vi "Position_TOTAL_R25.vi"(5 "Distance Between \nCameras  (*unit)":sgl=2.25) -> (12 "dX, dY\nLeft Cam":cluster{"X":sgl[], "Y":sgl[]}={"X"=[-1.0065897, 0.099401906, 1.1628555, 2.2500029, 0.0], "Y"=[10.716516, 10.801518, 10.883252, 10.9668045, 0.0]}, 13 "Position Valid":bool=TRUE, 14 "Left Camera Real Coordinates":cluster{"X":sgl, "Y":sgl}={"X"=10.842023, "Y"=1.3735824}, 16 "dX, dY\nRight Cam":cluster{"X":sgl[], "Y":sgl[]}={"X"=[-2.8840373, -1.7780458, -0.7145921, 0.3725553, -1.8774476], "Y"=[9.387911, 9.472914, 9.554648, 9.638201, -1.3286046]}, 18 "Robot Coordinates":cluster{"X":sgl, "Y":sgl}={"X"=10.17772, "Y"=2.3123062}, 19 "Orietnation\n(current)":sgl=-30.94054 format="%#_13g")   [LabVIEW 2015]
uses:
  <vilib>/Analysis/coordinate.llb/2D Cartesian Coordinate Rotation (Array).vi
  <vilib>/myRIO/Common/Instrument Driver Framework/myRIO v1.0/DIO/vis/myRIO v1.0 Close DIO.vi
  <vilib>/myRIO/Common/Instrument Driver Framework/myRIO v1.0/DIO/vis/myRIO v1.0 Unreserve DIO.vi
  <vilib>/myRIO/Common/Instrument Driver Framework/myRIO v1.0/DIO/vis/myRIO v1.0 Build MUX Configuration DIO.vi
  <vilib>/myRIO/Common/Instrument Driver Framework/myRIO v1.0/Resource Manager/vis/myRIO v1.0 Unreserve Channel List.vi
  <vilib>/myRIO/Common/Instrument Driver Framework/myRIO v1.0/Resource Manager/vis/myRIO v1.0 Create Configuration List.vi
  <vilib>/myRIO/Common/Instrument Driver Framework/myRIO v1.0/Resource Manager/vis/myRIO v1.0 Unreserve Channel.vi
  <vilib>/myRIO/Common/Instrument Driver Framework/myRIO v1.0/Resource Manager/vis/myRIO v1.0 Build Mutex Name.vi
  <vilib>/Instr/_visa.llb/VISA Configure Serial Port (Instr).vi
  <vilib>/myRIO/Common/Instrument Driver Framework/myRIO v1.0/DIO/vis/myRIO v1.0 Shutdown DIO.vi
  <vilib>/Utility/error.llb/Error Cluster From Error Code.vi
  <vilib>/myRIO/Common/Instrument Driver Framework/myRIO v1.0/Resource Manager/vis/myRIO v1.0 Configure IO.vi
  <vilib>/myRIO/Common/Instrument Driver Framework/Utilities/vis/Configuration Manager.vi
  <vilib>/myRIO/Common/Instrument Driver Framework/Utilities/vis/IO Manager.vi
  <vilib>/myRIO/Common/Instrument Driver Framework/myRIO v1.0/myRIO v1.0 Close.vi
  <vilib>/Analysis/NI_AALPro.lvlib
  <vilib>/myRIO/Instrument Drivers/Onboard IO/DIO/DIO.lvlib
panel:
  out "Current Template - Right":T1(ring)
  out "Current Template - Left":T1(ring)
  in  "Tab Control 2":T2(tab)
  out "Beacon Coordinates - Right Image":T3={"Beacon Position - X px"=[88.975365, 121.85722, 157.60713, 192.74931, 229.82234], "Beacon Position - Y px"=[106.21975, 102.49595, 103.61968, 103.22959, 103.920715]}
  out "Beacon Coordinates - Left Image":T3={"Beacon Position - X px"=[96.57839, 127.0317, 159.93825, 190.94315, 221.86247], "Beacon Position - Y px"=[111.67795, 107.306076, 106.92789, 105.73433, 104.09002]}
  in  "Image Width (px)":sgl=320.0
  in  "Image Height (px)":sgl=240.0
  in  "Cam AOV Horizontal (deg)":sgl=58.0
  in  "Cam AOV Vertical (deg)":sgl=45.0
  out "Angle to Pixel Ratios":T4={"Angle to Pixel\nRatio - Horizontal"=0.18125, "Angle to Pixel\nRatio - Vertical"=0.1875} {"Angle to Pixel\nRatio - Vertical" format="%#_13g"; "Angle to Pixel\nRatio - Horizontal" format="%#_13g"}
  in  "Num of Beacons (Total)":i8=5
  out "Left Data\nInput Flag\n- Internal":bool
  out "Right Data\nInput Flag\n- Internal":bool
  out "This Servo \nAngle - Left":sgl=52.96875
  in  "Valid Angles - L":bool[](array[boolean])=[TRUE, TRUE, TRUE, TRUE, TRUE]
  in  "Valid Angles -R":bool[](array[boolean])=[TRUE, TRUE, TRUE, TRUE, TRUE]
  in  "Beacon Angles - L":sgl[](array[numeric])=[64.19745, 58.642975, 52.682835, 47.05908, 41.446476]
  in  "Beacon Angles -R":sgl[](array[numeric])=[71.43643, 65.46979, 58.9926, 52.62266, 45.904842]
  out "This Servo \nAngle - Right":sgl=58.76953
  in  "Position Calc\nReady":bool=TRUE
  out "Array":sgl[](array[numeric])=[9.555056, 8.575206, 8.036942, 7.810829, 6.6351933]
  out "Array 2":sgl[](array[numeric])=[5.5039287, 6.210328, 7.1312, 8.266513, 8.73579]
  out "Array 3":sgl[](array[numeric])=[3.2039287, 3.9103284, 4.8311996, 5.9665127, 6.4357905]
  in  "stop":bool
  in  "Servo Algorithm\nCycle Time(ms)":i32=25
  in  "Move Servo\nThreshold (deg)":sgl=2.0 format="%#_13g"
  in  "SERVO ENABLE":bool
  in  "Max Write\nTx Attempts":u8=3
  in  "Max Read\nTx Attempts":u8=3
  in  "close comms":bool
  in  "Servo Comm\nLoop Time (ms)":i32=20
  out "dT - Comm Loop":u32=21
  in  "Left Servo\nID":string="\u0000"
  in  "Servo Comm\nWait Time - (ms)":i32
  in  "Right Servo\nID":string="\u0001"
  in  "Search Step Size\n(deg)":sgl=15.0 format="%#_13g"
  out "Last Orientation":sgl=-35.285717
  out "Last Position":cluster{"X":sgl, "Y":sgl}={"X"=10.147585, "Y"=2.64441}
  in  "Compliance Slope":u8=128
  in  "Search Step Size":u16=50
  in  "Mounting Offset - Left":sgl=-45.0
  in  "Minimum Delta \nServo Threshold":i16=3
  in  "Maximum Move \nServo Threshold":i16=300
  in  "Wait Tick Threshold":i32=10
  in  "Min Num Frames\nper Search":i32=3
  in  "Middle Beacon\nCoordinates":cluster{"X":sgl, "Y":sgl}={"X"=0.0, "Y"=2.5}
  in  "Max Recovery\nSearch Attempts":u16=3
  in  "Max Recovery Count\n(Recovery Search)":u16=20
  in  "Mounting Offset - Right":sgl=45.0
  in  "Tracking Timeout\nThreshold":i32=10
  in  "Timeout to \nEnable Reactive Predict":u16=3
  out "Beacon Scales - Right":sgl[](array[numeric])=[50.81787, 54.150085, 54.01553, 51.723366, 54.605507]
  out "Beacon Scales - Left":sgl[](array[numeric])=[46.59789, 48.180458, 47.842606, 46.504417, 45.297752]
  in  "Recovery Parallel\nSearch Offset":u16=50
  in  "Max # Pan Moves":u16=3
  in  "Current Angle\n - Right (internal)":sgl=58.76953
  in  "Current Angle\n - Left (internal)":sgl=52.96875
  in  "Servo Goal Position\n - Left":u16=360
  in  "Servo Goal Position\n - Right":u16=670
  out "Move Servo - R":bool
  out "Move Servo - L":bool
  out "Current L (10bit)":u16=232
  out "Servo Moving - L":bool
  out "Servo Moving - R":bool
  out "Current R (10bit)":u16=559
  out "deltaMoveServo\n- L":i16
  out "Move Respond - L":bool
  out "Move Respond - R":bool
  out "deltaMoveServo\n- R":i16
  out "Current Main State - Left":T5(ring)=enum."Tracking"
  in  "Initial Main State - Left":T5(ring)
  in  "Image Lock - Left":bool=TRUE
  in  "Track Angle Valid - Left":bool=TRUE
  out "New Data  Flag\nLeft Servo":bool
  in  "Tracking Angle - Left":sgl=52.933372
  in  "Search Direction - in - L":bool
  out "Frames Processed\nCount - in -L":i32
  out "Recovery Mode Count - in Left":u16
  in  "Image Lock - Right":bool
  out "Recovery Search\nmove Count - in - L":u16
  out "Recovery Search\nAttempt Count - in - L":u16
  out "Current Move Delta - L":u16
  out "Next Main State - Left":T5(ring)=enum."Tracking"
  in  "Recovery Search\nDirection - L":bool=TRUE
  out "Last Track Angle - L":sgl=52.96875
  in  "Initial Main State- Right":T5(ring)
  out "Current Main State - Right":T5(ring)=enum."Tracking"
  in  "Track Angle Valid  - Right":bool
  out "New Data  Flag\nRight Servo":bool
  in  "Tracking Angle - Right":sgl=58.953144
  out "Recovery Search\nAttempt Count - Right":u16
  out "Recovery Search\nmove Count - Right":u16
  out "Frames Processed\nCount - in Right":i32
  out "Recovery Mode Count in Right":i32
  in  "Recovery Search\nDirection - R":bool
  out "Next Main State - Right":T5(ring)=enum."Tracking"
  in  "Search Direction - in - Right":bool=TRUE
  out "Tracking Timeout\nCount - L":i32
  out "Tracking Timeout\nCount - R":i32
  out "Current Tracking State - Left":enum16{"Track", "Reactive Predict", ""}(ring)
  in  "Initial Tracking State - Left":enum16{"Track", "Reactive Predict", ""}(ring)
  out "Next Tracking State - Left":enum16{"Track", "Reactive Predict", ""}(ring)
  in  "Initial Tracking State - Right":enum16{"Track", "Reactive Predict", ""}(ring)
  out "Current Tracking State - Right 2":enum16{"Track", "Reactive Predict", ""}(ring)
  out "Next Tracking State - Right":enum16{"Track", "Reactive Predict", ""}(ring)
  in  "Initial Recovery State - L":enum16{"Generic Sweep", "Recovery Search"}(ring)=enum."Recovery Search"
  in  "Initial Recovery State  - Right":enum16{"Generic Sweep", "Recovery Search"}(ring)=enum."Recovery Search"
  out "Current Recovery State - Right":enum16{"Generic Sweep", "Recovery Search"}(ring)=enum."Recovery Search"
  out "Next Recovery State - Right":enum16{"Generic Sweep", "Recovery Search"}(ring)=enum."Recovery Search"
  out "Next Recovery State - Left":enum16{"Generic Sweep", "Recovery Search"}(ring)=enum."Recovery Search"
  out "Current Recovery State -L":enum16{"Generic Sweep", "Recovery Search"}(ring)=enum."Recovery Search"
  out "Current Move Delta - R":u16
  in  "Mining Alignment\nEnabled":bool
  in  "Real Beacon\n - Coordinates":cluster{"X":dbl[], "Y":dbl[]}={"X"=[0.0, 0.0, 0.0, 0.0, 0.0, 0.0], "Y"=[0.5, 1.5, 2.5, 3.5, 4.5, 0.0]}
  out "LOCAL\nBeacon Coordinates\nRelative to Robot":cluster{"dX_beacon":sgl[], "dY_beacon":sgl[]}={"dX_beacon"=[5.5039287, 6.210328, 7.1312, 8.266513, 8.73579], "dY_beacon"=[9.555056, 8.575206, 8.036942, 7.810829, 6.6351933]}
  out "Local Coordinates - Calculated":cluster{sgl[], sgl[]}(graph)={[5.5039287, 6.210328, 7.1312, 8.266513, 8.73579], [9.555056, 8.575206, 8.036942, 7.810829, 6.6351933]}
  out "Distance to LBF":sgl[](array[numeric])=[0.024284193, 0.015691843, 0.008273765, 0.028971607, 0.03291407]
  out "Right Camera Real Coordinate":cluster{"X":sgl, "Y":sgl}={"X"=9.513418, "Y"=3.25103}
  out "Post Filtering\n- Valid Beacons":bool[](array[boolean])=[TRUE, TRUE, TRUE, TRUE, FALSE]
  in  "Distance\nBetween Beacons":sgl=1.0 format="%#_13g"
  in  "Distance\nBetween Beacons \n- Tolerance":sgl=0.5 format="%#_13g"
  in  "Distance Threshold\nRef Triangles (*unit)":sgl=30.0
  out "All Object Coordinates \n- Local":cluster{"X":sgl[], "Y":sgl[]}={"X"=[2.3, 5.368779, 6.320682, 7.235974, 8.171657, 0.0], "Y"=[0.0, 9.329155, 8.759661, 8.21207, 7.6522775, 0.0]}
  out "Local Coordinates - Normalized":cluster{sgl[], dbl[]}(graph)={[2.3, 5.368779, 6.320682, 7.235974, 8.171657, 0.0], [0.0, 9.329154968261719, 8.759660720825195, 8.21207046508789, 7.65227746963501, 0.0]}
  out "All Object Coordinates \n- Local - Rotated":cluster{"X":sgl[], "Y":sgl[]}={"X"=[1.8774476, -1.0065897, 0.099401906, 1.1628555, 2.2500029, 0.0], "Y"=[1.3286046, 10.716516, 10.801518, 10.883252, 10.9668045, 0.0]}
  out "Local Coordinates - Rotated":cluster{dbl[], dbl[]}(graph)={[1.8774476489648846, -1.0065896210507148, 0.09940190570174412, 1.1628555490135675, 2.250002943734801, 0.0], [1.3286045709883498, 10.716515276262749, 10.801518262128845, 10.883252530212562, 10.966804865321656, 0.0]}
  out "Right_Flag 2":bool
  out "Beacons Found\n- Right (Bool Array)":bool[](array[boolean])=[TRUE, TRUE, TRUE, TRUE, TRUE]
  out "RIGHT Beacon Position - Y px (IN)":sgl[](array[numeric])=[106.21975, 102.49595, 103.61968, 103.22959, 103.920715]
  out "RIGHT Beacon Coord - X px (IN)":sgl[](array[numeric])=[88.975365, 121.85722, 157.60713, 192.74931, 229.82234]
  out "Left_Flag 2":bool
  out "Beacons Found\n- Left (Bool Array) 2":bool[](array[boolean])=[TRUE, TRUE, TRUE, TRUE, TRUE]
  out "LEFT Beacon Coord - X px (IN) 2":sgl[](array[numeric])=[96.57839, 127.0317, 159.93825, 190.94315, 221.86247]
  out "LEFT Beacon Position - Y px (IN) 2":sgl[](array[numeric])=[111.67795, 107.306076, 106.92789, 105.73433, 104.09002]
  in  "Fetch Input\n(mSec)":u32=20 caption="Update Camera Input\n(mSec)"
  in  "Max Std Dev (5)":sgl=0.1 format="%#_13g"
  out "Position \nLock Status":bool=TRUE
  out "Real Position in Course 2":cluster{"X":dbl[], "Y":dbl[]}(graph)={"X"=[10.147584990557128], "Y"=[2.644409845240164]}
  out "Robot Coordinates - Avgd":cluster{"X":sgl, "Y":sgl}={"X"=10.147585, "Y"=2.64441}
  in  "Max Std Dev (4)":sgl=0.1 format="%#_13g"
  in  "Max Std Dev (3)":sgl=0.2 format="%#_13g"
  in  "New Position\nWeight (X coord)":sgl=0.8 format="%#_13g"
  in  "Max X (arena)":sgl=35.0
  in  "Max Y (arena)":sgl=15.0
  in  "History Size":u8=15
  out "Orientation Avgd":sgl=-35.285717
  in  "New Position \nThreshold":sgl=2.0
  out "Robot Coordinates\nHistory":cluster{sgl, sgl}[](array[cluster])=[{10.147585, 2.64441}, {10.056327, 2.8351064}, {10.020484, 2.7815769}, {10.034186, 2.7172103}, {0.0, 0.0}, {10.036168, 2.7859242}, {9.938812, 2.8961887}, {10.1160965, 2.6632404}, {10.016709, 2.7454932}, {10.037537, 2.8544023}, {10.017025, 2.7817721}, {9.997087, 2.8064857}, {10.065648, 2.6537364}, {10.084976, 2.6750228}, {10.082739, 2.688601}]
  out "Orientation\nHistory":sgl[](array[numeric])=[-35.285717, -36.86449, -36.153664, -35.44657, 0.0, -37.6105, -36.02637, -35.82032, -36.08894, -37.01076, -36.293255, -36.40525, -35.738438, -35.683483, -35.770218]
  out "Position Valid\nHistory":bool[](array[boolean])=[TRUE, TRUE, TRUE, TRUE, FALSE, TRUE, TRUE, TRUE, TRUE, TRUE, TRUE, TRUE, TRUE, TRUE, TRUE]
  in  "Moving Average\nWindow Length":u8=10
  in  "New Orientation \nThreshold":sgl=10.0
  in  "Triangle Based\nWeight":sgl format="%#_13g"
  out "Scale Based\nWeight":sgl=1.0 format="%#_13g"
  out "New Position\nWeight (Y coord)":sgl=0.3 format="%#_13g"
  out "New Orientation\nWeight":sgl=0.2
  out "dT":dbl=144.111
  in  "Position Calc\nTimer":u32=100 caption="Position Calc Timer"
  out "inches":dbl
  out "dA2 3":sgl=44.126 format="%#_13g"
  out "Valid Beacon Sets_":bool[](array[boolean])=[TRUE, TRUE, TRUE, TRUE, TRUE]
  in  "Check Shared Var Timer":u32=50 caption="Main Loop\n Timer (ms)"
  out "dA2 2":sgl=48.543114 format="%#_13g"
  out "dA2 4":sgl=48.543114 format="%#_13g"
  out "Last Track Angle - R":sgl=59.941406
  in  "Recovery Search\nDirection - L 2":bool
  in  "Max Recovery Count\n(Recovery Search) 2":u16
  in  "Max Recovery\nSearch Attempts 2":u16
  in  "Image Lock - Right 2":bool
  # "SETTINGS"
  # "IMAGE TO ANGLE VARIABLES"
  # "INPUTS"
  # "OUTPUT VALUES"
  # "CONFIG"
  # "SERVO CONTROL VARIABLES"
  # "SERVO CONTROL VARIABLES"
  # "CONFIG"
  # "SHARED VARIABLE INPUTS"
  # "LOCAL VARIABLE INPUTS"
  # "INTERNRAL VARIABLES"
  # "MISC"
  # "SERVO IDs"
  # "CONTROL DELAYS"
  # "COMM LOOP DELAY"
  # "COMM PROTOCOL"
  # "Make function of distance^^"
  # "LEFT SERVO"
  # "RIGHT SERVO"
  # "Main State Machine"
  # "Recovery State Machine"
  # "Current Track Angle Inputs"
  # "Servo Status Inputs"
  # "Main State Machine Inputs"
  # "Recovery State Machine Inputs"
  # "Current Track Angle Inputs"
  # "Servo Status Inputs"
  # "Tracking State Machine Inputs"
  # "Tracking State Machine Inputs"
  # "POSITION CALCULATION VARIABLES"
  # "OUTPUT VALUES"
  # "CONFIG VALUES"
  # "FILTER CONFIG VALUES"
  # "FEEDBACK INPUT VALUES"
  # "INPUT VALUES"
  # "INTERMEDIATE VALUES"
  # "Use moving average for previous orientation thresholds"
  # "*********************"
  # "unfiltered"
  # "Inter Beacon Distance Filtering"
  # "NOTE: Must be 1 bigger than amount of beacons"
  # "NOTE: Must be 1 bigger than amount of beacons"
  # "VISION PROCESSEING INPUTS"
  # "update to coordinate outlier filtering R2"
  # "NEW FILTER VALS"
  # "MOVING AVERAGE\nVARIABLES"
  # "DISTANCE SOURCE WEIGHT"
  # "*****  I made this 0\n         bc it seems to be \n        more stable"
  # "Recovery State Machine Feedback"
  # "SEARCH ROUTINE VARIABLES"
types:
  T1 = enum16{"Range 1", "Range 2", "Range 3", "Range 0"}
  T2 = enum32{"image to angle ", "Empty", "servo control - Config", "left and right servo - Status", "Position Calc - Debug Data", "Position Calc - Debug Data 2", "Vision Processing INputs", "ROBOT POSITION", "Random"}
  T3 = cluster{"Beacon Position - X px":sgl[], "Beacon Position - Y px":sgl[]}
  T4 = cluster{"Angle to Pixel\nRatio - Horizontal":sgl, "Angle to Pixel\nRatio - Vertical":sgl}
  T5 = enum16{"Start Up Search", "Tracking", "Recovery Mode", ""}
  T6 = cluster{"Lock":bool, "Current Valid":bool, "Current Template":enum16{"Range 1", "Range 2", "Range 3", "Range 0"}, "Tracking Coordinates":cluster{"X":dbl, "Y":dbl}, "Setting Values":cluster{"Min Score":dbl, "Min Scale":dbl, "Max Scale":dbl, "Curve Parameters":cluster{"Min Length":i32, "Row Search Step":i32, "Col Search Step":i32}}}
  T7 = cluster{"Array of Double":dbl[], "Array of Double":dbl[]}
  T8 = enum16{"Sub - 2", "Sub - 3", "Sub - 4", "Normal - 5"}
  T9 = typedef "DIO.lvlib/DIO Reference.ctl" = cluster{"myRIO Reference":T10, "DIO Channels List":T14}
  T10 = typedef "myRIO Generic Hardware Reference.ctl" = cluster{"myRIO Model":T11, "myRIO Hardware Reference":T12}
  T11 = typedef "Hardware Version Enum.ctl" = enum16{"Unknown", "myRIO-1900", "myRIO-1950", "roboRIO"}
  T12 = typedef "myRIO v1.0 Reference.ctl" = cluster{"Generic FPGA Reference":T13, "Allow multiple opens":bool}
  T13 = typedef "Generic FPGA Reference.ctl" = refnum<k20>
  T14 = typedef "DIO Channels List.ctl" = T15[]
  T15 = typedef "DIO Channels Enum.ctl" = enum16{"Not Connected", "C/DIO0", "C/DIO1", "C/DIO2", "C/DIO3", "C/DIO4", "C/DIO5", "C/DIO6", "C/DIO7", "A/DIO0", "A/DIO1", "A/DIO2", "A/DIO3", "A/DIO4", "A/DIO5", "A/DIO6", "A/DIO7", "A/DIO8", "A/DIO9", "A/DIO10", "A/DIO11", "A/DIO12", "A/DIO13", "A/DIO14", "A/DIO15", "B/DIO0", "B/DIO1", "B/DIO2", "B/DIO3", "B/DIO4", "B/DIO5", "B/DIO6", "B/DIO7", "B/DIO8", "B/DIO9", "B/DIO10", "B/DIO11", "B/DIO12", "B/DIO13", "B/DIO14", "B/DIO15", "LED0", "LED1", "LED2", "LED3", "Button0", "DIO/DIO0", "DIO/DIO1", "DIO/DIO2", "DIO/DIO3", "DIO/DIO4", "DIO/DIO5", "DIO/DIO6", "DIO/DIO7", "DIO/DIO8", "DIO/DIO9", "SPI/CS0", "SPI/CS1", "SPI/CS2", "SPI/CS3", "LED RADIO (Green)", "LED RADIO (Red)", "LED COMM (Green)", "LED COMM (Red)", "LED MODE (Green)", "LED MODE (Red)"}
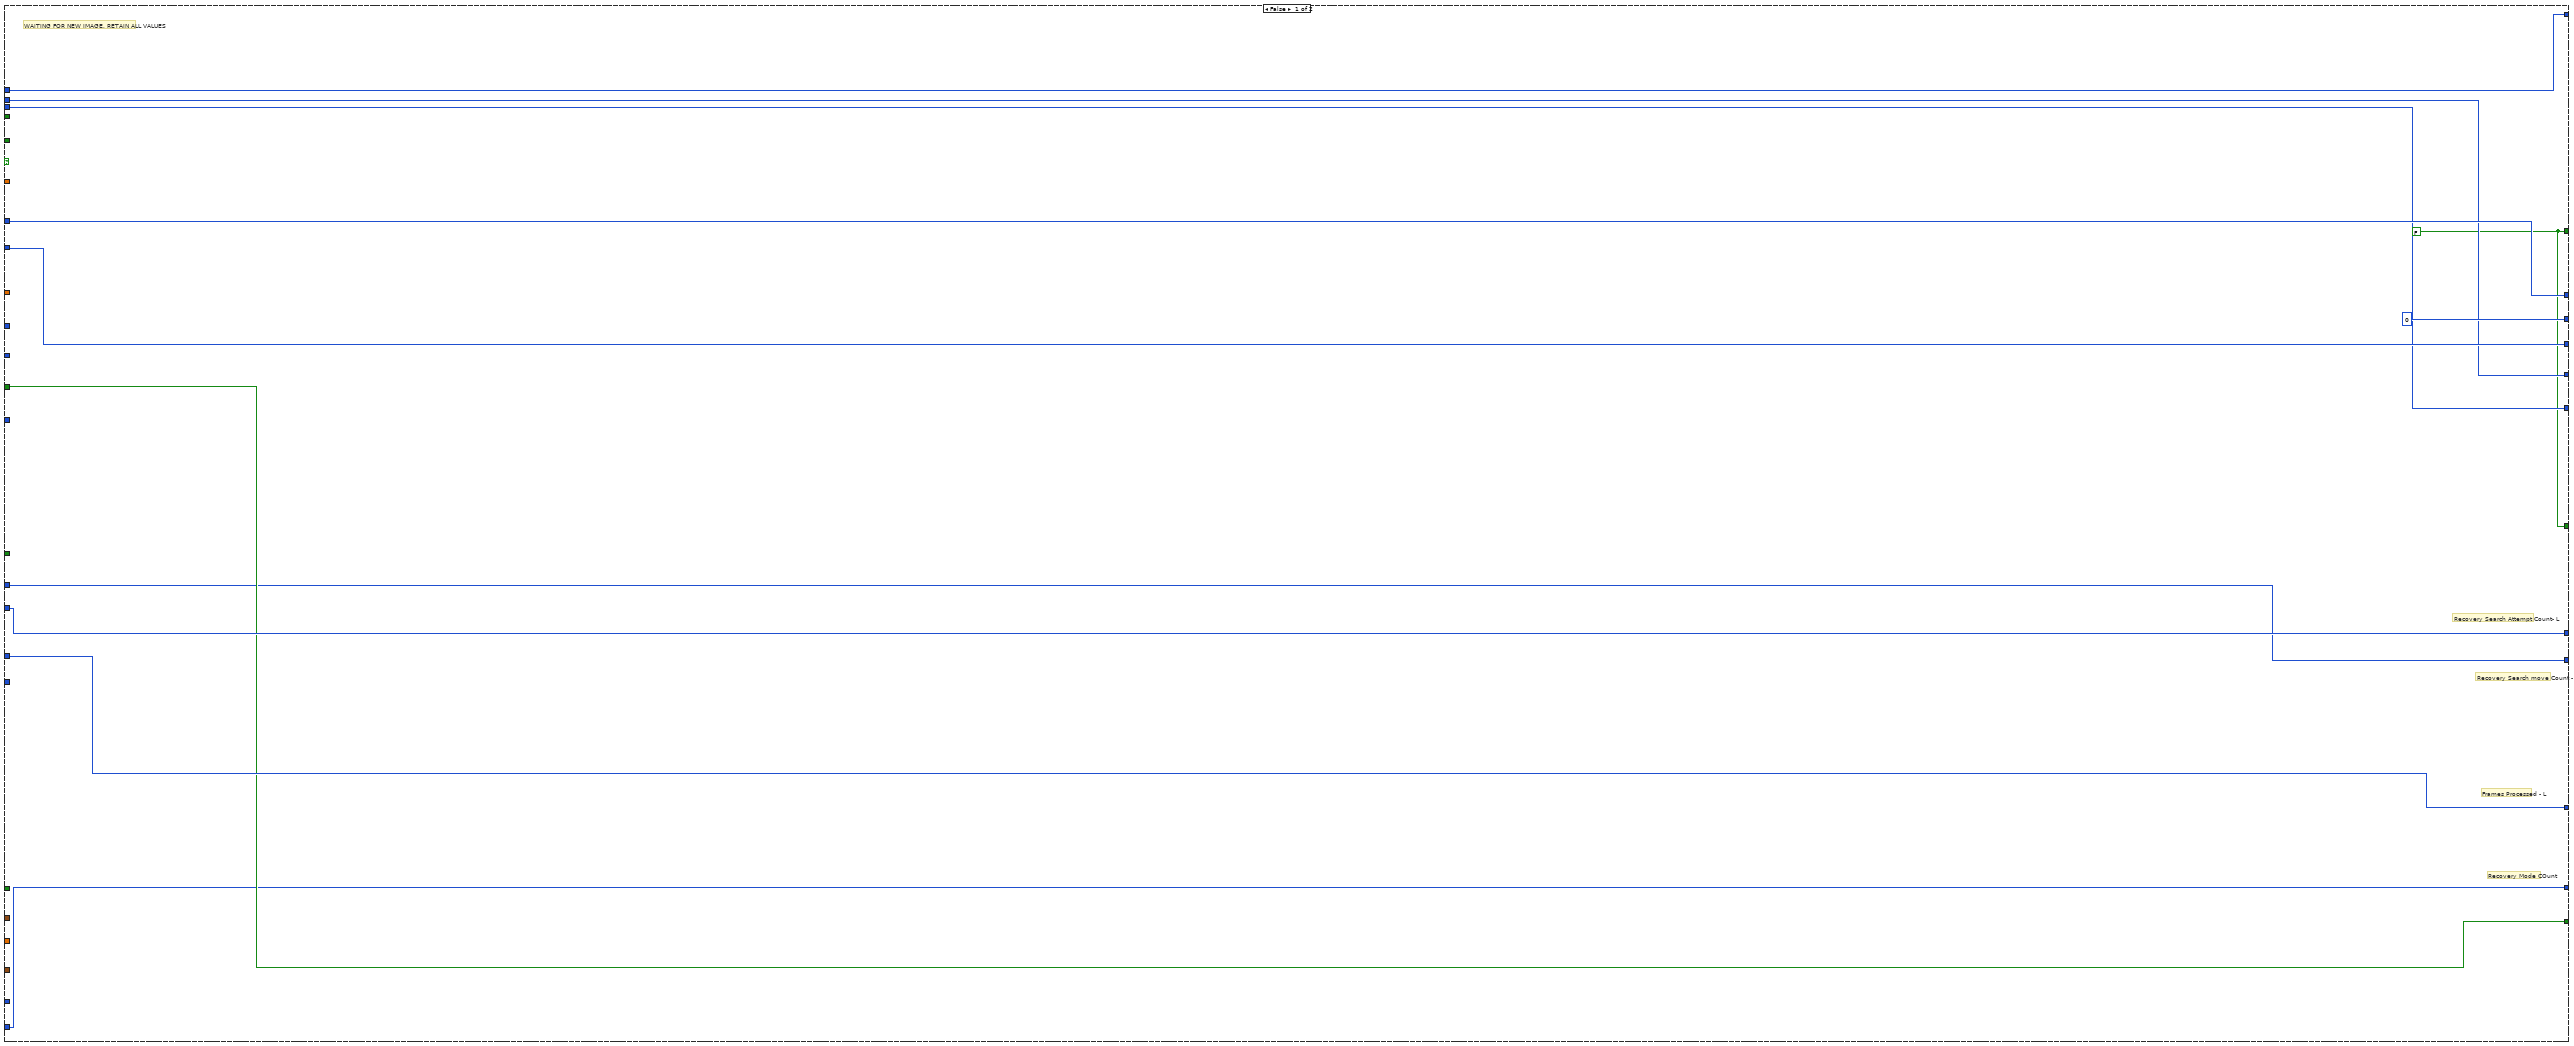
[diagram p2: hidden frame]
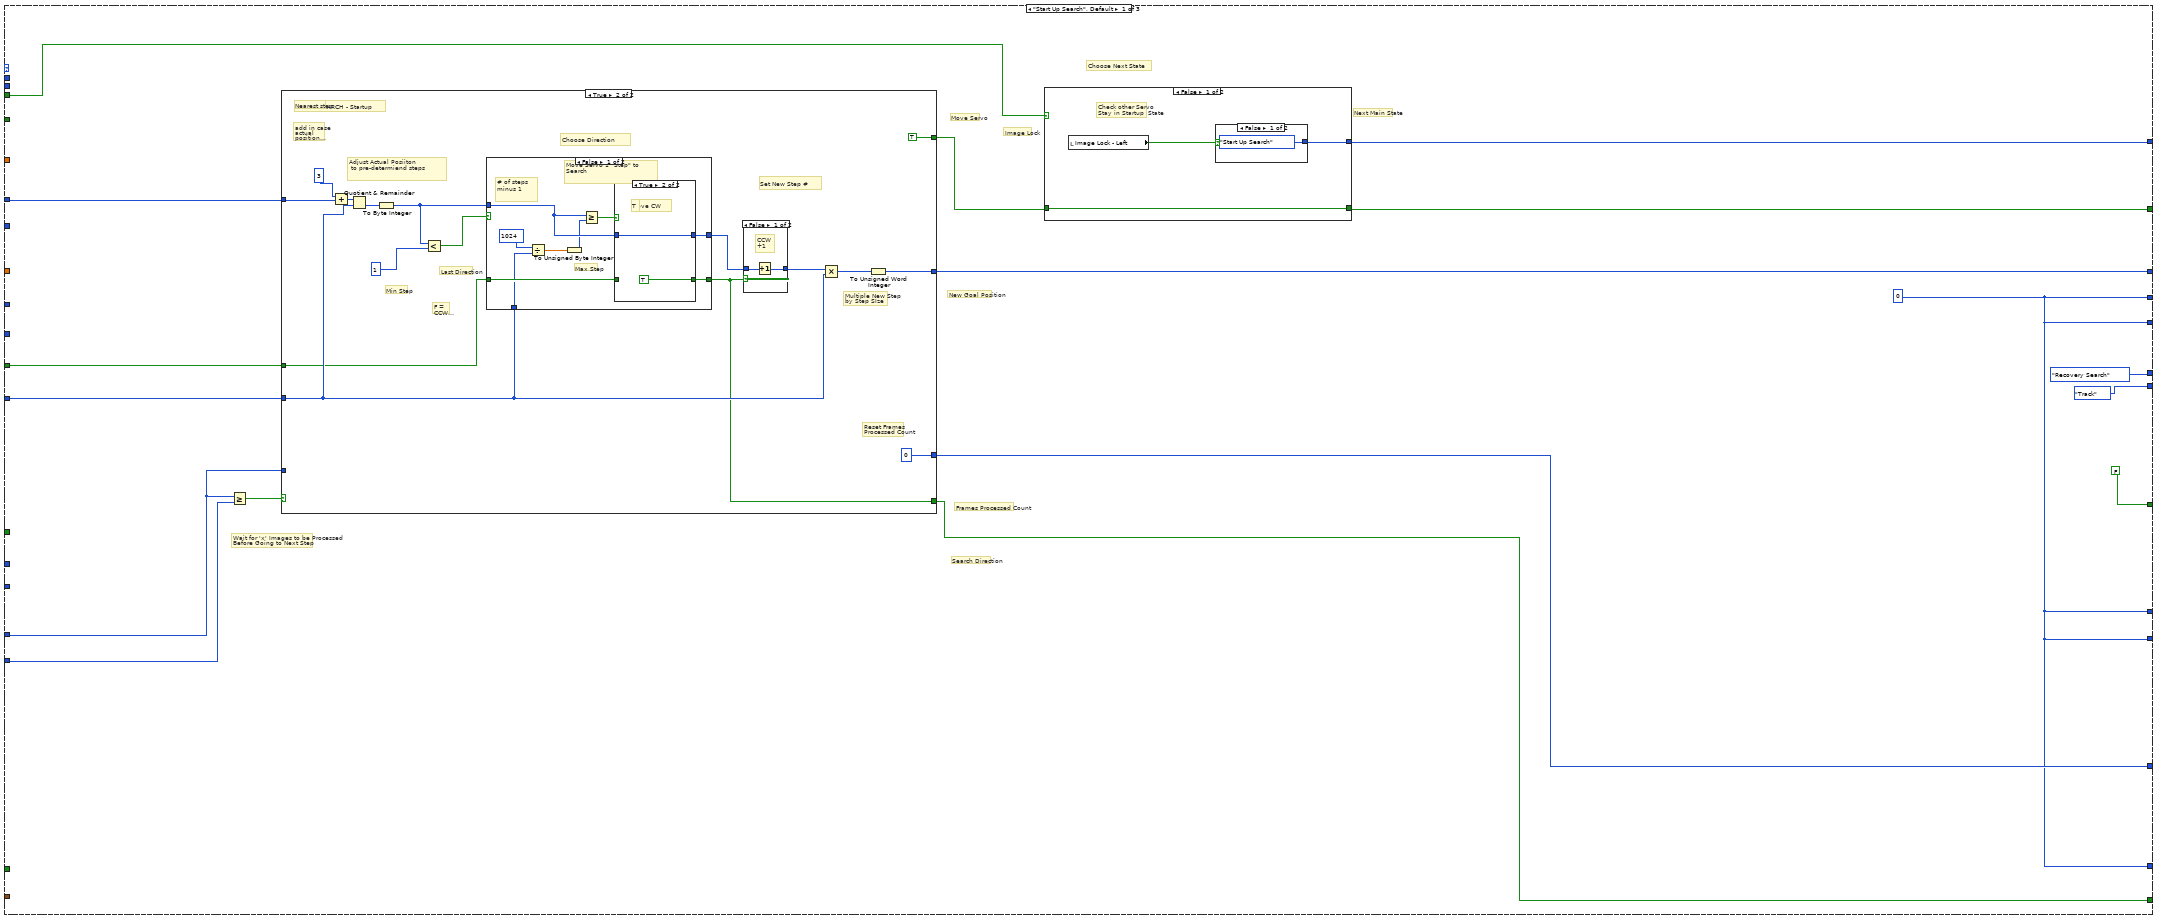
[diagram p3: hidden frame]
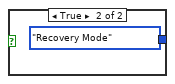
[diagram p4: hidden frame]
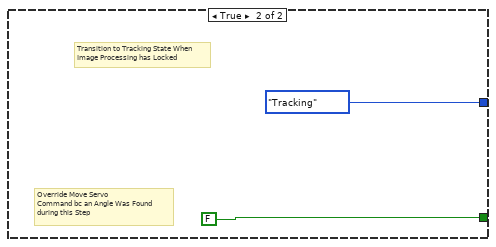
[diagram p5: hidden frame]
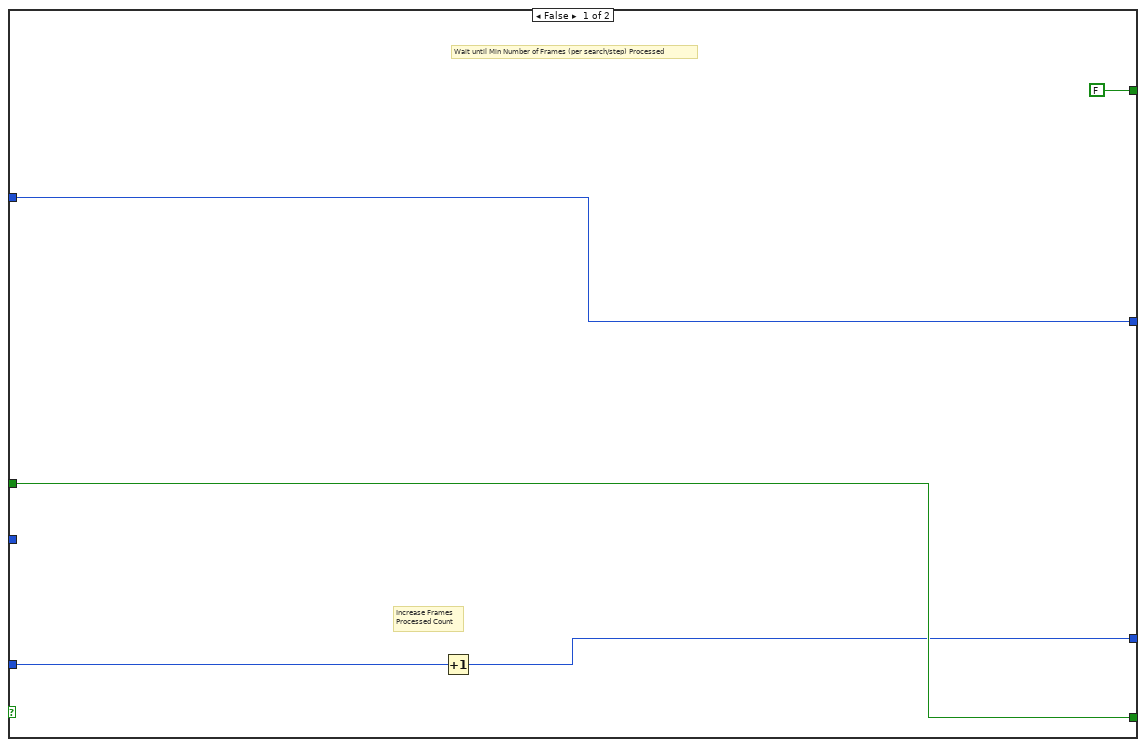
[diagram p6: hidden frame]
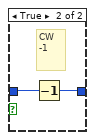
[diagram p7: hidden frame]
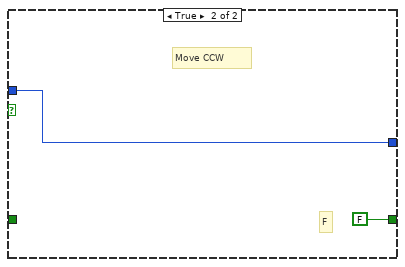
[diagram p9: hidden frame]
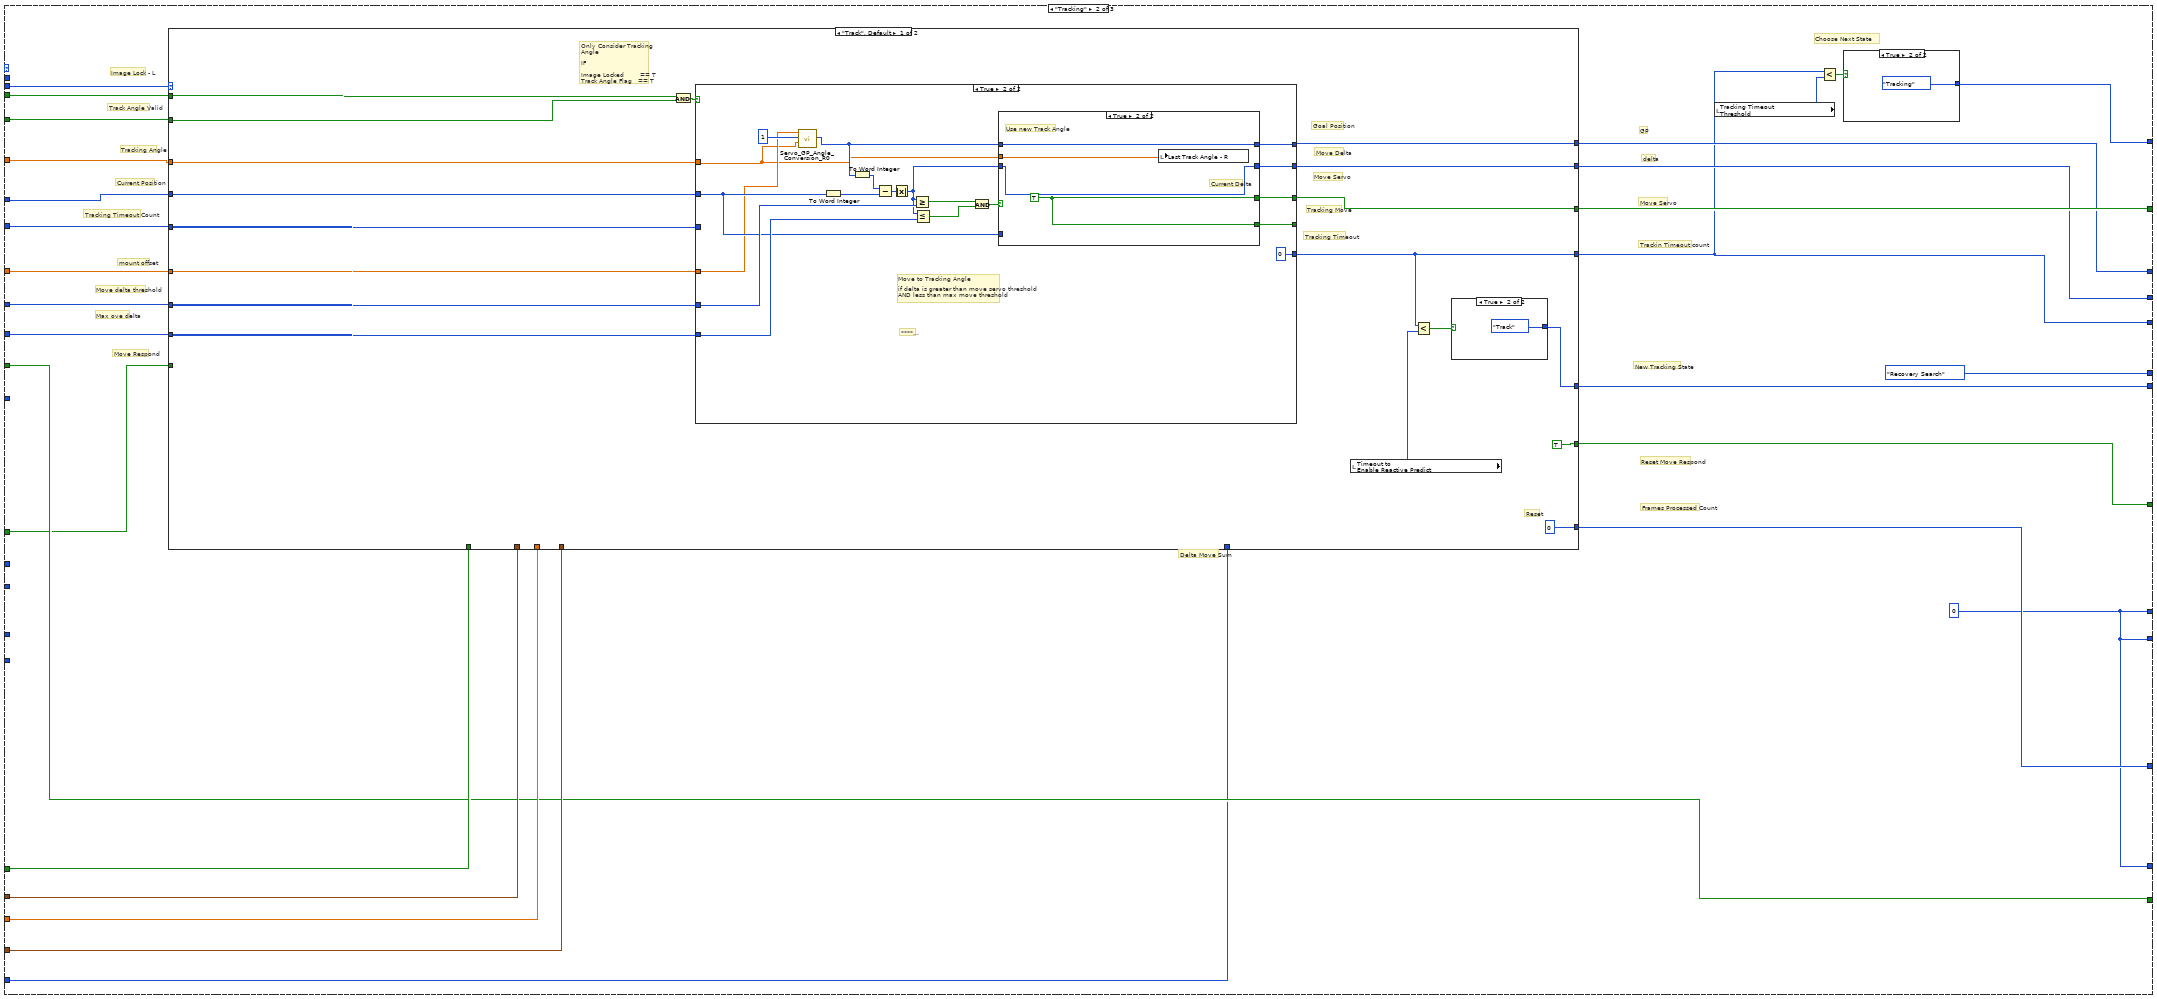
[diagram p10: hidden frame]
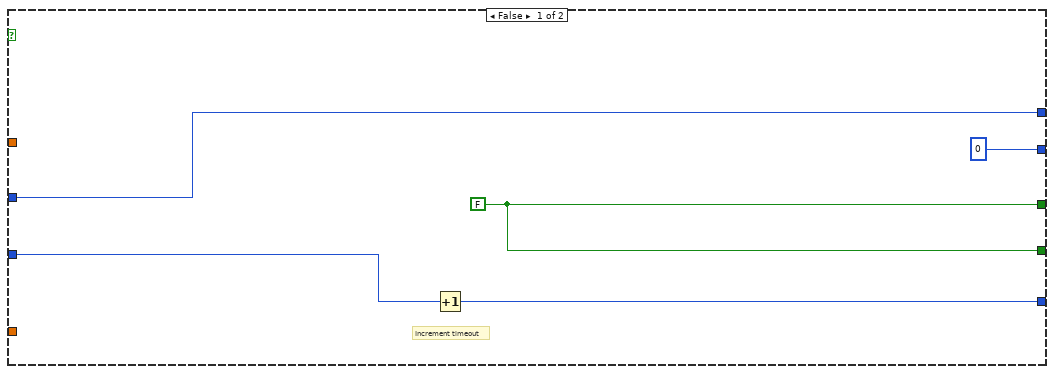
[diagram p11: hidden frame]
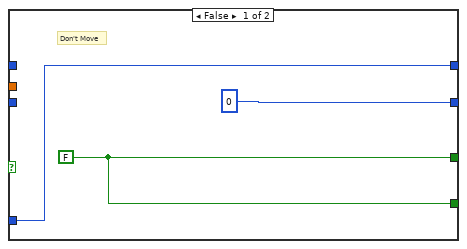
[diagram p12: hidden frame]
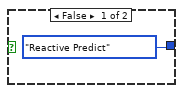
[diagram p13: hidden frame]
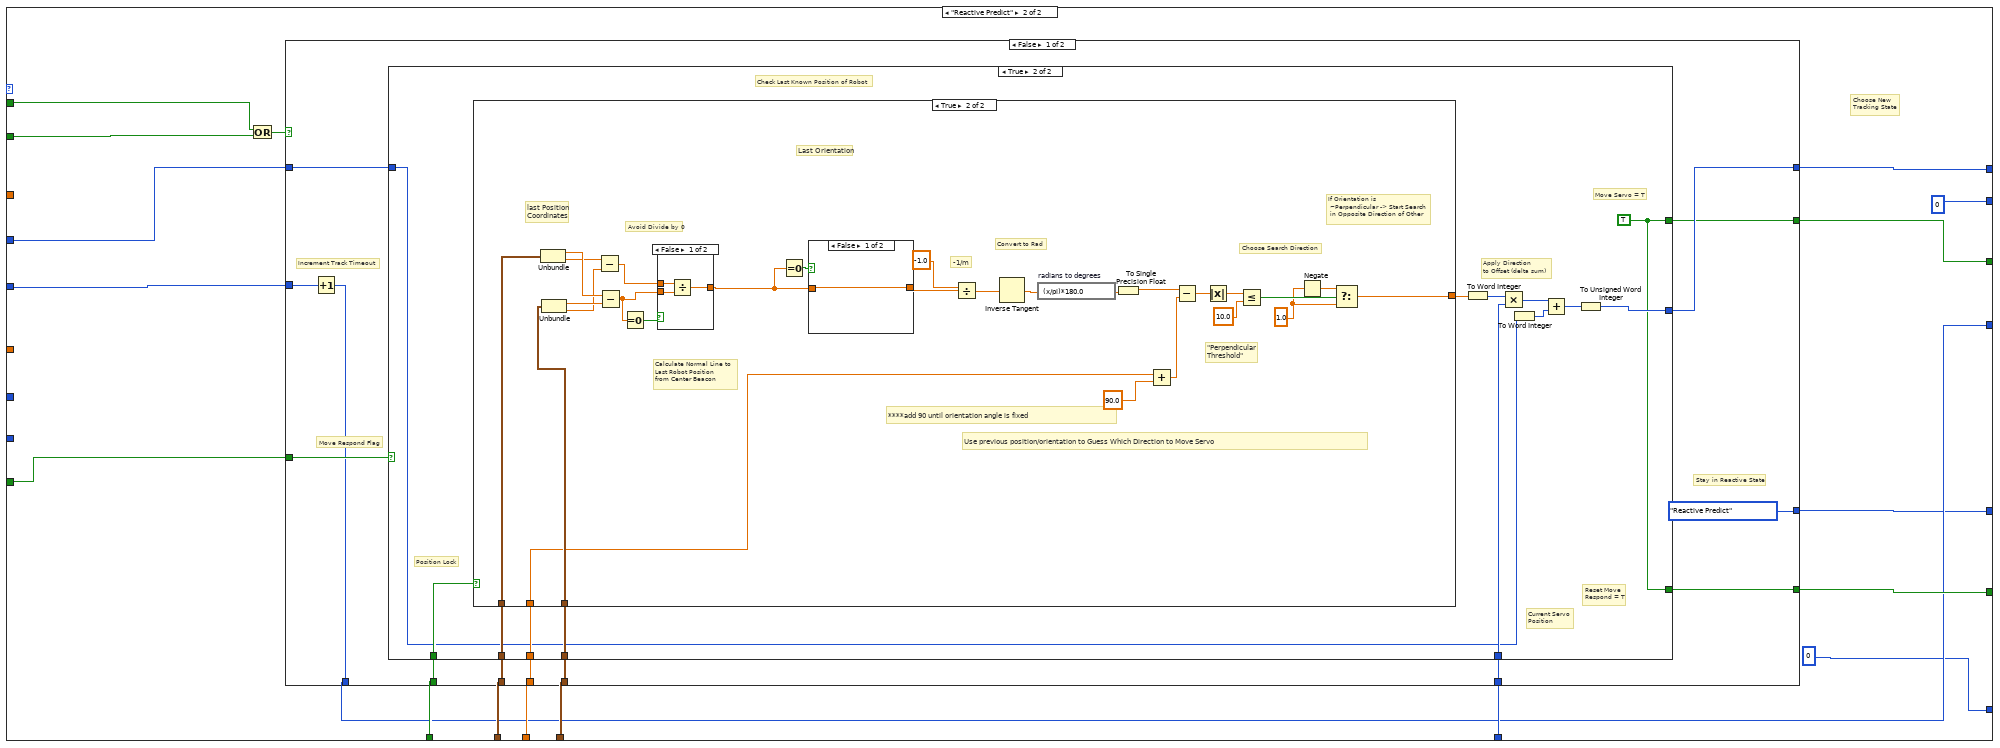
[diagram p14: hidden frame]
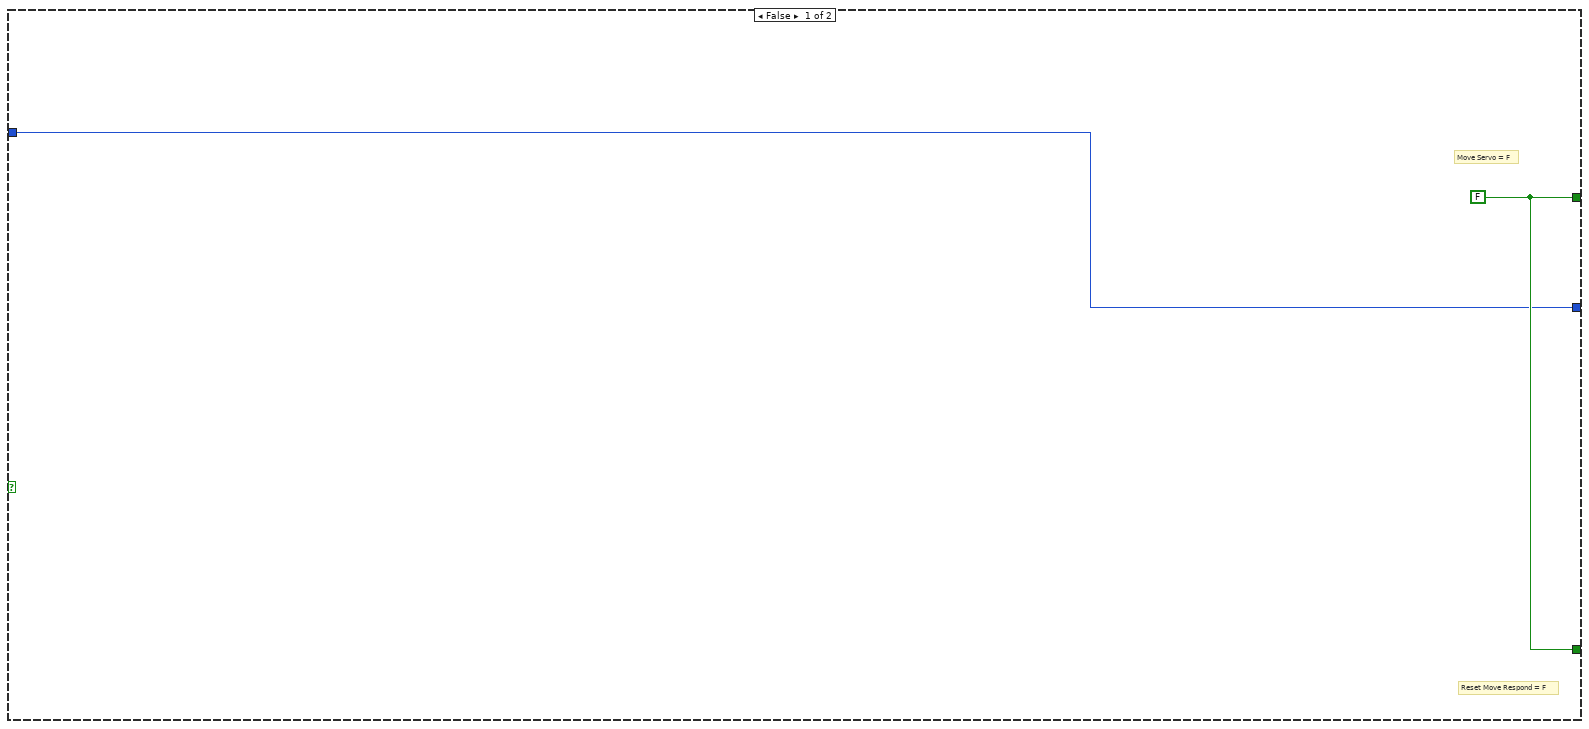
[diagram p15: hidden frame]
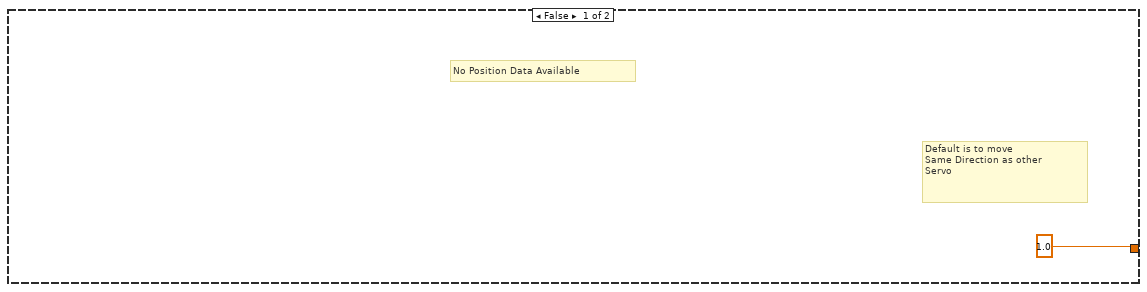
[diagram p16: hidden frame]
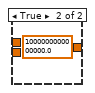
[diagram p17: hidden frame]
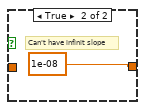
[diagram p18: hidden frame]
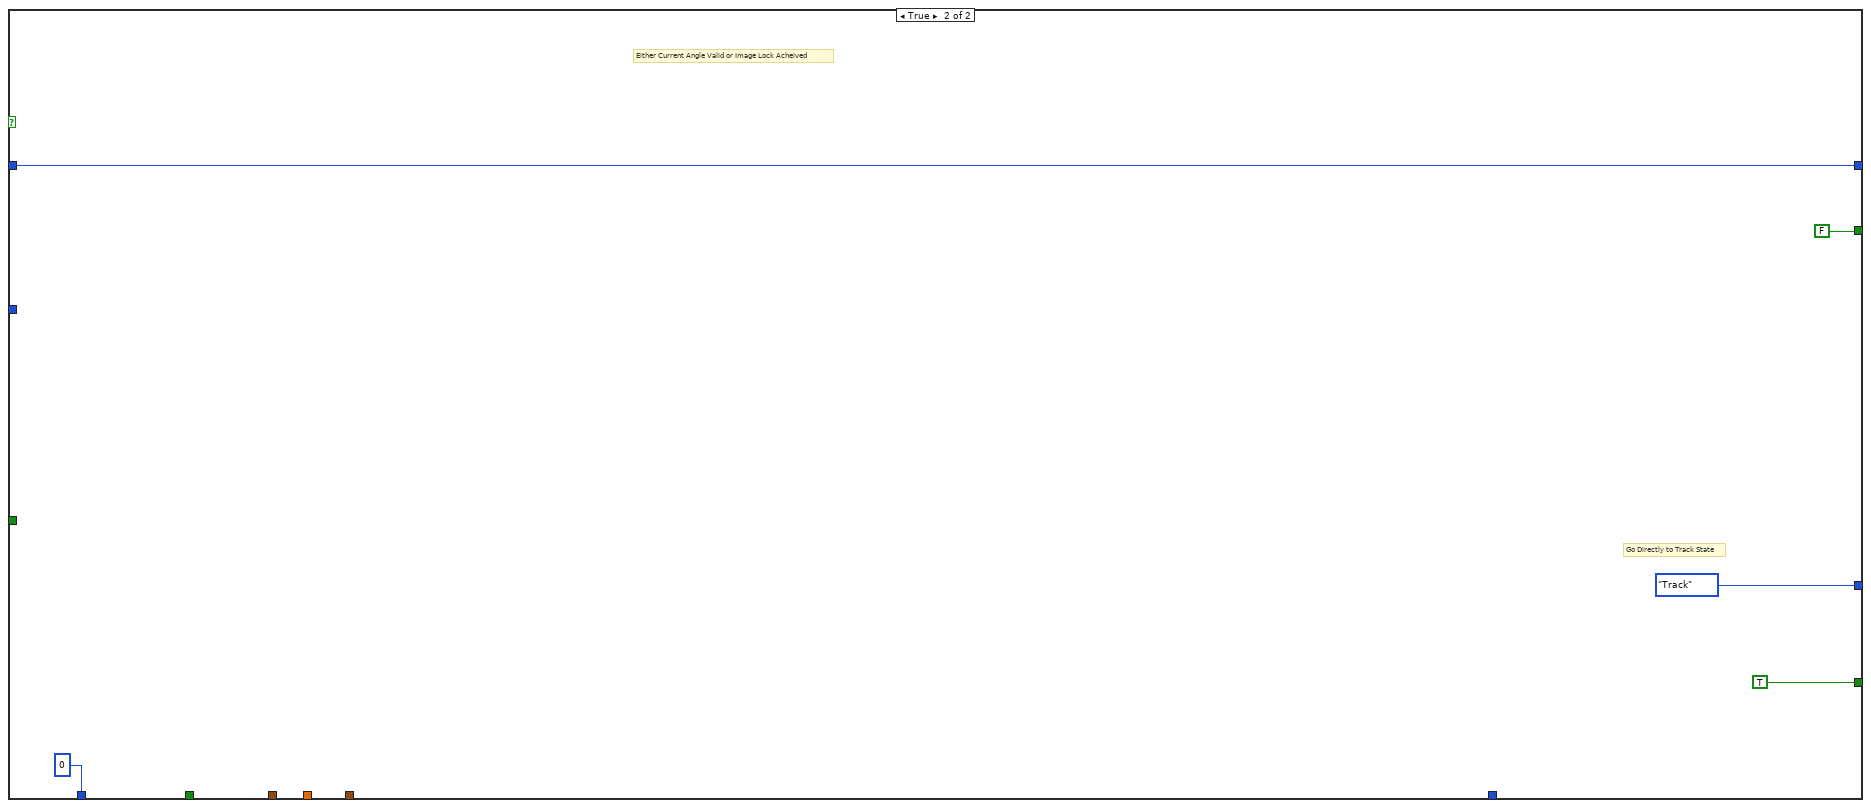
[diagram p19: hidden frame]
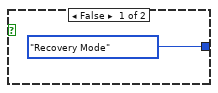
[diagram p20: hidden frame]
diagram:
  (unwired) enum16{"Generic Sweep", "Recovery Search"}."Recovery Search"
  w12 = 0 ("Frames Processed\nCount - in")
  w13 = 0 ("Frames Processed\nCount - in")
  w2 = FALSE
  w34 = sgl 0.0
  # "SERVO CONTROL FLAGS"
  # "***"
  # "Next Tracking State"
  # "Tracking Timeout Count"
  # "Search Direction - L"
  # "Next Recovery State"
  # "Move Respond"
  # "Recovery Mode Count - L"
  # "Delta Move Sum - L"
  # "Wait Tick Count - L"
  # "Frames Processed - L"
  # "Recovery Search move Count - L"
  # "Recovery Search Attempt Count- L"
  # "Next Main State"
  # "Search Direction - L"
  # "Next Recovery State"
  # "INPUTS - Local vars"
  # "Recovery Mode Count - L"
  # "Delta Move Sum - L"
  # "Frames Processed\nLeft"
  # "Move Respond - R"
  # "Initial Search Direction\n- Right"
  # "Move Respond"
  # "Recovery Mode Count - L"
  # "Delta Move Sum - L"
  # "Wait Tick Count - L"
  # "Frames Processed - L"
  # "Recovery Search move Count - L"
  # "Recovery Search Attempt Count- L"
  # "Next Main State"
  # "Settings -- Update in a slow loop"
  # "Recovery Mode Count - L"
  # "Delta Move Sum - L"
  # "Frames Processed\nLeft"
  # "Move Respond - L"
  # "Replace these with\nconstants"
  # "Initial Search Direction\n- Left"
  # "Read Inputs when Available"
  # "# of Physical Beacons"
  # "Right Data Internal Falg"
  # "Left Data Internal Falg"
  # "Initialize Shift Arrays"
  # "Robot Position (cluster)\nShift Array"
  # "Robot Position (cluster)\nShift Array"
  # "Position Valid Shift Array"
  # "Orientation Shift Array"
  # "Position Valid Shift Array"
  # "Orientation Shift Array"
  # "Servo Communication (to Servo- UART))"
  # "Internal Local Variables"
  # "Servo Control Logic"
  # "Local Variables"
  # "Images to Robot Position Calculation Process"
  # "SERVO MOTOR CONTROL"
  # "SERVO MOTOR CONTROL"
  n1 = Divide(x="Cam AOV Horizontal (deg)", y="Image Width (px)") -> (x/y=w25:sgl)
  n2 = Divide(x="Cam AOV Vertical (deg)", y="Image Height (px)") -> (x/y=w26:sgl)
  n3 = Bundle(w25, w26) -> (w20:cluster{sgl, sgl})  [unwired: 1 in]
  "Angle to Pixel Ratios" <- w20
  n4 = disable-structure shown="Disabled" {
    frame Disabled {
      # "Always Read Incoming Flags & Store"
      n5 = while {
        tunnel: "Check Shared Var Timer" -> [w47]
        stop <- FALSE stop-if-true
        n6 = shared-variable "RT myRIO Target - Overlord\\Localization_Variables_r0.lvlib\\Left_Flag"() -> (→"Left_Flag 2":bool)  [unwired: 1 in, 1 out]
        n7 = shared-variable "RT myRIO Target - Overlord\\Localization_Variables_r0.lvlib\\RIGHT_FLAG"() -> (→"Right_Flag 2":bool)  [unwired: 1 in, 1 out]
        n8 = call "Wait8"("Count(mSec)"=w47) -> ()  [unwired: 1 out]
      }
    }
    frame Enabled {
    }
  }
  n9 = while {
    shift-right: [w55] -> _
    shift-left: w2 -> [w60]
    shift-right: [w54] -> _
    shift-left: w2 -> [w58]
    tunnel: w20 -> [w56]
    tunnel: "Num of Beacons (Total)" -> [w57]
    stop <- FALSE stop-if-true
    # "Wait for Both Internal Flags"
    n10 = call "Wait6"("Count(mSec)"="Fetch Input\n(mSec)") -> ()  [unwired: 1 out]
    n11 = shared-variable "RT myRIO Target - Overlord\\Localization_Variables_r0.lvlib\\Left_Flag"() -> (w48:bool)  [unwired: 1 in, 1 out]
    n12 = shared-variable "RT myRIO Target - Overlord\\Localization_Variables_r0.lvlib\\RIGHT_FLAG"() -> (w49:bool)  [unwired: 1 in, 1 out]
    n13 = case shown="True" w49 {
      tunnel: w57 -> [_ w79]
      tunnel: w56 -> [_ w78]
      tunnel: [w61 w73] -> w51
      tunnel: w58 -> [w61 _]
      frame False {
        # "Don't Update Servo Position\nbc we're waiting on new Data to\ncome in and the servo position\nwas set at the previous set of data"
      }
      frame True {
        w73 = TRUE
        # "Store Values"
        # "Raise Internal Flag"
        # "If New Data Available"
        # "From Shift Reg"
        # "Perforrm Indivudual Angle Calculation"
        # "Pull Down Individual Flag"
        n14 = shared-variable "RT myRIO Target - Overlord\\Localization_Variables_r0.lvlib\\Info - Right"() -> (w69:T6)  [unwired: 1 in, 1 out]
        n15 = shared-variable "RT myRIO Target - Overlord\\Localization_Variables_r0.lvlib\\RIGHT_BEACON_Y_array"() -> (w63:dbl[])  [unwired: 1 in, 1 out]
        "RIGHT Beacon Position - Y px (IN)" <- w63
        n16 = shared-variable "RT myRIO Target - Overlord\\Localization_Variables_r0.lvlib\\RIGHT_BEACON_X_array"() -> (w65:dbl[])  [unwired: 1 in, 1 out]
        "RIGHT Beacon Coord - X px (IN)" <- w65
        n17 = shared-variable "RT myRIO Target - Overlord\\Localization_Variables_r0.lvlib\\Image Lock - R"() -> (w67:bool)  [unwired: 1 in, 1 out]
        n18 = shared-variable "RT myRIO Target - Overlord\\Localization_Variables_r0.lvlib\\RIGHT_BEACON_BOOL_array"() -> (w64:bool[])  [unwired: 1 in, 1 out]
        "Beacons Found\n- Right (Bool Array)" <- w64
        n19 = shared-variable "RT myRIO Target - Overlord\\Localization_Variables_r0.lvlib\\RIGHT_BEACON_Scales"() -> (→"Beacon Scales - Right":sgl[])  [unwired: 1 in, 1 out]
        n20 = Unbundle By Name(w69) -> ("Tracking Coordinates"=w72:cluster{"X":dbl, "Y":dbl}, "Current Valid"=w71:bool, "Current Template"=→"Current Template - Right":T1)
        n21 = local write "Image Lock - Right"(w67) -> ()
        n22 = Bundle("Array of Double"=w65, "Array of Double"=w63) -> (w74:T7)  [unwired: 1 in]
        "Beacon Coordinates - Right Image" <- w74
        n23 = shared-variable "RT myRIO Target - Overlord\\Localization_Variables_r0.lvlib\\Right Servo Angle_Image"() -> (w66:dbl)  [unwired: 1 in, 1 out]
        "This Servo \nAngle - Right" <- w66
        n24 = shared-variable "RT myRIO Target - Overlord\\Localization_Variables_r0.lvlib\\RIGHT_FLAG"(FALSE) -> ()  [unwired: 1 in, 1 out]
        n25 = feedback #1() -> (w81:sgl[])  [unwired: 1 in]
        n26 = feedback #2() -> (w80:bool[])  [unwired: 1 in]
        n27 = call "Angle Calc_Individual Process R4.vi"("Angle to Pixel Ratios"=w78, "Previous Angles"=w81, "Num of Beacons"=w79, "Beacon Coordinates - Image"=w74, "Current Servo Angle"=w66, "Beacons Found (Bool Array)"=w64, "Previous Valid Angles"=w80, "Tracking Coordinates"=w72) -> ("Servo Goal Angle"=w77:sgl, "Valid Beacons (Bool Array)\nPosition Calc"=w76:bool[], "Angle Of Beacons \nRelative to Robot"=w75:sgl[])  [unwired: 4 in, 1 out]
        n28 = feedback-in #1(w75) -> ()
        n29 = feedback-in #2(w76) -> ()
        n30 = local write "Tracking Angle - Right"(w77) -> ()
        n31 = local write "Beacon Angles -R"(w75) -> ()
        n32 = local write "Valid Angles -R"(w76) -> ()
        n33 = local write "Track Angle Valid  - Right"(w71) -> ()
        n34 = local write "New Data  Flag\nRight Servo"(w73) -> ()
      }
    }
    "Right Data\nInput Flag\n- Internal" <- w51
    n35 = case shown="True" w48 {
      tunnel: [w82 w94] -> w50
      tunnel: w60 -> [w82 _]
      tunnel: w56 -> [_ w96]
      tunnel: w57 -> [_ w95]
      frame False {
        # "Don't Update Servo Position\nbc we're waiting on new Data to\ncome in and the servo position\nwas set at the previous set of data"
      }
      frame True {
        w94 = TRUE
        # "Store Values"
        # "Raise Internal Flag"
        # "If New Data Available"
        # "Perforrm Indivudual Angle Calculation"
        # "Pull Down Individual Flag"
        n36 = shared-variable "RT myRIO Target - Overlord\\Localization_Variables_r0.lvlib\\LEFT_BEACON_Scales"() -> (→"Beacon Scales - Left":sgl[])  [unwired: 1 in, 1 out]
        n37 = shared-variable "RT myRIO Target - Overlord\\Localization_Variables_r0.lvlib\\LEFT_BEACON_BOOL_array"() -> (w85:bool[])  [unwired: 1 in, 1 out]
        "Beacons Found\n- Left (Bool Array) 2" <- w85
        n38 = shared-variable "RT myRIO Target - Overlord\\Localization_Variables_r0.lvlib\\LEFT_BEACON_X_array"() -> (w86:dbl[])  [unwired: 1 in, 1 out]
        "LEFT Beacon Coord - X px (IN) 2" <- w86
        n39 = shared-variable "RT myRIO Target - Overlord\\Localization_Variables_r0.lvlib\\LEFT_BEACON_Y_array"() -> (w84:dbl[])  [unwired: 1 in, 1 out]
        "LEFT Beacon Position - Y px (IN) 2" <- w84
        n40 = shared-variable "RT myRIO Target - Overlord\\Localization_Variables_r0.lvlib\\Info - Left"() -> (w90:T6)  [unwired: 1 in, 1 out]
        n41 = shared-variable "RT myRIO Target - Overlord\\Localization_Variables_r0.lvlib\\Image Lock - L"() -> (w88:bool)  [unwired: 1 in, 1 out]
        n42 = Unbundle By Name(w90) -> ("Tracking Coordinates"=w93:cluster{"X":dbl, "Y":dbl}, "Current Valid"=w92:bool, "Current Template"=→"Current Template - Left":T1)
        n43 = local write "Image Lock - Left"(w88) -> ()
        n44 = Bundle("Array of Double"=w86, "Array of Double"=w84) -> (w100:T7)  [unwired: 1 in]
        "Beacon Coordinates - Left Image" <- w100
        n45 = shared-variable "RT myRIO Target - Overlord\\Localization_Variables_r0.lvlib\\Left Servo Angle_Image"() -> (w87:dbl)  [unwired: 1 in, 1 out]
        "This Servo \nAngle - Left" <- w87
        n46 = shared-variable "RT myRIO Target - Overlord\\Localization_Variables_r0.lvlib\\Left_Flag"(FALSE) -> ()  [unwired: 1 in, 1 out]
        n47 = feedback #3() -> (w102:sgl[])  [unwired: 1 in]
        n48 = feedback #4() -> (w101:bool[])  [unwired: 1 in]
        n49 = call "Angle Calc_Individual Process R4.vi"("Angle to Pixel Ratios"=w96, "Previous Angles"=w102, "Num of Beacons"=w95, "Beacon Coordinates - Image"=w100, "Current Servo Angle"=w87, "Beacons Found (Bool Array)"=w85, "Previous Valid Angles"=w101, "Tracking Coordinates"=w93) -> ("Servo Goal Angle"=w99:sgl, "Valid Beacons (Bool Array)\nPosition Calc"=w98:bool[], "Angle Of Beacons \nRelative to Robot"=w97:sgl[])  [unwired: 4 in, 1 out]
        n50 = feedback-in #3(w97) -> ()
        n51 = feedback-in #4(w98) -> ()
        n52 = local write "Beacon Angles - L"(w97) -> ()
        n53 = local write "Valid Angles - L"(w98) -> ()
        n54 = local write "Tracking Angle - Left"(w99) -> ()
        n55 = local write "Track Angle Valid - Left"(w92) -> ()
        n56 = local write "New Data  Flag\nLeft Servo"(w94) -> ()
      }
    }
    "Left Data\nInput Flag\n- Internal" <- w50
    n57 = And(x=w50, y=w51) -> (x .and. y?=w59:bool)
    n58 = case shown="True" w59 {
      selector: w59 -> [_ w105]
      tunnel: w50 -> [w104 _]
      tunnel: [w104 w106] -> w55
      tunnel: [w103 w106] -> w54
      tunnel: w51 -> [w103 _]
      frame False {
      }
      frame True {
        w106 = FALSE
        # "Reset Internal Data Flags"
        # "Position Data\nReady Enabled"
        n59 = local write "Position Calc\nReady"(w105) -> ()
      }
    }
  }
  n60 = Bundle(w34, w34) -> (w37:cluster{sgl, sgl})  [unwired: 1 in]
  n61 = Initialize Array(w34, "History Size") -> (w32:sgl[])
  n62 = Initialize Array(w37, "History Size") -> (w33:cluster{sgl, sgl}[])
  n63 = Initialize Array(FALSE, "History Size") -> (w31:bool[])
  n64 = call "Tick Count4"() -> ("Tick Count(uSec)"=w30:u32)
  n65 = while {
    shift-right: [w117] -> _
    shift-left: w32 -> [w114]
    shift-right: [w116] -> _
    shift-left: w31 -> [w115]
    shift-right: [w118] -> _
    shift-left: w33 -> [w109]
    shift-right: [w110] -> _
    shift-left: w30 -> [w111]
    stop <- "stop" stop-if-true
    n66 = call "Wait5"("Count(mSec)"="Position Calc\nTimer") -> ()  [unwired: 1 out]
    n67 = case shown="True" "Position Calc\nReady" {
      selector: "Position Calc\nReady" -> [_ w209]
      tunnel: w109 -> [_ w227]
      tunnel: w109 -> [w127 w222]
      tunnel: w114 -> [w129 w221]
      tunnel: w115 -> [w128 w220]
      tunnel: [w129 w226] -> w117
      tunnel: [w128 w224] -> w116
      tunnel: [w127 w225] -> w118
      tunnel: w115 -> [_ w219]
      tunnel: w114 -> [_ w218]
      tunnel: [w126 w214] -> w112
      tunnel: w111 -> [_ w214]
      tunnel: [FALSE TRUE] -> w113
      tunnel: w109 -> [_ w211]
      frame False {
        n68 = call "Tick Count5"() -> ("Tick Count(uSec)"=w126:u32)
      }
      frame True {
        w130 = T1."Range 0" ("Current Template - Left")
        w152 = 0.0 ("y")
        # "***************************"
        # "dY"
        # "dX"
        # "Valid"
        # "Find Local Coordinates"
        # "Valid COunt"
        # "Make sure 2+ Data Sets are Still available"
        # "Check 1st element\nwith rest of elements"
        # "Make Sure all Pointed \nIn Same Direction"
        # "For Each Valid Beacon\nCalculate Distance from Each Camera to Each Beacon"
        # "Find Common Beacons\nAmong Cameras"
        # "Currently will only\ncalculate position if 2+ \nbeacons are available \nfrom both cameras"
        # "System is in Normal (long range) State"
        # "Average Both Data Sets"
        # "Estimate Distance for each Available Beacon Angle\nPER Camera, indivduallly"
        # "At least 2+ Avaialbe"
        # "CALCULATE AVERAGE ORIENTATION"
        # "Update Outputs\nif Current Calc is Invalid\n(shouldn't matter)"
        # "Estimate Orienation Based on Previous Position"
        # "****# of previous in history that must be true\nin order for position to be considered \"locked\""
        # "New Position is Valid if both \nOrientation and Positions\nis within range of previous"
        # "Robot Position\n Shift Array"
        # "Position Valid Shift Array"
        # "Orientation Shift Array"
        # "Orientation Value"
        # "Shift & Insert Current Position Valid"
        # "Position Valid\n(orientation)"
        # "Position Valid\n(position)"
        # "Update Shift Registers"
        # "Shift & Insert Current Calculated Orientation"
        # "Shift & Insert Current Robot Position"
        # "UPDATE FINAL OUTPUT\n VALUES"
        n69 = local read "Num of Beacons (Total)"() -> (w192:i8)
        n70 = Not(x=w209) -> (.not. x?=w210:bool)
        n71 = local write "Position Calc\nReady"(w210) -> ()
        n72 = disable-structure shown="Disabled" {
          frame Disabled {
            w277 = T8."Normal - 5" ("Initial State")
            # "***********do for both"
            # "sTATE"
            n73 = local read item#-1() -> (w281)
            n74 = local read item#-1() -> (w280)
            n75 = Equal?(x=w281, y=w277) -> (x = y?=w279:bool)
            n76 = Equal?(x=w280, y=w277) -> (x = y?=w278:bool)
            n77 = And(x=w279, y=w278) -> ()  [unwired: 1 out]
          }
          frame Enabled {
          }
        }
        n78 = local read "Current Template - Left"() -> (w156:T1)
        n79 = local read "Current Template - Right"() -> (w155:T1)
        n80 = local read "Beacon Scales - Left"() -> (w198:sgl[])
        n81 = local read "Beacon Scales - Right"() -> (w195:sgl[])
        n82 = for {
          N: w192 -> [_]
          tunnel: "Valid Angles - L" -> [w415] mode=indexing
          tunnel: "Beacon Angles - L" -> [w422] mode=indexing
          tunnel: w198 -> [w423] mode=indexing
          tunnel: "Valid Angles -R" -> [w408] mode=indexing
          tunnel: "Beacon Angles -R" -> [w421] mode=indexing
          tunnel: w195 -> [w420] mode=indexing
          tunnel: "Distance Between \nCameras  (*unit)" -> [w419]
          tunnel: [w414] -> w189 mode=indexing
          tunnel: [w413] -> w188 mode=indexing
          tunnel: [w412] -> w190 mode=indexing
          tunnel: [w411] -> w159 mode=indexing
          tunnel: [w410] -> w158 mode=indexing
          tunnel: [w409] -> w157 mode=indexing
          tunnel: w156 -> [w407]
          tunnel: w155 -> [w406]
          # "dY"
          # "dX"
          # "Valid"
          # "If Both Cameras are using Same Beacon Data,\nAverage the 2 independently esitmated positions"
          # "dY"
          # "dX"
          # "dY"
          # "dX"
          n83 = case shown="True" w415 {
            tunnel: w422 -> [_ w500]
            tunnel: [w487 w491] -> w417
            tunnel: [w487 w492] -> w416
            tunnel: w423 -> [_ w490]
            tunnel: w407 -> [_ w489]
            frame False {
              w487 = sgl 0.0
              # "Current Data Set Was Not Valid\nFill with 0\nWill not be used later"
            }
            frame True {
              # "Estimate Distance"
              # "Negate dX if A2>90"
              # "Find LOCAL Coordinate of Each Beacon"
              # "Current - Valid Data Set"
              n84 = call "Beacon_Scale_to_Distance_R0.vi"("Scale - In"=w490, "Current Template - In"=w489) -> ("Distance - Out"=w488:sgl)  [unwired: 9 in]
              n85 = Less?(x=w500, y=sgl 90.0) -> (x < y?=w502:bool)
              n86 = case shown="False" w502 {
                tunnel: w500 -> [w509 w511]
                tunnel: [w507 w512] -> w499
                tunnel: [FALSE TRUE] -> w494
                frame False {
                  # "Negative Y"
                  # "A2 is > 90"
                  n87 = Subtract(x=w509, y=sgl 90.0) -> (x-y=w507:sgl)
                }
                frame True {
                  # "Positive Y"
                  # "A2 is < 90"
                  n88 = Subtract(x=sgl 90.0, y=w511) -> (x-y=w512:sgl)
                }
              }
              "dA2 2" <- w499
              n89 = expression code="(x/180.0)*pi" "degrees to radians"(w499) -> (w497:sgl)
              n90 = expression code="(x/180.0)*pi" "degrees to radians"(w499) -> (w498:sgl)
              n91 = Cosine(x=w497) -> (cos(x)=w495:sgl)
              n92 = Sine(x=w498) -> (sin(x)=w496:sgl)
              n93 = Multiply(x=w488, y=w495) -> (x*y=w492:sgl)
              n94 = Multiply(x=w488, y=w496) -> (x*y=w493:sgl)
              n95 = case shown="True" w494 {
                tunnel: w493 -> [w504 w505]
                tunnel: [w503 w505] -> w491
                frame False {
                  n96 = Negate(x=w504) -> (-x=w503:sgl)
                }
                frame True {
                }
              }
            }
          }
          n97 = case shown="True" w408 {
            tunnel: w421 -> [_ w473]
            tunnel: [w458 w464] -> w410
            tunnel: [w458 w463] -> w411
            tunnel: w420 -> [_ w460]
            tunnel: w419 -> [_ w465]
            tunnel: [w458 w462] -> w409
            tunnel: w406 -> [_ w461]
            frame False {
              w458 = sgl 0.0
              # "Current Data Set Was Not Valid\nFill with 0\nWill not be used later"
            }
            frame True {
              # "Add delta for\nRIGHT camera ONLY"
              # "Estimate Distance"
              # "Negate dX if A2>90"
              # "Find LOCAL Coordinate of Each Beacon"
              # "Current - Valid Data Set"
              n98 = call "Beacon_Scale_to_Distance_R0.vi"("Scale - In"=w460, "Current Template - In"=w461) -> ("Distance - Out"=w459:sgl)  [unwired: 9 in]
              n99 = Less?(x=w473, y=sgl 90.0) -> (x < y?=w475:bool)
              n100 = case shown="False" w475 {
                tunnel: w473 -> [w482 w484]
                tunnel: [w480 w485] -> w472
                tunnel: [FALSE TRUE] -> w467
                frame False {
                  # "Negative Y"
                  # "A2 is > 90"
                  n101 = Subtract(x=w482, y=sgl 90.0) -> (x-y=w480:sgl)
                }
                frame True {
                  # "Positive Y"
                  # "A2 is < 90"
                  n102 = Subtract(x=sgl 90.0, y=w484) -> (x-y=w485:sgl)
                }
              }
              "dA2 3" <- w472
              n103 = expression code="(x/180.0)*pi" "degrees to radians"(w472) -> (w470:sgl)
              n104 = expression code="(x/180.0)*pi" "degrees to radians"(w472) -> (w471:sgl)
              n105 = Cosine(x=w470) -> (cos(x)=w468:sgl)
              n106 = Sine(x=w471) -> (sin(x)=w469:sgl)
              n107 = Multiply(x=w459, y=w468) -> (x*y=w463:sgl)
              n108 = Multiply(x=w459, y=w469) -> (x*y=w466:sgl)
              n109 = case shown="True" w467 {
                tunnel: w466 -> [w477 w478]
                tunnel: [w476 w478] -> w462
                frame False {
                  n110 = Negate(x=w477) -> (-x=w476:sgl)
                }
                frame True {
                }
              }
              n111 = Add(x=w465, y=w462) -> (x+y=w464:sgl)
            }
          }
          n112 = And(x=w415, y=w408) -> (x .and. y?=w418:bool)
          n113 = case shown="False" w418 {
            tunnel: w417 -> [w431 w457]
            tunnel: w416 -> [w428 w456]
            tunnel: w410 -> [w430 w455]
            tunnel: w411 -> [w429 w454]
            tunnel: [w426 w450] -> w414
            tunnel: [w425 w449] -> w413
            tunnel: w415 -> [w427 _]
            tunnel: w408 -> [w432 _]
            tunnel: [w424 TRUE] -> w412
            frame False {
              n114 = Exclusive Or(1:w432, 2:w427) -> (0:w433:bool)
              n115 = case shown="True" w433 {
                tunnel: w431 -> [_ w441]
                tunnel: w430 -> [_ w438]
                tunnel: w429 -> [_ w437]
                tunnel: w428 -> [_ w439]
                tunnel: w427 -> [_ w443]
                tunnel: [w434 w442] -> w426
                tunnel: [w434 w440] -> w425
                tunnel: [FALSE TRUE] -> w424
                frame False {
                  w434 = sgl 0.0
                  # "None are valid,"
                }
                frame True {
                  # "Only 1 beacon is valid,\nUse the valid beacon"
                  n116 = case shown="False" w443 {
                    tunnel: [w445 w447] -> w442
                    tunnel: w441 -> [_ w447]
                    tunnel: [w444 w446] -> w440
                    tunnel: w439 -> [_ w446]
                    tunnel: w438 -> [w445 _]
                    tunnel: w437 -> [w444 _]
                    frame False {
                      # "Left is invalid,\nRight MUST be valid"
                    }
                    frame True {
                      # "Left is Valid"
                    }
                  }
                }
              }
            }
            frame True {
              w451 = sgl 2.0 ("y")
              # "Both are Valid"
              n117 = Add(x=w457, y=w455) -> (x+y=w452:sgl)
              n118 = Add(x=w456, y=w454) -> (x+y=w453:sgl)
              n119 = Divide(x=w453, y=w451) -> (x/y=w449:sgl)
              n120 = Divide(x=w452, y=w451) -> (x/y=w450:sgl)
            }
          }
        }
        "Array" <- w159
        "Array 2" <- w158
        "Array 3" <- w157
        n121 = And(x="Valid Angles - L", y="Valid Angles -R") -> (x .and. y?=w180:bool[])
        n122 = Boolean To (0,1)(Boolean=w180) -> (0, 1=w177:i16[])
        n123 = Add Array Elements(numeric array=w177) -> (sum=w178:i16)
        n124 = Greater?(x=w178, y=1) -> (0:w176:bool)
        n125 = for {
          N: w192 -> [_]
          tunnel: w176 -> [w342]
          tunnel: "Beacon Angles - L" -> [w341] mode=indexing
          tunnel: "Beacon Angles -R" -> [w340] mode=indexing
          tunnel: "Distance Between \nCameras  (*unit)" -> [w339]
          tunnel: "Distance Threshold\nRef Triangles (*unit)" -> [w338]
          tunnel: [w337] -> w163 mode=indexing
          tunnel: [w336] -> _ mode=indexing
          tunnel: [w335] -> w162 mode=indexing
          tunnel: [w334] -> _ mode=indexing
          tunnel: [w333] -> w164 mode=indexing
          tunnel: [w332] -> w170 mode=indexing
          n126 = case shown="True" w342 {
            tunnel: w341 -> [w347 w357]
            tunnel: w340 -> [w346 w356]
            tunnel: w339 -> [_ w348]
            tunnel: w338 -> [_ w349]
            tunnel: [w347 w355] -> w337
            tunnel: [w346 w354] -> w336
            tunnel: [FALSE w353] -> w335
            tunnel: [w344 w352] -> w334
            tunnel: [w344 w351] -> w333
            tunnel: [0 w350] -> w332
            frame False {
              w344 = sgl 1.0
            }
            frame True {
              # "Build Reference Triangle"
              n127 = call "Position Calc_Build Reference Triangle_R1.vi"("A2_in"=w357, "A3_in"=w356, "S1 (Length Between\n Cameras - inches)"=w348, "Distance\nThreshold"=w349) -> ("S2"=w352:sgl, "S3"=w351:sgl, "Direction"=w350:i8, "A2"=w355:sgl, "A3"=w354:sgl, "Accept"=w353:bool)  [unwired: 6 in]
            }
          }
        }
        n128 = for {
          N: w192 -> [_]
          tunnel: w162 -> [w327] mode=indexing
          tunnel: w170 -> [w331] mode=indexing
          tunnel: [w331] -> w172 mode=indexing if=w327
          shift-right: [w330] -> w166
          shift-left: 0 -> [w328]
          # "Only add to array\nif valid distance"
          n129 = Increment(x=w328) -> (x+1=w329:i32)
          n130 = Select(t=w329, s=w327, f=w328) -> (s? t:f=w330:i32)
        }
        n131 = Index Array(array=w172, index=0) -> (element=w173:i32)
        n132 = Equal?(x=w172, y=w173) -> (x = y?=w174:bool[])
        n133 = And Array Elements(Boolean array=w174) -> (logical AND=w168:bool)
        n134 = Greater?(x=w166, y=1) -> (0:w167:bool)
        n135 = And(x=w168, y=w167) -> (x .and. y?=w161:bool)
        n136 = case shown="True" w161 {
          tunnel: w192 -> [w284 w293]
          tunnel: w164 -> [_ w292]
          tunnel: w163 -> [_ w291]
          tunnel: w162 -> [_ w290]
          tunnel: [w283 w289] -> w191
          tunnel: [w282 w288] -> w187
          tunnel: [w282 w287] -> w186
          frame False {
            # "Build Array for False"
            n137 = for {
              N: w284 -> [_]
              tunnel: [sgl 0.0] -> w282 mode=indexing
              tunnel: [FALSE] -> w283 mode=indexing
            }
          }
          frame True {
            n138 = for {
              N: w293 -> [_]
              tunnel: w291 -> [w299] mode=indexing
              tunnel: w292 -> [w298] mode=indexing
              tunnel: [w297] -> w288 mode=indexing
              tunnel: [w296] -> w287 mode=indexing
              tunnel: [w295] -> w289 mode=indexing
              tunnel: w290 -> [w294] mode=indexing
              n139 = case shown="True" w294 {
                selector: w294 -> [w301 w305]
                tunnel: w299 -> [_ w313]
                tunnel: [w300 w303] -> w297
                tunnel: [w300 w304] -> w296
                tunnel: w298 -> [_ w302]
                tunnel: [w301 w305] -> w295
                frame False {
                  w300 = sgl 0.0
                  # "Current Data Set Was Not Valid\nFill with 0\nWill not be used later"
                }
                frame True {
                  # "dY"
                  # "dX"
                  # "Negate dX if A2>90"
                  # "Find LOCAL Coordinate of Each Beacon"
                  # "Current - Valid Data Set"
                  n140 = Less?(x=w313, y=sgl 90.0) -> (x < y?=w315:bool)
                  n141 = case shown="False" w315 {
                    tunnel: w313 -> [w322 w324]
                    tunnel: [w320 w325] -> w312
                    tunnel: [FALSE TRUE] -> w307
                    frame False {
                      # "Negative Y"
                      # "A2 is > 90"
                      n142 = Subtract(x=w322, y=sgl 90.0) -> (x-y=w320:sgl)
                    }
                    frame True {
                      # "Positive Y"
                      # "A2 is < 90"
                      n143 = Subtract(x=sgl 90.0, y=w324) -> (x-y=w325:sgl)
                    }
                  }
                  "dA2 4" <- w312
                  n144 = expression code="(x/180.0)*pi" "degrees to radians"(w312) -> (w310:sgl)
                  n145 = expression code="(x/180.0)*pi" "degrees to radians"(w312) -> (w311:sgl)
                  n146 = Cosine(x=w310) -> (cos(x)=w308:sgl)
                  n147 = Sine(x=w311) -> (sin(x)=w309:sgl)
                  n148 = Multiply(x=w302, y=w308) -> (x*y=w304:sgl)
                  n149 = Multiply(x=w302, y=w309) -> (x*y=w306:sgl)
                  n150 = case shown="True" w307 {
                    tunnel: w306 -> [w317 w318]
                    tunnel: [w316 w318] -> w303
                    frame False {
                      n151 = Negate(x=w317) -> (-x=w316:sgl)
                    }
                    frame True {
                    }
                  }
                }
              }
            }
          }
        }
        n152 = Subtract(x=sgl 1.0, y="Triangle Based\nWeight") -> (x-y=w183:sgl)
        "Scale Based\nWeight" <- w183
        n153 = for {
          N: w192 -> [_]
          tunnel: w191 -> [w362] mode=indexing
          tunnel: w190 -> [w361] mode=indexing
          tunnel: w189 -> [w366] mode=indexing
          tunnel: w188 -> [w365] mode=indexing
          tunnel: w187 -> [w368] mode=indexing
          tunnel: w186 -> [w367] mode=indexing
          tunnel: "Triangle Based\nWeight" -> [w364]
          tunnel: w183 -> [w363]
          tunnel: [w360] -> w160 mode=indexing
          tunnel: [w359] -> w182 mode=indexing
          tunnel: [w358] -> w181 mode=indexing
          # "If Beacon info \nis available from\nboth"
          n154 = And(x=w362, y=w361) -> (x .and. y?=w369:bool)
          n155 = case shown="True" w369 {
            selector: w369 -> [_ w395]
            tunnel: w368 -> [w376 w403]
            tunnel: w367 -> [w374 w404]
            tunnel: w366 -> [w372 w402]
            tunnel: w365 -> [w371 w401]
            tunnel: w364 -> [_ w405]
            tunnel: w363 -> [_ w400]
            tunnel: [w375 w393] -> w358
            tunnel: [w377 w394] -> w359
            tunnel: w362 -> [w378 _]
            tunnel: w361 -> [w373 _]
            tunnel: [w370 w395] -> w360
            frame False {
              n156 = case shown="False" w378 {
                selector: w378 -> [_ w390]
                tunnel: [w383 w392] -> w377
                tunnel: w376 -> [_ w392]
                tunnel: [w381 w391] -> w375
                tunnel: w374 -> [_ w391]
                tunnel: w373 -> [w384 _]
                tunnel: w372 -> [w382 _]
                tunnel: w371 -> [w380 _]
                tunnel: [w379 w390] -> w370
                frame False {
                  n157 = case shown="False" w384 {
                    selector: w384 -> [w385 w387]
                    tunnel: [w386 w389] -> w383
                    tunnel: w382 -> [_ w389]
                    tunnel: [w386 w388] -> w381
                    tunnel: w380 -> [_ w388]
                    tunnel: [w385 w387] -> w379
                    frame False {
                      w386 = sgl 0.0
                      # "None avail"
                    }
                    frame True {
                    }
                  }
                }
                frame True {
                }
              }
            }
            frame True {
              n158 = Multiply(x=w403, y=w405) -> (x*y=w399:sgl)
              n159 = Multiply(x=w404, y=w405) -> (x*y=w397:sgl)
              n160 = Multiply(x=w402, y=w400) -> (x*y=w398:sgl)
              n161 = Multiply(x=w401, y=w400) -> (x*y=w396:sgl)
              n162 = Add(x=w399, y=w398) -> (x+y=w394:sgl)
              n163 = Add(x=w397, y=w396) -> (x+y=w393:sgl)
            }
          }
        }
        "Valid Beacon Sets_" <- w160
        n164 = Boolean To (0,1)(Boolean=w160) -> (0, 1=w203:i16[])
        n165 = Add Array Elements(numeric array=w203) -> (sum=w202:i16)
        n166 = Greater?(x=w202, y=i16 1) -> (0:w200:bool)
        n167 = case shown="True" w200 {
          tunnel: w227 -> [_ w604]
          tunnel: [0.0 ("f") w603] -> w223
          tunnel: [w516 w602] -> w146
          tunnel: w219 -> [_ w523]
          tunnel: w218 -> [_ w601]
          tunnel: [FALSE w600] -> w144
          tunnel: [FALSE w599] -> w142
          tunnel: w211 -> [_ w598]
          tunnel: [sgl 0.0 w596] -> w204
          tunnel: "Distance Between \nCameras  (*unit)" -> [_ w535]
          tunnel: w182 -> [_ w534]
          tunnel: w181 -> [_ w533]
          tunnel: w160 -> [_ w532]
          tunnel: w192 -> [_ w531]
          frame False {
            w515 = 0.0 ("f")
            n168 = Bundle("f"=w515, "f"=w515) -> (w516:cluster{"f":dbl, "f":dbl})  [unwired: 1 in]
          }
          frame True {
            w568 = sgl 2.0
            w585 = 0
            # "Current Orientaiton"
            # "Valid Position Ccount\n(within moving avg\nwinfow)"
            # "Valid Position Ccount"
            # "Only Apply This Filtering \nif 3 or More Beacons Still Valid"
            # "Orientation Value"
            # "Orientation Valid"
            # "Y (current)"
            # "X (current)"
            # "Number of Valid\nPrevious Orientations"
            # "More than 1 Previous\nValid Positions"
            # "More than\n2previous position\navailable"
            # "Choose Beacon Set\nwith Lowest Std Dev"
            # "Y value cannot be negative"
            # "Find New # Of Valid Beacons"
            # "Adjust/Normalize\nLocal Beacon Positions\nusing Line of Best fit"
            # "# Valid\nData Sets"
            # "cam, y"
            # "cam, x"
            # "Calculate dX and dY\nfor right cam"
            # "Average dX and dY from each (valid) beacon to find position of each camera\n\nthen average all  positions for each camera find center between"
            # "Convert Slope\nto Radians"
            # "*rotate CCW in rad"
            # "Rotate Coordinate\n System by Slope"
            n169 = Boolean To (0,1)(Boolean=w523) -> (0, 1=w552:i16[])
            n170 = Initialize Array(u8 0, "Moving Average\nWindow Length") -> (w528:u8[])
            n171 = Add Array Elements(numeric array=w552) -> (sum=w522:i16)
            n172 = Greater?(x=w522, y=0) -> (0:w525:bool)
            n173 = while {
              shift-right: [w606] -> w526
              shift-left: w528 -> [w608]
              tunnel: w523 -> [w613] mode=indexing
              shift-right: [w612] -> w524
              shift-left: u8 0 -> [w614]
              tunnel: "Moving Average\nWindow Length" -> [w605]
              i -> [w607]
              stop <- w609 stop-if-true
              # "Grab Last 2 Valid Position Indexes"
              n174 = case shown="True" w613 {
                tunnel: w614 -> [w616 w618]
                tunnel: [w616 w621] -> w612
                tunnel: w608 -> [w615 w620]
                tunnel: w607 -> [_ w619]
                tunnel: [w615 w617] -> w606
                frame False {
                }
                frame True {
                  # "Update Index\nto use"
                  # "Increment\nValid Count"
                  n175 = Replace Array Subset(array=w620, new element=w619, index=w618) -> (w617:u8[])
                  n176 = Increment(x=w618) -> (x+1=w621:u8)
                }
              }
              n177 = Greater Or Equal?(x=w612, y=w605) -> (x >= y?=w611:bool)
              n178 = Greater Or Equal?(x=w607, y=w605) -> (x >= y?=w610:bool)
              n179 = Or(x=w611, y=w610) -> (x .or. y?=w609:bool)
            }
            n180 = Bundle(w534, w533) -> (→"LOCAL\nBeacon Coordinates\nRelative to Robot" →"Local Coordinates - Calculated":cluster{sgl[], sgl[]})  [unwired: 1 in]
            n181 = call "Coordinate_Outlier_Filtering_R2.vi"("Num of Beacons"=w531, "Max Std Dev(all 5)"="Max Std Dev (5)", "X in"=w534, "Valid Data\nSets in"=w532, "Y in"=w533, "Max Std Dev( 4 )"="Max Std Dev (4)", "Max Std Dev (3)"="Max Std Dev (3)") -> ("Y out"=w545:sgl[], "X out"=w546:sgl[], "Valid Beacons\nout"=w543:bool[], "Slope out"=w551:dbl)  [unwired: 3 in, 2 out]
            n182 = Inverse Tangent(1:w551) -> (0:w564:dbl)
            n183 = expression code="(x/pi)*180.0" "radians to degrees"(w564) -> (w550:dbl)
            n184 = Boolean To (0,1)(Boolean=w543) -> (0, 1=w542:i16[])
            n185 = To Single Precision Float(number=w550) -> (single precision float=w596:sgl)
            n186 = case shown="True" w525 {
              tunnel: [w631 w652] -> w599
              tunnel: w601 -> [_ w654]
              tunnel: w596 -> [w632 w649]
              tunnel: [w630 w653] -> w603
              tunnel: w598 -> [_ _]
              tunnel: w526 -> [_ w650]
              tunnel: w524 -> [_ w641]
              frame False {
                # "Since no history available,\ncheck that current is with 0-360"
                # "Use Current Orientation bc \nPrevious are not available"
                # "New Position\nValid"
                n187 = In Range and Coerce(upper limit=sgl 360.0, x=w632, lower limit=sgl -360.0 ("upper limit")) -> (In Range?=w631:bool)  [unwired: 1 out]
                n188 = Select(t=w632, s=w631, f=sgl 0.0) -> (s? t:f=w630:sgl)
              }
              frame True {
                # "Calculate New, Weighted\nOrientation"
                # "Moving Average Out"
                n189 = local read "Last Position"() -> (w639:cluster{"X":sgl, "Y":sgl})
                n190 = Unbundle By Name(w639) -> ("X"=w636:sgl)
                n191 = call "Scaling and Mapping2"("Signals"=w636) -> ("Scaled Signals"=w638:dynamicdata)  [unwired: 9 in, 1 out]
                n192 = for {
                  N: w641 -> [_]
                  shift-right: [w678] -> w647
                  shift-left: 0.0 -> [w677]
                  tunnel: w650 -> [w676] mode=indexing
                  tunnel: w654 -> [w674]
                  # "Fetch Last Valid Values\nand Sum"
                  n193 = Index Array(array=w674, index=w676) -> (element=w675:sgl)
                  n194 = Add(x=w675, y=w677) -> (x+y=w678:dbl)
                }
                n195 = To Single Precision Float(number=w638) -> (single precision float=w637:sgl)
                "New Orientation\nWeight" <- w637
                n196 = Subtract(x=sgl 1.0, y=w637) -> (x-y=w646:sgl)
                n197 = Multiply(x=w649, y=w637) -> (x*y=w644:sgl)
                n198 = Multiply(x=w646, y=w647) -> (x*y=w642:dbl)
                n199 = To Double Precision Float(number=w641) -> (double precision float=w640:dbl)
                n200 = Divide(x=w642, y=w640) -> (x/y=w643:dbl)
                n201 = Add(x=w644, y=w643) -> (x+y=w645:dbl)
                n202 = Greater Than 0?(x=w641) -> (x > 0?=w651:bool)
                n203 = case shown="True" w651 {
                  tunnel: w645 -> [w658 w664]
                  tunnel: w650 -> [_ w671]
                  tunnel: w654 -> [_ w670]
                  tunnel: [w657 w663] -> w653
                  tunnel: [w656 w666] -> w652
                  frame False {
                    # "No Pevious is Available to Compare\ncheck that current is real angle"
                    n204 = In Range and Coerce(upper limit=sgl 360.0, x=w658, lower limit=sgl -360.0 ("upper limit")) -> (In Range?=w656:bool)  [unwired: 1 out]
                    n205 = Select(t=w658, s=w656, f=sgl 0.0) -> (s? t:f=w657:dbl)
                  }
                  frame True {
                    # "Check That New Value\nis within Range of Old\n(avg)"
                    # "(X1 - X2)^2"
                    # "Previous"
                    # "Pevious is Available to Compare"
                    n206 = Index Array(array=w671, index=u8 0) -> (element=w672:u8)
                    n207 = Index Array(array=w670, index=w672) -> (element=w669:sgl)
                    n208 = Subtract(x=w669, y=w664) -> (x-y=w668:dbl)
                    n209 = Absolute Value(x=w668) -> (abs(x)=w667:dbl)
                    n210 = Less Or Equal?(x=w667, y="New Orientation \nThreshold") -> (x <= y?=w666:bool)
                    n211 = Select(t=w664, s=w666, f=sgl 0.0) -> (s? t:f=w663:dbl)
                  }
                }
              }
            }
            n212 = Add Array Elements(numeric array=w542) -> (sum=w541:i16)
            n213 = Greater?(x=w541, y=i16 2) -> (0:w539:bool)
            n214 = case shown="True" w539 {
              tunnel: w531 -> [_ w629]
              tunnel: w543 -> [w622 w628]
              tunnel: w546 -> [_ w627]
              tunnel: w545 -> [_ w626]
              tunnel: [w622 w625] -> w544
              tunnel: "Distance\nBetween Beacons" -> [_ w624]
              tunnel: "Distance\nBetween Beacons \n- Tolerance" -> [_ w623]
              frame False {
                # "Don't apply filtering,\nnot enough data points"
              }
              frame True {
                # "This will filter beacons if they are calculate to be \ntoo close to each other. The beacon(s) that is\n discarded is chosen based distance between each/every\nbeacon,. Capable of filtering as long as 1/2 of sample\nset has uniform distances (between beacons)."
                # "Validate Distance Between\nEach Beacon"
                n215 = call "Beacon_Filtering_Inter_Beacon_Distance_R1.vi"("Num of Beacons"=w629, "Inter Beacon\nReal Distance"=w624, "X in"=w627, "Inter Beacon\ndelta Threshold"=w623, "Y in"=w626, "Valid Data\nSets in"=w628) -> ("Beacons Valid - Out"=w625:bool[])  [unwired: 9 in]
              }
            }
            "Post Filtering\n- Valid Beacons" <- w544
            n216 = Increment(x=w531) -> (x+1=w586:i8)
            n217 = for {
              N: w586 -> [_]
              tunnel: [w797] -> w587 mode=indexing
              tunnel: w546 -> [w793]
              tunnel: w545 -> [w796]
              tunnel: [w795] -> w588 mode=indexing
              tunnel: w535 -> [w792]
              i -> [w794]
              # "Build Array's of Coordinates\nFor All Objects"
              n218 = Greater Than 0?(x=w794) -> (x > 0?=w798:bool)
              n219 = case shown="True" w798 {
                tunnel: [w800 w806] -> w797
                tunnel: w793 -> [w803 _]
                tunnel: w796 -> [w802 _]
                tunnel: [w799 0.0] -> w795
                tunnel: w794 -> [w804 _]
                tunnel: w792 -> [_ w806]
                frame True {
                  # "Rest of Array is\nBeacon Coordinates"
                  n220 = Decrement(x=w804) -> (x-1=w801:i32)
                  n221 = Index Array(array=w803, index=w801) -> (element=w800:sgl)
                  n222 = Index Array(array=w802, index=w801) -> (element=w799:sgl)
                }
                frame False {
                  # "First object is the\nother Camera\n\nthis coordinate\nis simply:\nx = 0\ny = distance btween cams"
                }
              }
            }
            n223 = Bundle(w587, w588) -> (→"All Object Coordinates \n- Local" →"Local Coordinates - Normalized":cluster{sgl[], dbl[]})  [unwired: 1 in]
            n224 = expression code="(x/180.0)*pi" "degrees to radians"(w603) -> (w549:dbl)
            n225 = call-poly <vilib>:"2D Cartesian Coordinate Rotation.vi"("theta"=w549, "Y"=w588, "X"=w587) -> ("Y Out"=w565:dbl[], "X Out"=w566:dbl[])  [unwired: 6 in, 1 out]
            n226 = Bundle("X Out"=w566, "Y Out"=w565) -> (→"All Object Coordinates \n- Local - Rotated" →"Local Coordinates - Rotated":cluster{"X Out":dbl[], "Y Out":dbl[]})  [unwired: 1 in]
            n227 = Index Array(array=w565, index=w585) -> (element=w561:dbl)
            n228 = Index Array(array=w566, index=w585) -> (element=w584:dbl)
            n229 = for {
              N: w531 -> [_]
              tunnel: w565 -> [w788]
              tunnel: w566 -> [w789]
              tunnel: w584 -> [w787]
              tunnel: w561 -> [w786]
              tunnel: [w785] -> w558 mode=indexing
              tunnel: [w784] -> w557 mode=indexing
              tunnel: [w783] -> w536 mode=indexing
              tunnel: [w782] -> w559 mode=indexing
              i -> [w791]
              n230 = Increment(x=w791) -> (x+1=w790:i32)
              n231 = Index Array(array=w788, index=w790) -> (element=w782:dbl)
              n232 = Index Array(array=w789, index=w790) -> (element=w783:dbl)
              n233 = Subtract(x=w782, y=w786) -> (x-y=w784:dbl)
              n234 = Subtract(x=w783, y=w787) -> (x-y=w785:dbl)
            }
            n235 = Bundle(w558, w557) -> (→"dX, dY\nRight Cam":cluster{dbl[], dbl[]})  [unwired: 1 in]
            n236 = Bundle(w536, w559) -> (→"dX, dY\nLeft Cam":cluster{dbl[], dbl[]})  [unwired: 1 in]
            n237 = Unbundle("Real Beacon\n - Coordinates") -> ("X"=w582:dbl[], "Y"=w562:dbl[])
            n238 = Boolean To (0,1)(Boolean=w544) -> (0, 1=w560:i16[])
            n239 = for {
              N: w531 -> [_]
              tunnel: w544 -> [w768] mode=indexing
              tunnel: w582 -> [w765] mode=indexing
              tunnel: w562 -> [w764] mode=indexing
              tunnel: w536 -> [w767] mode=indexing
              tunnel: w559 -> [w763] mode=indexing
              tunnel: w558 -> [w766] mode=indexing
              tunnel: w557 -> [w762] mode=indexing
              tunnel: [w761] -> w581 mode=indexing
              tunnel: [w760] -> w580 mode=indexing
              tunnel: [w759] -> w579 mode=indexing
              tunnel: [w758] -> w578 mode=indexing
              n240 = case shown="True" w768 {
                tunnel: w767 -> [_ w781]
                tunnel: w766 -> [_ w780]
                tunnel: w765 -> [_ w771]
                tunnel: w764 -> [_ w770]
                tunnel: w763 -> [_ w779]
                tunnel: w762 -> [_ w772]
                tunnel: [w769 w777] -> w761
                tunnel: [w769 w776] -> w760
                tunnel: [w769 w775] -> w759
                tunnel: [w769 w774] -> w758
                frame False {
                  w769 = sgl 0.0
                  # "Add Nothing"
                }
                frame True {
                  # "realX = beaconX + dY\nrealY = beaconY + (-dx)"
                  # "Right Cam"
                  # "Left Cam"
                  # "dX = -dX\nSwap dX, dY"
                  # "Translate to Real Coordinates\nOnly Apply for Valid Beacons"
                  n241 = Negate(x=w781) -> (-x=w778:dbl)
                  n242 = Negate(x=w780) -> (-x=w773:dbl)
                  n243 = Add(x=w771, y=w779) -> (x+y=w777:dbl)
                  n244 = Add(x=w770, y=w778) -> (x+y=w776:dbl)
                  n245 = Add(x=w771, y=w772) -> (x+y=w775:dbl)
                  n246 = Add(x=w770, y=w773) -> (x+y=w774:dbl)
                }
              }
            }
            n247 = Add Array Elements(numeric array=w560) -> (sum=w563:i16)
            n248 = Add Array Elements(numeric array=w581) -> (sum=w577:dbl)
            n249 = Add Array Elements(numeric array=w580) -> (sum=w576:dbl)
            n250 = Add Array Elements(numeric array=w579) -> (sum=w575:dbl)
            n251 = Add Array Elements(numeric array=w578) -> (sum=w574:dbl)
            n252 = Divide(x=w577, y=w563) -> (x/y=w573:dbl)
            n253 = Divide(x=w576, y=w563) -> (x/y=w571:dbl)
            n254 = Divide(x=w575, y=w563) -> (x/y=w572:dbl)
            n255 = Divide(x=w574, y=w563) -> (x/y=w570:dbl)
            n256 = Bundle(w573, w571) -> (→"Left Camera Real Coordinates":cluster{dbl, dbl})  [unwired: 1 in]
            n257 = Bundle(w572, w570) -> (→"Right Camera Real Coordinate":cluster{dbl, dbl})  [unwired: 1 in]
            n258 = Add(x=w573, y=w572) -> (x+y=w569:dbl)
            n259 = Add(x=w571, y=w570) -> (x+y=w567:dbl)
            n260 = Divide(x=w569, y=w568) -> (x/y=w520:dbl)
            n261 = Divide(x=w567, y=w568) -> (x/y=w521:dbl)
            n262 = Bundle(w520, w521) -> (→"Robot Coordinates":cluster{dbl, dbl})  [unwired: 1 in]
            n263 = Less Than 0?(x=w521) -> ()  [unwired: 1 out]
            n264 = case shown="True" w525 {
              tunnel: w522 -> [_ _]
              tunnel: w520 -> [w683 w707]
              tunnel: [w684 w717] -> w600
              tunnel: w604 -> [_ w711]
              tunnel: w521 -> [w682 w694]
              tunnel: [w681 w721] -> w602
              tunnel: "Max X (arena)" -> [w680 w716]
              tunnel: "Max Y (arena)" -> [w679 w715]
              tunnel: w526 -> [_ w713]
              tunnel: w524 -> [_ w712]
              frame False {
                # "New Position\nValid"
                # "Since no history available,\ncheck that current is within\nthe bounds of the arena size"
                # "Use Current Position bc \nPrevious are not available"
                n265 = In Range and Coerce(upper limit=w680, x=w683, lower limit=sgl 0.0 ("upper limit")) -> (In Range?=w686:bool)  [unwired: 1 out]
                n266 = In Range and Coerce(upper limit=w679, x=w682, lower limit=sgl 0.0 ("upper limit")) -> (In Range?=w685:bool)  [unwired: 1 out]
                n267 = Bundle(w683, w682) -> (w681:cluster{dbl, dbl})  [unwired: 1 in]
                n268 = And(x=w686, y=w685) -> (x .and. y?=w684:bool)
              }
              frame True {
                w714 = 0.0
                # "Change Y weight depending\non previous X position in course"
                # "If needed, make seperate FOR Loop for \nY only... Using more previous values than X"
                # "New Y"
                # "New X"
                # "Only consider if velocity is\ngreater than certain speed"
                # "Weighted Robot \nCoordinates"
                # "Position\nValid\n(current)"
                n269 = local read "Last Position"() -> (w692:cluster{"X":sgl, "Y":sgl})
                n270 = Unbundle By Name(w692) -> ("X"=w691:sgl)
                n271 = for {
                  N: w712 -> [_]
                  shift-right: [w730] -> w710
                  shift-left: w714 -> [w729]
                  shift-right: [w728] -> w695
                  shift-left: w714 -> [w727]
                  tunnel: w713 -> [w725] mode=indexing
                  tunnel: w711 -> [w723]
                  # "Fetch Last Valid Values\nand Sum"
                  n272 = Index Array(array=w723, index=w725) -> (element=w724:cluster{sgl, sgl})
                  n273 = Unbundle(w724) -> (w726:sgl, w722:sgl)
                  n274 = Add(x=w722, y=w727) -> (x+y=w728:dbl)
                  n275 = Add(x=w726, y=w729) -> (x+y=w730:dbl)
                }
                n276 = call "Scaling and Mapping"("Signals"=w691) -> ("Scaled Signals"=w690:dynamicdata)  [unwired: 9 in, 1 out]
                n277 = To Single Precision Float(number=w690) -> (single precision float=w689:sgl)
                "New Position\nWeight (Y coord)" <- w689
                n278 = Subtract(x=sgl 1.0, y="New Position\nWeight (X coord)") -> (x-y=w709:sgl)
                n279 = Subtract(x=sgl 1.0, y=w689) -> (x-y=w693:sgl)
                n280 = To Single Precision Float(number=w712) -> (single precision float=w701:sgl)
                n281 = Multiply(x=w709, y=w710) -> (x*y=w702:dbl)
                n282 = Multiply(x=w695, y=w693) -> (x*y=w703:dbl)
                n283 = Divide(x=w702, y=w701) -> (x/y=w699:dbl)
                n284 = Divide(x=w703, y=w701) -> (x/y=w700:dbl)
                n285 = Multiply(x="New Position\nWeight (X coord)", y=w707) -> (x*y=w705:dbl)
                n286 = Multiply(x=w694, y=w689) -> (x*y=w704:dbl)
                n287 = Add(x=w705, y=w699) -> (x+y=w698:dbl)
                n288 = Add(x=w704, y=w700) -> (x+y=w697:dbl)
                n289 = Greater Than 0?(x=w712) -> (x > 0?=w720:bool)
                n290 = case shown="True" w720 {
                  tunnel: w698 -> [w735 w742]
                  tunnel: w697 -> [w734 w741]
                  tunnel: w713 -> [_ w754]
                  tunnel: w711 -> [_ w753]
                  tunnel: [w732 w742] -> w719
                  tunnel: [w731 w741] -> w718
                  tunnel: [w736 w743] -> w717
                  tunnel: w716 -> [w738 _]
                  tunnel: w715 -> [w737 _]
                  frame False {
                    w733 = sgl 0.0 ("upper limit")
                    # "Check that within bounds of arena"
                    # "No Pevious is Available to Compare"
                    n291 = In Range and Coerce(upper limit=w738, x=w735, lower limit=w733) -> (In Range?=w740:bool)  [unwired: 1 out]
                    n292 = In Range and Coerce(upper limit=w737, x=w734, lower limit=w733) -> (In Range?=w739:bool)  [unwired: 1 out]
                    n293 = And(x=w740, y=w739) -> (x .and. y?=w736:bool)
                    n294 = Select(t=w735, s=w736, f=w733) -> (s? t:f=w732:dbl)
                    n295 = Select(t=w734, s=w736, f=w733) -> (s? t:f=w731:dbl)
                  }
                  frame True {
                    # "New"
                    # "(Y1 - Y2)^2"
                    # "(X1 - X2)^2"
                    # "Previous"
                    # "Pevious is Available to Compare"
                    n296 = Index Array(array=w754, index=u8 0) -> (element=w756:u8)
                    n297 = Index Array(array=w753, index=w756) -> (element=w755:cluster{sgl, sgl})
                    n298 = Unbundle(w755) -> (w745:sgl, w744:sgl)
                    n299 = Subtract(x=w745, y=w742) -> (x-y=w750:dbl)
                    n300 = Subtract(x=w741, y=w744) -> (x-y=w749:dbl)
                    n301 = Square(x=w750) -> (x^2=w748:dbl)
                    n302 = Square(x=w749) -> (x^2=w747:dbl)
                    n303 = Add(x=w748, y=w747) -> (x+y=w751:dbl)
                    n304 = Square Root(x=w751) -> (sqrt(x)=w746:dbl)
                    n305 = Less Or Equal?(x=w746, y="New Position \nThreshold") -> (x <= y?=w743:bool)
                  }
                }
                n306 = Bundle("upper limit"=w719, "upper limit"=w718) -> (w721:cluster{"upper limit":dbl, "upper limit":dbl})  [unwired: 1 in]
              }
            }
          }
        }
        "Orietnation\n(current)" <- w204
        n307 = local read "Current Template - Right"() -> (w139:T1)
        n308 = local read "Current Template - Left"() -> (w140:T1)
        n309 = Equal?(x=w140, y=w130) -> (x = y?=w137:bool)
        n310 = Equal?(x=w139, y=w130) -> (x = y?=w136:bool)
        n311 = Or(x=w137, y=w136) -> (x .or. y?=w138:bool)
        n312 = case shown="True" w138 {
          tunnel: [w230 w252] -> w143
          tunnel: [w229 w251] -> w141
          tunnel: w144 -> [w230 _]
          tunnel: w142 -> [w229 _]
          tunnel: [w228 w248] -> w145
          tunnel: w146 -> [w228 _]
          frame False {
            # "Disabled  -- ignore and pass all values thru"
          }
          frame True {
            w235 = 0 ("index")
            # "At Least 1?"
            # "# valid (0,1,2)"
            # "Only Stores in index\n0 for this special case"
            # "Curve Fitting for Range 0"
            # "Latch Y position"
            n313 = local read "Beacons Found\n- Left (Bool Array) 2"() -> (w268:bool[])
            n314 = local read "Beacons Found\n- Right (Bool Array)"() -> (w269:bool[])
            n315 = local read "Beacon Scales - Right"() -> (w260:sgl[])
            n316 = local read "Beacon Scales - Left"() -> (w261:sgl[])
            n317 = Index Array(array=w268, index=w235) -> (element=w267:bool)
            n318 = Index Array(array=w269, index=w235) -> (element=w262:bool)
            n319 = Index Array(array=w261, index=w235) -> (element=w232:sgl)
            n320 = Equal To 0?(x=w232) -> (x = 0?=w233:bool)
            n321 = Select(t=1.0, s=w233, f=w232) -> (s? t:f=w231:dbl)
            n322 = Index Array(array=w260, index=w235) -> (element=w237:sgl)
            n323 = Equal To 0?(x=w237) -> (x = 0?=w239:bool)
            n324 = Select(t=1.0, s=w239, f=w237) -> (s? t:f=w236:dbl)
            n325 = Power Of X(1:w236, 2:-0.826) -> (0:w247:dbl)
            n326 = Select(t=sgl 1.0, s=w267, f=sgl 0.0) -> (s? t:f=w259:sgl)
            n327 = Power Of X(1:w231, 2:-0.826) -> (0:w242:dbl)
            n328 = Select(t=sgl 1.0, s=w262, f=sgl 0.0) -> (s? t:f=w258:sgl)
            n329 = Multiply(x=93.909, y=w247) -> (x*y=w241:dbl)
            n330 = Multiply(x=w258, y=w241) -> (x*y=w256:dbl)
            n331 = Multiply(x=93.909, y=w242) -> (x*y=w240:dbl)
            n332 = Multiply(x=w259, y=w240) -> (x*y=w257:dbl)
            n333 = Add(x=w259, y=w258) -> (x+y=w253:sgl)
            n334 = Add(x=w257, y=w256) -> (x+y=w255:dbl)
            n335 = local read "Last Position"() -> (w270:cluster{"X":sgl, "Y":sgl})
            n336 = Greater Than 0?(x=w253) -> (x > 0?=w254:bool)
            n337 = case shown="True" w254 {
              selector: w254 -> [w271 w273]
              tunnel: w255 -> [_ w276]
              tunnel: w253 -> [_ w275]
              tunnel: [sgl 0.0 w274] -> w249
              tunnel: [w271 w273] -> w252
              tunnel: [w271 w273] -> w251
              frame False {
              }
              frame True {
                # "Avg Values"
                n338 = Divide(x=w276, y=w275) -> (x/y=w274:dbl)
              }
            }
            n339 = Unbundle(w270) -> ("Y"=w250:sgl)  [unwired: 1 out]
            n340 = Bundle(w249, "Y"=w250) -> (w248:cluster{dbl, "Y":sgl})  [unwired: 1 in]
          }
        }
        n341 = And(x=w143, y=w141) -> (x .and. y?=w134:bool)
        "Position Valid" <- w134
        n342 = Exclusive Or(1:w141, 2:w143) -> (0:w212:bool)
        n343 = case shown="True" w134 {
          tunnel: [w813 w816] -> w133
          tunnel: [w814 w815] -> w154
          tunnel: w223 -> [_ w816]
          tunnel: w145 -> [_ w815]
          tunnel: w212 -> [_ _]
          frame False {
            w813 = sgl 0.0 ("f")
            n344 = Bundle("f"=w813, "f"=w813) -> (w814:cluster{"f":sgl, "f":sgl})  [unwired: 1 in]
          }
          frame True {
            # "For Servos"
            n345 = shared-variable "RT myRIO Target - Overlord\\Localization_Variables_r0.lvlib\\Last Robot Position"(w815) -> ()  [unwired: 1 in, 1 out]
            "Last Orientation" <- w816
            "Last Position" <- w815
          }
        }
        "Robot Coordinates - Avgd" <- w154
        "Orientation Avgd" <- w133
        n346 = local read "History Size"() -> (w206:u8)
        n347 = Decrement(x=w206) -> (x-1=w207:u8)
        n348 = for {
          N: w206 -> [_]
          shift-right: [w854] -> w225
          shift-left: w222 -> [w853]
          tunnel: w154 -> [w852]
          tunnel: w207 -> [w851]
          i -> [w850]
          n349 = Subtract(x=w851, y=w850) -> (x-y=w849:i32)
          n350 = Equal To 0?(x=w849) -> (x = 0?=w848:bool)
          n351 = case shown="False" w848 {
            tunnel: w849 -> [w856 w861]
            tunnel: w853 -> [w859 w862]
            tunnel: [w857 w863] -> w854
            tunnel: w852 -> [_ w860]
            frame False {
              n352 = Decrement(x=w856) -> (x-1=w855:i32)
              n353 = Index Array(array=w859, index=w855) -> (element=w858:cluster{sgl, sgl})
              n354 = Replace Array Subset(array=w859, new element=w858, index=w856) -> (w857:cluster{sgl, sgl}[])
            }
            frame True {
              n355 = Replace Array Subset(array=w862, new element=w860, index=w861) -> (w863:cluster{sgl, sgl}[])
            }
          }
        }
        n356 = Unbundle(w154) -> ("upper limit"=w131:dbl, "upper limit"=w132:dbl)
        n357 = shared-variable "RT myRIO Target - Overlord\\Localization_Variables_r0.lvlib\\loc_theta"(w133) -> ()  [unwired: 1 in, 1 out]
        n358 = shared-variable "RT myRIO Target - Overlord\\Localization_Variables_r0.lvlib\\loc_flag"(w134) -> ()  [unwired: 1 in, 1 out]
        n359 = shared-variable "RT myRIO Target - Overlord\\Localization_Variables_r0.lvlib\\loc_y"(w132) -> ()  [unwired: 1 in, 1 out]
        n360 = shared-variable "RT myRIO Target - Overlord\\Localization_Variables_r0.lvlib\\loc_x"(w131) -> ()  [unwired: 1 in, 1 out]
        n361 = Decrement(x=w206) -> (x-1=w208:u8)
        n362 = for {
          N: w206 -> [_]
          shift-right: [w838] -> w226
          shift-left: w221 -> [w837]
          tunnel: w133 -> [w836]
          tunnel: w208 -> [w835]
          i -> [w834]
          n363 = Subtract(x=w835, y=w834) -> (x-y=w832:i32)
          n364 = Equal To 0?(x=w832) -> (x = 0?=w833:bool)
          n365 = case shown="False" w833 {
            tunnel: w832 -> [w840 w845]
            tunnel: w837 -> [w843 w846]
            tunnel: [w841 w847] -> w838
            tunnel: w836 -> [_ w844]
            frame False {
              # "Shift"
              n366 = Decrement(x=w840) -> (x-1=w839:i32)
              n367 = Index Array(array=w843, index=w839) -> (element=w842:sgl)
              n368 = Replace Array Subset(array=w843, new element=w842, index=w840) -> (w841:sgl[])
            }
            frame True {
              # "insert new"
              n369 = Replace Array Subset(array=w846, new element=w844, index=w845) -> (w847:sgl[])
            }
          }
        }
        n370 = Decrement(x=w206) -> (x-1=w205:u8)
        n371 = for {
          N: w206 -> [_]
          shift-right: [w823] -> w224
          shift-left: w220 -> [w822]
          tunnel: w134 -> [w821]
          tunnel: w205 -> [w820]
          i -> [w819]
          n372 = Subtract(x=w820, y=w819) -> (x-y=w817:i32)
          n373 = Equal To 0?(x=w817) -> (x = 0?=w818:bool)
          n374 = case shown="False" w818 {
            tunnel: w822 -> [w828 w830]
            tunnel: [w826 w831] -> w823
            tunnel: w821 -> [_ w829]
            tunnel: w817 -> [w824 _]
            frame False {
              n375 = Decrement(x=w824) -> (x-1=w825:i32)
              n376 = Index Array(array=w828, index=w825) -> (element=w827:bool)
              n377 = Replace Array Subset(array=w828, new element=w827, index=w824) -> (w826:bool[])
            }
            frame True {
              n378 = Replace Array Subset(array=w830, new element=w829) -> (w831:bool[])  [unwired: 1 in]
            }
          }
        }
        n379 = Boolean To (0,1)(Boolean=w224) -> (0, 1=w217:i16[])
        n380 = Add Array Elements(numeric array=w217) -> (sum=w216:i16)
        n381 = Greater Or Equal?(x=w216, y=i16 2) -> (x >= y?=w135:bool)
        "Position \nLock Status" <- w135
        n382 = case shown="True" w134 {
          tunnel: w154 -> [_ w812]
          frame False {
          }
          frame True {
            # "update debug graph\nif current is valid"
            n383 = Unbundle(w812) -> ("upper limit"=w811:dbl, "upper limit"=w810:dbl)
            n384 = Build Array(w810) -> (w808:dbl[])
            n385 = Build Array(w811) -> (w809:dbl[])
            n386 = Bundle(w809, w808) -> (→"Real Position in Course 2":cluster{dbl[], dbl[]})  [unwired: 1 in]
          }
        }
        n387 = shared-variable "RT myRIO Target - Overlord\\Localization_Variables_r0.lvlib\\Position_Lock"(w135) -> ()  [unwired: 1 in, 1 out]
        n388 = Unbundle By Name(w154) -> ("upper limit"=w151:dbl, "upper limit"=w153:dbl)
        n389 = Multiply(x=w151, y=w152) -> ()  [unwired: 1 out]
        n390 = Multiply(x=w153, y=w152) -> ()  [unwired: 1 out]
        n391 = Round Toward -Infinity(1:w151) -> (0:w150:dbl)
        n392 = Subtract(x=w151, y=w150) -> (x-y=w149:dbl)
        n393 = Multiply(x=w149, y=12.0) -> (x*y=→"inches":dbl)
      }
    }
    n394 = case shown="True" w113 {
      tunnel: w112 -> [_ w120]
      frame False {
      }
      frame True {
        n395 = call "Tick Count3"() -> ("Tick Count(uSec)"=w121:u32)
        n396 = Subtract(x=w121, y=w120) -> (x-y=w124:u32)
        n397 = Divide(x=w124, y=u32 1000 ("x")) -> (x/y=→"dT":dbl)
      }
    }
    n398 = call "Tick Count6"() -> ("Tick Count(uSec)"=w110:u32)
    "Robot Coordinates\nHistory" <- w109
    "Orientation\nHistory" <- w114
    "Position Valid\nHistory" <- w115
  }
  n399 = disable-structure shown="Enabled" {
    disable-tunnel: [w866 _] -> _
    disable-tunnel: ["Search Step Size\n(deg)" _] -> _
    frame Enabled {
      n400 = Multiply(x=3.413333333333333, y="Search Step Size\n(deg)") -> (x*y=w864:dbl)
      n401 = To Unsigned Word Integer(number=w864) -> (unsigned 16bit integer=w866:u16)
    }
    frame Disabled {
    }
  }
  n402 = Multiply(x="Move Servo\nThreshold (deg)", y=3.413333333333333) -> (x*y=w18:dbl)
  n403 = To Unsigned Word Integer(number=w18) -> ()  [unwired: 1 out]
  n404 = call "Tick Count8"() -> ()  [unwired: 1 out]
  n405 = flat-sequence {
    tunnel: [w870] -> w42
    tunnel: [w869] -> w41
    tunnel: [w874] -> w40
    tunnel: ["Left Servo\nID"] -> w29
    tunnel: ["Right Servo\nID"] -> w28
    tunnel: ["Compliance Slope"] -> w27
    tunnel: [w914] -> w39
    tunnel: [w913] -> w38
    tunnel: w42 -> [w912]
    tunnel: w41 -> [w911]
    tunnel: w40 -> [w910]
    tunnel: w29 -> [w908]
    tunnel: w28 -> [w907]
    tunnel: w27 -> [w906]
    tunnel: w39 -> [w1181]
    tunnel: w38 -> [w1180]
    frame #0 {
      # "BAUD RATE"
      # "Initialize UART and DIO"
      n406 = call-poly "VISA Configure Serial Port"("VISA resource name"=refnum<visa-resource-name> "ASRL1::INSTR", "Enable Termination\nChar (T)"=FALSE ("Enable Termination\nChar (T)"), "baud rate (9600)"=u32 115200) -> ("VISA resource name out"=w870:refnum<visa-resource-name>)  [unwired: 11 in, 1 out]
      n407 = call <vilib>:"Smart Open.vi"("Channel Names"=tag[] ["A/DIO2"]) -> ("DIO Ref Out"=w869:T9)  [unwired: 9 in, 1 out]
      n408 = flat-sequence {
        tunnel: w870 -> [w882]
        tunnel: w869 -> [w881]
        tunnel: "Left Servo\nID" -> [w883]
        tunnel: [w880] -> w871
        tunnel: "Compliance Slope" -> [w879]
        tunnel: "Right Servo\nID" -> [w896]
        tunnel: w871 -> [w895]
        tunnel: "Compliance Slope" -> [w894]
        tunnel: w870 -> [w893]
        tunnel: w869 -> [w892]
        frame #0 {
          w880 = 3
          n409 = while {
            tunnel: w880 -> [w889]
            tunnel: w882 -> [w887]
            tunnel: w881 -> [w886]
            tunnel: w883 -> [w885]
            tunnel: w879 -> [w884]
            i -> [w890]
            stop <- w888 stop-if-true
            n410 = call "Set_Compliance_Slope_R2.vi"("Compliance Slope"=w884, "DIO Ref Out"=w886, "VISA resource name"=w887, "Servo ID"=w885) -> ()  [unwired: 6 in, 2 out]
            n411 = Increment(x=w890) -> (x+1=w891:i32)
            n412 = Greater Or Equal?(x=w891, y=w889) -> (x >= y?=w888:bool)
          }
        }
        frame #1 {
          n413 = while {
            tunnel: w895 -> [w902]
            tunnel: w896 -> [w900]
            tunnel: w893 -> [w899]
            tunnel: w892 -> [w898]
            tunnel: w894 -> [w897]
            i -> [w903]
            stop <- w901 stop-if-true
            n414 = call "Set_Compliance_Slope_R2.vi"("Compliance Slope"=w897, "DIO Ref Out"=w898, "VISA resource name"=w899, "Servo ID"=w900) -> ()  [unwired: 6 in, 2 out]
            n415 = Increment(x=w903) -> (x+1=w904:i32)
            n416 = Greater Or Equal?(x=w904, y=w902) -> (x >= y?=w901:bool)
          }
        }
      }
      n417 = call "Tick Count"() -> ("Tick Count(uSec)"=w874:u32)
    }
    frame #1 {
      # "Service Count"
      n418 = while {
        shift-right: [w917] -> _
        shift-left: w910 -> [w934]
        tunnel: "Max Write\nTx Attempts" -> [w929]
        tunnel: "Max Read\nTx Attempts" -> [w928]
        shift-right: [w924] -> w914
        shift-left: w912 -> [w927]
        shift-right: [w923] -> w913
        shift-left: w911 -> [w926]
        tunnel: w908 -> [w922]
        tunnel: w907 -> [w921]
        tunnel: w906 -> [w920]
        shift-right: [w918] -> _
        shift-left: u16 0 -> [w919]
        stop <- "close comms" stop-if-true
        # "Loop Timer"
        n419 = local read "SERVO ENABLE"() -> (w916:bool)
        n420 = call "Tick Count2"() -> ("Tick Count(uSec)"=w917:u32)
        n421 = Subtract(x=w917, y=w934) -> (x-y=w933:u32)
        n422 = call "Wait4"("Count(mSec)"="Servo Comm\nLoop Time (ms)") -> ()  [unwired: 1 out]
        n423 = Divide(x=w933, y=u32 1000) -> (x/y=→"dT - Comm Loop":dbl)
        n424 = case shown="True" w916 {
          tunnel: w929 -> [_ w943]
          tunnel: w928 -> [_ w974]
          tunnel: w927 -> [w937 w938]
          tunnel: w926 -> [w936 w967]
          tunnel: [w937 w940] -> w924
          tunnel: [w936 w939] -> w923
          tunnel: w922 -> [_ w946]
          tunnel: w921 -> [_ w945]
          tunnel: w920 -> [_ w944]
          tunnel: w919 -> [_ w942]
          tunnel: [u16 100 w941] -> w918
          frame False {
            # "Restart at same value\nUsed to Periodically update \nCompliance Slope"
          }
          frame True {
            n425 = flat-sequence {
              tunnel: [w980] -> w978
              tunnel: [w981] -> w977
              tunnel: [w979] -> w976
              tunnel: w974 -> [w982]
              tunnel: [w984] -> w965
              tunnel: [w983] -> w963
              tunnel: w938 -> [w984]
              tunnel: w967 -> [w983]
              tunnel: w946 -> [w979]
              tunnel: w978 -> [w1002]
              tunnel: w977 -> [w1003]
              tunnel: w976 -> [w1001]
              tunnel: [w1001] -> w975
              tunnel: [w1000] -> w968
              tunnel: [w999] -> w966
              tunnel: w965 -> [w999]
              tunnel: [w998] -> w964
              tunnel: w963 -> [w998]
              tunnel: w975 -> [w1021]
              tunnel: w943 -> [w1020]
              tunnel: w968 -> [w1015]
              tunnel: w966 -> [w1017]
              tunnel: w964 -> [w1016]
              tunnel: [w1017] -> w961
              tunnel: [w1016] -> w959
              tunnel: [w1054] -> w962
              tunnel: w961 -> [w1054]
              tunnel: [w1053] -> w960
              tunnel: w959 -> [w1053]
              tunnel: ["Servo Comm\nWait Time - (ms)"] -> w951
              tunnel: w974 -> [w1061]
              tunnel: [w1060] -> w973
              tunnel: [w1059] -> w972
              tunnel: [w1055] -> w970
              tunnel: w962 -> [w1058]
              tunnel: w960 -> [w1057]
              tunnel: [w1058] -> w958
              tunnel: [w1057] -> w955
              tunnel: [w1056] -> w952
              tunnel: w951 -> [w1056]
              tunnel: w945 -> [w1055]
              tunnel: w973 -> [w1081]
              tunnel: w972 -> [w1080]
              tunnel: [w1079] -> w971
              tunnel: w970 -> [w1079]
              tunnel: [w1078] -> w969
              tunnel: w958 -> [w1077]
              tunnel: [w1077] -> w957
              tunnel: [w1076] -> w956
              tunnel: w955 -> [w1076]
              tunnel: w952 -> [w1075]
              tunnel: [w1075] -> w950
              tunnel: w971 -> [w1100]
              tunnel: w969 -> [w1098]
              tunnel: w943 -> [w1099]
              tunnel: w957 -> [w1097]
              tunnel: w956 -> [w1096]
              tunnel: [w1097] -> w954
              tunnel: [w1096] -> w953
              tunnel: w950 -> [w1093]
              tunnel: [w1093] -> w949
              tunnel: w954 -> [w1133]
              tunnel: w953 -> [w1132]
              tunnel: w949 -> [w1131]
              tunnel: [w1133] -> w948
              tunnel: [w1132] -> w947
              tunnel: w948 -> [w1137]
              tunnel: w947 -> [w1136]
              tunnel: w946 -> [w1142]
              tunnel: w945 -> [w1141]
              tunnel: w944 -> [w1140]
              tunnel: w942 -> [w1135]
              tunnel: w943 -> [w1139]
              tunnel: [w1138] -> w941
              tunnel: [w1137] -> w940
              tunnel: [w1136] -> w939
              frame #0 {
                n426 = while {
                  tunnel: [w997] -> w980
                  tunnel: w979 -> [w996]
                  tunnel: [w989] -> w981
                  tunnel: w982 -> [w987]
                  tunnel: w984 -> [w986]
                  tunnel: w983 -> [w985]
                  i -> [w988]
                  stop <- w990 stop-if-true
                  # "Attemp to Read Until\nMax Read Tx Attemps Limit"
                  n427 = call "ReadServo_R3.vi"("DIO Ref In"=w985, "VISA resource name out"=w986, "Servo ID"=w996) -> ("Error"=w993:u8, "Valid Checksum"=w994:bool, "Current Position"=w997:u64)  [unwired: 6 in]
                  n428 = Increment(x=w988) -> (x+1=w991:i32)
                  n429 = Equal To 0?(x=w993) -> (x = 0?=w995:bool)
                  n430 = Greater Or Equal?(x=w991, y=w987) -> (x >= y?=w992:bool)
                  n431 = And(x=w994, y=w995) -> (x .and. y?=w989:bool)
                  n432 = Or(x=w989, y=w992) -> (x .or. y?=w990:bool)
                }
              }
              frame #1 {
                # "Read Position First"
                n433 = local read "Servo Goal Position\n - Left"() -> (w1000:u16)
                n434 = case shown="True" w1003 {
                  tunnel: w1002 -> [_ w1005]
                  tunnel: w1000 -> [_ w1009]
                  frame False {
                  }
                  frame True {
                    # "Convert Received Position to Angle Relative to Robot"
                    n435 = local write "Current L (10bit)"(w1005) -> ()
                    n436 = local read "Mounting Offset - Left"() -> (w1007:sgl)
                    n437 = To Word Integer(number=w1005) -> (16bit integer=w1014:i16)
                    n438 = To Word Integer(number=w1009) -> (16bit integer=w1013:i16)
                    n439 = Subtract(x=w1013, y=w1014) -> (x-y=w1012:i16)
                    n440 = Absolute Value(x=w1012) -> (abs(x)=w1011:i16)
                    n441 = call "Servo_GP_Angle_Conversion_R0.vi"("GP in"=w1005, "Mode Select"=0, "Mount Offset"=w1007) -> ("Angle Out"=w1004:sgl)  [unwired: 7 in, 1 out]
                    n442 = Greater?(x=w1011, y=u16 5) -> (0:w1008:bool)
                    n443 = local write "Servo Moving - L"(w1008) -> ()
                    n444 = local write "Move Servo - L"(w1008) -> ()
                    n445 = local write "Current Angle\n - Left (internal)"(w1004) -> ()
                    n446 = shared-variable "RT myRIO Target - Overlord\\Localization_Variables_r0.lvlib\\Left Servo Angle_Current"(w1004) -> ()  [unwired: 1 in, 1 out]
                  }
                }
              }
              frame #2 {
                n447 = local read "Move Servo - L"() -> (w1018:bool)
                n448 = case shown="True" w1018 {
                  tunnel: w1021 -> [_ w1036]
                  tunnel: w1015 -> [_ w1023]
                  tunnel: [TRUE w1034] -> w1019
                  tunnel: w1020 -> [_ w1026]
                  tunnel: w1017 -> [_ w1025]
                  tunnel: w1016 -> [_ w1024]
                  frame False {
                    # "Only Send if Current Position is far enough"
                  }
                  frame True {
                    w1032 = 1
                    # "High Byte"
                    # "Low Byte"
                    n449 = Type Cast(type="", x=w1023) -> (*(type *) &x=w1033:string)
                    n450 = local write "Servo Moving - L"(TRUE) -> ()
                    n451 = String Subset(string=w1033, offset (0)=1, length (rest)=w1032) -> (substring=w1028:string)
                    n452 = String Subset(string=w1033, offset (0)=0, length (rest)=w1032) -> (substring=w1027:string)
                    n453 = while {
                      tunnel: w1036 -> [w1050]
                      tunnel: [w1042] -> w1034
                      tunnel: w1028 -> [w1046]
                      tunnel: w1027 -> [w1045]
                      tunnel: w1026 -> [w1039]
                      tunnel: w1025 -> [w1038]
                      tunnel: w1024 -> [w1037]
                      i -> [w1040]
                      stop <- w1041 stop-if-true
                      # "Attemp to Write Until\nMax Write Tx Attemps Limit"
                      n454 = call "MoveServo_R3.vi"("DIO Ref Out"=w1037, "VISA resource name out"=w1038, "GP - Low Byte"=w1046, "GP - High Byte"=w1045, "Servo ID"=w1050) -> ("Valid Checksum"=w1047:bool, "Error"=w1049:u64)  [unwired: 5 in]
                      n455 = Equal To 0?(x=w1049) -> (x = 0?=w1048:bool)
                      n456 = And(x=w1047, y=w1048) -> (x .and. y?=w1042:bool)
                      n457 = Increment(x=w1040) -> (x+1=w1044:i32)
                      n458 = Greater Or Equal?(x=w1044, y=w1039) -> (x >= y?=w1043:bool)
                      n459 = Or(x=w1042, y=w1043) -> (x .or. y?=w1041:bool)
                    }
                  }
                }
                n460 = case shown="True" w1019 {
                  frame False {
                  }
                  frame True {
                    # "Update Servo flag"
                    n461 = local write "Move Servo - L"(FALSE) -> ()
                  }
                }
              }
              frame #3 {
                n462 = call "Wait2"("Count(mSec)"="Servo Comm\nWait Time - (ms)") -> ()  [unwired: 1 out]
              }
              frame #4 {
                n463 = while {
                  tunnel: [w1074] -> w1060
                  tunnel: w1055 -> [w1073]
                  tunnel: [w1066] -> w1059
                  tunnel: w1061 -> [w1064]
                  tunnel: w1058 -> [w1063]
                  tunnel: w1057 -> [w1062]
                  i -> [w1065]
                  stop <- w1067 stop-if-true
                  # "Attemp to Read Until\nMax Read Tx Attemps Limit"
                  n464 = call "ReadServo_R3.vi"("DIO Ref In"=w1062, "VISA resource name out"=w1063, "Servo ID"=w1073) -> ("Error"=w1070:u8, "Valid Checksum"=w1071:bool, "Current Position"=w1074:u64)  [unwired: 6 in]
                  n465 = Increment(x=w1065) -> (x+1=w1068:i32)
                  n466 = Equal To 0?(x=w1070) -> (x = 0?=w1072:bool)
                  n467 = Greater Or Equal?(x=w1068, y=w1064) -> (x >= y?=w1069:bool)
                  n468 = And(x=w1071, y=w1072) -> (x .and. y?=w1066:bool)
                  n469 = Or(x=w1066, y=w1069) -> (x .or. y?=w1067:bool)
                }
              }
              frame #5 {
                n470 = local read "Servo Goal Position\n - Right"() -> (w1078:u16)
                n471 = case shown="True" w1080 {
                  tunnel: w1081 -> [_ w1083]
                  tunnel: w1078 -> [_ w1087]
                  frame False {
                    # "Don't update current position"
                  }
                  frame True {
                    # "Convert Received Position to Angle Relative to Robot"
                    n472 = local read "Mounting Offset - Right"() -> (w1085:sgl)
                    n473 = local write "Current R (10bit)"(w1083) -> ()
                    n474 = call "Servo_GP_Angle_Conversion_R0.vi"("GP in"=w1083, "Mode Select"=0, "Mount Offset"=w1085) -> ("Angle Out"=w1082:sgl)  [unwired: 7 in, 1 out]
                    n475 = To Word Integer(number=w1087) -> (16bit integer=w1091:i16)
                    n476 = local write "Current Angle\n - Right (internal)"(w1082) -> ()
                    n477 = To Word Integer(number=w1083) -> (16bit integer=w1092:i16)
                    n478 = shared-variable "RT myRIO Target - Overlord\\Localization_Variables_r0.lvlib\\Right Servo Angle_Current"(w1082) -> ()  [unwired: 1 in, 1 out]
                    n479 = Subtract(x=w1091, y=w1092) -> (x-y=w1090:i16)
                    n480 = Absolute Value(x=w1090) -> (abs(x)=w1089:i16)
                    n481 = Greater?(x=w1089, y=u16 5) -> (0:w1086:bool)
                    n482 = local write "Servo Moving - R"(w1086) -> ()
                    n483 = local write "Move Servo - R"(w1086) -> ()
                  }
                }
              }
              frame #6 {
                n484 = local read "Move Servo - R"() -> (w1094:bool)
                n485 = case shown="True" w1094 {
                  tunnel: w1098 -> [_ w1103]
                  tunnel: w1100 -> [_ w1110]
                  tunnel: [TRUE w1111] -> w1095
                  tunnel: w1099 -> [_ w1106]
                  tunnel: w1097 -> [_ w1105]
                  tunnel: w1096 -> [_ w1104]
                  frame False {
                  }
                  frame True {
                    w1113 = 1
                    # "High Byte"
                    # "Low Byte"
                    n486 = Type Cast(type="", x=w1103) -> (*(type *) &x=w1112:string)
                    n487 = local write "Servo Moving - R"(TRUE) -> ()
                    n488 = String Subset(string=w1112, offset (0)=1, length (rest)=w1113) -> (substring=w1109:string)
                    n489 = String Subset(string=w1112, offset (0)=0, length (rest)=w1113) -> (substring=w1108:string)
                    n490 = while {
                      tunnel: [w1122] -> w1111
                      tunnel: w1110 -> [w1127]
                      tunnel: w1109 -> [w1126]
                      tunnel: w1108 -> [w1125]
                      tunnel: w1106 -> [w1120]
                      tunnel: w1105 -> [w1118]
                      tunnel: w1104 -> [w1117]
                      i -> [w1121]
                      stop <- w1119 stop-if-true
                      # "Attemp to Write Until\nMax Write Tx Attemps Limit"
                      n491 = call "MoveServo_R3.vi"("DIO Ref Out"=w1117, "VISA resource name out"=w1118, "GP - Low Byte"=w1126, "GP - High Byte"=w1125, "Servo ID"=w1127) -> ("Valid Checksum"=w1129:bool, "Error"=w1128:u64)  [unwired: 5 in]
                      n492 = Increment(x=w1121) -> (x+1=w1123:i32)
                      n493 = Greater Or Equal?(x=w1123, y=w1120) -> (x >= y?=w1124:bool)
                      n494 = Equal To 0?(x=w1128) -> (x = 0?=w1130:bool)
                      n495 = And(x=w1129, y=w1130) -> (x .and. y?=w1122:bool)
                      n496 = Or(x=w1122, y=w1124) -> (x .or. y?=w1119:bool)
                    }
                  }
                }
                n497 = case shown="True" w1095 {
                  frame False {
                  }
                  frame True {
                    # "Update Servo flag"
                    n498 = local write "Move Servo - R"(FALSE) -> ()
                  }
                }
              }
              frame #7 {
                n499 = call "Wait3"("Count(mSec)"=w1131) -> ()  [unwired: 1 out]
              }
              frame #8 {
                # "Increment Service Count"
                # "Update Compliance Slope\nEvery x loops"
                n500 = Equal?(x=w1135, y=u16 1000) -> (x = y?=w1144:bool)
                n501 = case shown="True" w1144 {
                  tunnel: w1140 -> [_ w1154]
                  tunnel: w1137 -> [_ w1153]
                  tunnel: w1136 -> [_ w1152]
                  tunnel: w1137 -> [_ w1151]
                  tunnel: w1136 -> [_ w1150]
                  tunnel: w1142 -> [_ w1149]
                  tunnel: w1141 -> [_ w1148]
                  tunnel: w1135 -> [w1145 _]
                  tunnel: [w1145 u16 0] -> w1143
                  tunnel: w1139 -> [_ w1146]
                  frame False {
                  }
                  frame True {
                    # "Reset Service\nCount"
                    n502 = flat-sequence {
                      tunnel: w1153 -> [w1159]
                      tunnel: w1152 -> [w1158]
                      tunnel: w1149 -> [w1160]
                      tunnel: [w1156] -> w1155
                      tunnel: w1154 -> [w1157]
                      tunnel: w1146 -> [w1156]
                      tunnel: w1148 -> [w1172]
                      tunnel: w1155 -> [w1171]
                      tunnel: w1154 -> [w1170]
                      tunnel: w1151 -> [w1169]
                      tunnel: w1150 -> [w1168]
                      frame #0 {
                        n503 = while {
                          tunnel: w1156 -> [w1167]
                          tunnel: w1159 -> [w1165]
                          tunnel: w1158 -> [w1164]
                          tunnel: w1160 -> [w1163]
                          tunnel: w1157 -> [w1162]
                          i -> [w1161]
                          stop <- w1166 stop-if-true
                          n504 = call "Set_Compliance_Slope_R2.vi"("Compliance Slope"=w1162, "DIO Ref Out"=w1164, "VISA resource name"=w1165, "Servo ID"=w1163) -> ()  [unwired: 6 in, 2 out]
                          n505 = Greater Or Equal?(x=w1161, y=w1167) -> (x >= y?=w1166:bool)
                        }
                      }
                      frame #1 {
                        n506 = while {
                          tunnel: w1171 -> [w1179]
                          tunnel: w1172 -> [w1177]
                          tunnel: w1169 -> [w1176]
                          tunnel: w1168 -> [w1175]
                          tunnel: w1170 -> [w1174]
                          i -> [w1173]
                          stop <- w1178 stop-if-true
                          n507 = call "Set_Compliance_Slope_R2.vi"("Compliance Slope"=w1174, "DIO Ref Out"=w1175, "VISA resource name"=w1176, "Servo ID"=w1177) -> ()  [unwired: 6 in, 2 out]
                          n508 = Greater Or Equal?(x=w1173, y=w1179) -> (x >= y?=w1178:bool)
                        }
                      }
                    }
                  }
                }
                n509 = Increment(x=w1143) -> (x+1=w1138:u16)
              }
            }
          }
        }
      }
    }
    frame #2 {
      n510 = VISA Close(VISA resource name=w1181) -> ()  [unwired: 1 in, 1 out]
      n511 = call <vilib>:"Close.vi"("DIO Ref In"=w1180) -> ()  [unwired: 10 in, 1 out]
    }
  }
  n512 = while {
    stop <- FALSE stop-if-true
    n513 = call "Wait9"("Count(mSec)"=u32 1000) -> ()  [unwired: 1 out]
  }
  n514 = while {
    shift-right: [w1252] -> _
    shift-left: "Initial Main State - Left" -> [w1274]
    shift-right: [w1244] -> _
    shift-left: "Search Direction - in - L" -> [w1268]
    shift-right: [w1243] -> _
    shift-left: FALSE -> [w1267]
    shift-right: [w1246] -> _
    shift-left: w13 -> [w1245]
    shift-right: [w1247] -> _
    shift-left: w13 -> [w1261]
    shift-right: [w1248] -> _
    shift-left: w13 -> [w1266]
    shift-right: [w1249] -> _
    shift-left: w13 -> [w1260]
    shift-right: [w1250] -> _
    shift-left: w13 -> [w1259]
    shift-right: [w1196] -> _
    shift-left: "Search Direction - in - Right" -> [w1209]
    shift-right: [w1240] -> _
    shift-left: FALSE -> [w1207]
    shift-right: [w1241] -> _
    shift-left: w12 -> [w1198]
    shift-right: [w1195] -> _
    shift-left: w12 -> [w1197]
    shift-right: [w1194] -> _
    shift-left: w12 -> [w1204]
    shift-right: [w1193] -> _
    shift-left: w12 -> [w1206]
    shift-right: [w1192] -> _
    shift-left: w12 -> [w1205]
    shift-right: [w1184] -> _
    shift-left: "Initial Main State- Right" -> [w1221]
    shift-right: [w1236] -> _
    shift-left: 0 -> [w1238]
    shift-right: [w1188] -> _
    shift-left: 0 -> [w1213]
    shift-right: [w1235] -> _
    shift-left: "Initial Tracking State - Left" -> [w1237]
    shift-right: [w1190] -> _
    shift-left: "Initial Tracking State - Right" -> [w1219]
    shift-right: [w1189] -> _
    shift-left: "Initial Recovery State  - Right" -> [w1220]
    shift-right: [w1233] -> _
    shift-left: "Initial Recovery State - L" -> [w1234]
    stop <- FALSE stop-if-true
    w1228 = enum16{"Track", "Reactive Predict", ""}."Track" ("Initial Tracking State - Right")
    w1254 = T5."Tracking" ("Next Main State")
    # "Wait for New"
    # "ADD TRACKING TIMEOUT COUNT**********************"
    # "Service Track Angle Flag"
    # "Add Logic to Have Search Directions\nopposite if Both Searching"
    # "REMOVE LAST GOAL POSITION WITH cURRENT"
    # "Go to Current State"
    # "Add Logic to Have Search Directions\nopposite if Both Searching"
    # "Manuallly Reset\nRespond Var"
    # "Manuallly Reset\nRespond Var"
    # "Update Comm Process Variables"
    # "Both  inTracking (main state)"
    # "Current delta - L"
    # "delta move sum - R"
    # "delta move sum - L"
    # "Current delta - R"
    # "Service Move Respond Variables"
    n515 = local read "Min Num Frames\nper Search"() -> (w1242:i32)
    n516 = local read "Minimum Delta \nServo Threshold"() -> (w1258:i16)
    n517 = local read "Maximum Move \nServo Threshold"() -> (w1257:i16)
    n518 = local read "Middle Beacon\nCoordinates"() -> (w1199:cluster{"X":sgl, "Y":sgl})
    n519 = local read "Position \nLock Status"() -> (w1265:bool)
    n520 = local read "Position \nLock Status"() -> (w1202:bool)
    n521 = local read "Search Step Size"() -> (w1256:u16)
    n522 = local read "Last Orientation"() -> (w1263:sgl)
    n523 = local read "Last Orientation"() -> (w1200:sgl)
    n524 = local read "Last Position"() -> (w1264:cluster{"X":sgl, "Y":sgl})
    n525 = local read "Last Position"() -> (w1201:cluster{"X":sgl, "Y":sgl})
    n526 = local read "Min Num Frames\nper Search"() -> (w1203:i32)
    n527 = call "Wait"("Count(mSec)"="Servo Algorithm\nCycle Time(ms)") -> ()  [unwired: 1 out]
    n528 = local read "Minimum Delta \nServo Threshold"() -> (w1211:i16)
    n529 = local read "Maximum Move \nServo Threshold"() -> (w1210:i16)
    n530 = local read "Search Step Size"() -> (w1208:u16)
    n531 = local read "New Data  Flag\nRight Servo"() -> (w1216:bool)
    n532 = local read "New Data  Flag\nLeft Servo"() -> (w1232:bool)
    n533 = local read "Image Lock - Right"() -> (w1218:bool)
    n534 = local read "Tracking Angle - Right"() -> (w1215:sgl)
    n535 = local read "Image Lock - Left"() -> (w1273:bool)
    n536 = local read "Tracking Angle - Left"() -> (w1271:sgl)
    n537 = local read "Current R (10bit)"() -> (w1214:u16)
    n538 = local read "Current L (10bit)"() -> (w1270:u16)
    n539 = case shown="True" w1232 {
      tunnel: [w1786 w1824] -> w1276
      tunnel: [w1780 w1823] -> w1275
      tunnel: w1274 -> [w1781 w1822]
      tunnel: w1273 -> [_ w1821]
      tunnel: "Track Angle Valid - Left" -> [_ w1820]
      tunnel: w1271 -> [_ w1819]
      tunnel: w1270 -> [w1786 w1818]
      tunnel: "Mounting Offset - Left" -> [_ w1817]
      tunnel: w1268 -> [w1777 w1816]
      tunnel: w1267 -> [_ w1815]
      tunnel: w1266 -> [w1778 w1814]
      tunnel: w1265 -> [_ w1813]
      tunnel: w1264 -> [_ w1812]
      tunnel: w1263 -> [_ w1811]
      tunnel: "Middle Beacon\nCoordinates" -> [_ w1810]
      tunnel: w1261 -> [w1776 w1809]
      tunnel: w1260 -> [w1775 w1808]
      tunnel: w1259 -> [w1779 w1807]
      tunnel: w1258 -> [_ w1806]
      tunnel: w1257 -> [_ w1805]
      tunnel: w1256 -> [_ w1804]
      tunnel: [0 w1803] -> w1253
      tunnel: [w1781 w1802] -> w1252
      tunnel: [w1780 w1801] -> w1251
      tunnel: [w1779 w1800] -> w1250
      tunnel: [w1775 w1799] -> w1249
      tunnel: [w1778 w1798] -> w1248
      tunnel: [w1776 w1797] -> w1247
      tunnel: w1245 -> [_ w1796]
      tunnel: [w1777 w1795] -> w1244
      tunnel: w1242 -> [_ w1794]
      tunnel: w1238 -> [w1784 w1793]
      tunnel: w1237 -> [w1783 w1792]
      tunnel: [w1784 w1791] -> w1236
      tunnel: [w1783 w1790] -> w1235
      tunnel: w1234 -> [w1782 w1789]
      tunnel: [w1782 w1788] -> w1233
      frame False {
        w1780 = FALSE
        # "Recovery Mode COunt"
        # "Frames Processed - L"
        # "Recovery Search move Count - L"
        # "Recovery Search Attempt Count- L"
        # "WAITING FOR NEW IMAGE, RETAIN ALL VALUES"
      }
      frame True {
        w1826 = u16 1023
        w1829 = u16 0
        # "New Tracking State"
        # "Tracking Timeout Count"
        # "Next Main State"
        # "Next Recovery State"
        # "Reset Respond"
        # "Search Direction"
        # "Recovery Count"
        # "Recovery Search move Count"
        # "Recovery Search Attempt Count"
        # "Frames Processed"
        # "Apply Floor/Ceiling to Goal Position"
        # "Current move Delta"
        # "Service Track Angle Flag"
        # "Move Servo"
        # "Goal Position"
        # "Go to Current State"
        n540 = case shown="\"Recovery Mode\"" w1822 {
          tunnel: w1818 -> [w1847 w1923 w2091]
          tunnel: w1819 -> [_ w1925 _]
          tunnel: w1804 -> [w1846 _ w2086]
          tunnel: w1816 -> [w1845 w1906 w2080]
          tunnel: [w1844 w1921 w2090] -> w1830
          tunnel: [w1842 w1922 w2089] -> w1823
          tunnel: w1820 -> [_ w1916 w2067]
          tunnel: [w1840 w1918 w2076] -> w1802
          tunnel: w1821 -> [w1831 w1917 w2065]
          tunnel: w1817 -> [_ w1926 w2087]
          tunnel: w1806 -> [_ w1924 _]
          tunnel: [w1834 w1920 w2071] -> w1803
          tunnel: w1805 -> [_ w1919 _]
          tunnel: w1814 -> [w1839 _ w2081]
          tunnel: [enum16{"Generic Sweep", "Recovery Search"}."Recovery Search" enum16{"Generic Sweep", "Recovery Search"}."Recovery Search" w2088] -> w1788
          tunnel: w1809 -> [_ _ w2085]
          tunnel: w1789 -> [_ _ w2068]
          tunnel: w1815 -> [_ w1903 w2097]
          tunnel: w1796 -> [_ w1899 w2092]
          tunnel: w1811 -> [_ w1909 w2094]
          tunnel: w1812 -> [_ w1910 w2095]
          tunnel: w1813 -> [_ w1911 w2096]
          tunnel: w1810 -> [_ w1908 w2093]
          tunnel: [FALSE w1905 w2069] -> w1801
          tunnel: w1794 -> [w1838 _ w2079]
          tunnel: [w1834 w1900 w2078] -> w1797
          tunnel: [w1834 w1900 w2084] -> w1800
          tunnel: [w1834 w1900 w2083] -> w1799
          tunnel: [w1837 w1901 w2082] -> w1798
          tunnel: w1808 -> [_ _ w2074]
          tunnel: w1807 -> [_ _ w2073]
          tunnel: [w1835 w1906 w2072] -> w1795
          tunnel: w1793 -> [_ w1915 _]
          tunnel: [w1834 w1907 w2071] -> w1791
          tunnel: w1792 -> [_ w1912 _]
          tunnel: [enum16{"Track", "Reactive Predict", ""}."Track" ("Initial Tracking State - Right") w1904 enum16{"Track", "Reactive Predict", ""}."Track" ("Initial Tracking State - Right")] -> w1790
          frame "Start Up Search", Default {
            w1834 = u16 0
            # "Image Lock"
            # "Search Direction"
            # "Wait for 'x' Images to be Processed\nBefore Going to Next Step"
            # "Next Main State"
            # "New Goal Position"
            # "Move Servo"
            # "Choose Next State"
            # "Frames Processed Count"
            n541 = Greater Or Equal?(x=w1839, y=w1838) -> (x >= y?=w1843:bool)
            n542 = case shown="True" w1843 {
              tunnel: w1847 -> [w1857 w1873]
              tunnel: w1846 -> [_ w1871]
              tunnel: w1845 -> [w1856 w1870]
              tunnel: [w1857 w1863] -> w1844
              tunnel: [w1855 0] -> w1837
              tunnel: [FALSE TRUE] -> w1841
              tunnel: w1839 -> [w1858 _]
              tunnel: [w1856 w1864] -> w1835
              frame False {
                # "Wait until Min Number of Frames (per search/step) Processed"
                # "Increase Frames\nProcessed Count"
                n543 = Increment(x=w1858) -> (x+1=w1855:i32)
              }
              frame True {
                # "Reset Frames\nProcessed Count"
                # "SWEEP SEARCH - Startup"
                # "Multiple New Step\nby Step SIze"
                # "F = CCW\nT = CW"
                # "Last Direction"
                # "Min Step"
                # "add in case\nactual position\nis lower than GP"
                # "Set New Step #"
                # "Choose Direction"
                # "Nearest step"
                # "Adjust Actual Posiiton\n to pre-determiend steps"
                # "Move Servo 1 \"Step\" to\nSearch"
                n544 = Subtract(x=w1873, y=u16 200) -> (x-y=w1861:u16)
                n545 = Add(x=10, y=w1861) -> (x+y=w1879:i32)
                n546 = Quotient & Remainder(x=w1879, y=w1871) -> (floor(x/y)=w1877:i32)  [unwired: 1 out]
                n547 = To Byte Integer(number=w1877) -> (8bit integer=w1868:i8)
                n548 = Less?(x=w1868, y=1) -> (x < y?=w1874:bool)
                n549 = case shown="False" w1874 {
                  tunnel: w1868 -> [w1890 w1898]
                  tunnel: [w1892 FALSE] -> w1864
                  tunnel: [w1891 w1898] -> w1876
                  tunnel: w1870 -> [w1889 _]
                  tunnel: w1871 -> [w1887 _]
                  frame False {
                    # "Max Step"
                    # "# of steps\nminus 1"
                    n550 = Divide(x=300, y=w1887) -> (x/y=w1884:dbl)
                    n551 = To Unsigned Byte Integer(number=w1884) -> (unsigned 8bit integer=w1885:u8)
                    n552 = Greater Or Equal?(x=w1890, y=w1885) -> (x >= y?=w1886:bool)
                    n553 = case shown="True" w1886 {
                      tunnel: [w1893 TRUE] -> w1892
                      tunnel: [w1894 w1895] -> w1891
                      tunnel: w1890 -> [w1894 w1895]
                      tunnel: w1889 -> [w1893 _]
                      frame False {
                        # "No Need to\nChange Direction"
                      }
                      frame True {
                        # "T"
                        # "Move CW"
                      }
                    }
                  }
                  frame True {
                    # "F"
                    # "Move CCW"
                  }
                }
                n554 = case shown="False" w1864 {
                  tunnel: w1876 -> [w1881 w1882]
                  tunnel: [w1880 w1883] -> w1872
                  frame False {
                    # "CCW\n+1"
                    n555 = Increment(x=w1881) -> (x+1=w1880:i8)
                  }
                  frame True {
                    # "CW\n-1"
                    n556 = Decrement(x=w1882) -> (x-1=w1883:i8)
                  }
                }
                n557 = Multiply(x=w1872, y=w1871) -> (x*y=w1869:u16)
                n558 = To Unsigned Word Integer(number=w1869) -> (unsigned 16bit integer=w1867:u16)
                n559 = Add(x=w1867, y=u16 200) -> (x+y=w1863:u16)
              }
            }
            n560 = case shown="False" w1831 {
              tunnel: [w1849 FALSE] -> w1842
              tunnel: w1841 -> [w1849 _]
              tunnel: [w1850 T5."Tracking" ("Next Main State")] -> w1840
              frame False {
                # "Check other Servo\nStay in Startup  State"
                n561 = local read "Image Lock - Right"() -> (w1848:bool)
                n562 = case shown="False" w1848 {
                  tunnel: [T5."Start Up Search" ("Next Main State") T5."Recovery Mode" ("Next Main State")] -> w1850
                  frame False {
                  }
                  frame True {
                  }
                }
              }
              frame True {
                # "Override Move Servo\nCommand bc an Angle Was Found\nduring this Step"
                # "Transition to Tracking State When\nImage Processing has Locked"
              }
            }
          }
          frame "Tracking" {
            w1900 = 0
            # "Frames Processed Count"
            # "Image Lock - L"
            # "Track Angle Valid"
            # "Tracking Angle"
            # "Tracking Timeout Count"
            # "Max ove delta"
            # "Move delta threshold"
            # "mount offset"
            # "Current Position"
            # "Move Respond"
            # "Trackin Timeout count"
            # "Move Servo"
            # "delta"
            # "GP"
            # "Reset Move Respond"
            # "New Tracking State"
            # "Delta Move Sum"
            # "Choose Next State"
            n563 = case shown="\"Track\", Default" w1912 {
              tunnel: w1926 -> [w1944 _]
              tunnel: w1925 -> [w1943 _]
              tunnel: w1924 -> [w1942 _]
              tunnel: w1923 -> [w1941 w1989]
              tunnel: [w1940 w1987] -> w1922
              tunnel: [w1939 w1995] -> w1921
              tunnel: [w1938 0] -> w1920
              tunnel: w1919 -> [w1937 _]
              tunnel: w1917 -> [w1936 w1979]
              tunnel: w1916 -> [w1935 w1982]
              tunnel: w1915 -> [w1934 w1984]
              tunnel: w1911 -> [_ w1994]
              tunnel: w1910 -> [_ w1993]
              tunnel: w1909 -> [_ w1992]
              tunnel: w1908 -> [_ w1991]
              tunnel: w1903 -> [_ w1990]
              tunnel: w1899 -> [_ w1988]
              tunnel: [TRUE w1985] -> w1905
              tunnel: [w1931 w1983] -> w1907
              tunnel: [w1929 w1981] -> w1904
              tunnel: [0 0] -> w1901
              frame "Track", Default {
                # "Reset"
                # "Tracking Timeout"
                # "Move Delta"
                # "Goal Position"
                # "Tracking Move"
                # "Move Servo"
                # "Only Consider Tracking Angle\n\nIF\n\nImage Locked        == T\nTrack Angle Flag   == T"
                n564 = And(x=w1936, y=w1935) -> (x .and. y?=w1928:bool)
                n565 = case shown="True" w1928 {
                  tunnel: w1944 -> [_ w1952]
                  tunnel: w1943 -> [_ w1950]
                  tunnel: w1942 -> [_ w1967]
                  tunnel: w1941 -> [w1947 w1957]
                  tunnel: [w1947 w1966] -> w1939
                  tunnel: [w1949 w1965] -> w1940
                  tunnel: [w1949 w1964] -> _
                  tunnel: [u16 0 w1963] -> w1938
                  tunnel: w1937 -> [_ w1959]
                  tunnel: w1934 -> [w1946 _]
                  tunnel: [w1945 0] -> w1931
                  frame False {
                    w1949 = FALSE
                    # "Increment timeout"
                    n566 = Increment(x=w1946) -> (x+1=w1945:i32)
                  }
                  frame True {
                    # "******"
                    # "Move to Tracking Angle \n\nif delta is greater than move servo threshold\nAND less than max move threshold"
                    n567 = call "Servo_GP_Angle_Conversion_R0.vi"("Angle In"=w1950, "Mode Select"=1, "Mount Offset"=w1952) -> ("GP out"=w1951:u16)  [unwired: 7 in, 1 out]
                    n568 = To Word Integer(number=w1957) -> (16bit integer=w1955:i16)
                    n569 = To Word Integer(number=w1951) -> (16bit integer=w1968:i16)
                    n570 = Subtract(x=w1968, y=w1955) -> (x-y=w1958:i16)
                    n571 = Absolute Value(x=w1958) -> (abs(x)=w1954:i16)
                    n572 = Greater Or Equal?(x=w1954, y=w1967) -> (x >= y?=w1961:bool)
                    n573 = Less Or Equal?(x=w1954, y=w1959) -> (x <= y?=w1960:bool)
                    n574 = And(x=w1961, y=w1960) -> (x .and. y?=w1962:bool)
                    n575 = case shown="True" w1962 {
                      tunnel: w1951 -> [_ w1973]
                      tunnel: [w1970 w1973] -> w1966
                      tunnel: [w1971 w1975] -> w1965
                      tunnel: [w1971 w1975] -> w1964
                      tunnel: w1957 -> [w1970 _]
                      tunnel: w1954 -> [_ w1974]
                      tunnel: [u16 0 w1974] -> w1963
                      tunnel: w1950 -> [_ w1972]
                      frame False {
                        w1971 = FALSE
                        # "Don't Move"
                      }
                      frame True {
                        w1975 = TRUE
                        # "1024/300"
                        # "Current Delta"
                        # "Use new Track Angle"
                        n576 = local write "Last Track Angle - L"(w1972) -> ()
                      }
                    }
                  }
                }
                n577 = local read "Timeout to \nEnable Reactive Predict"() -> (w1932:u16)
                n578 = Less?(x=w1931, y=w1932) -> (x < y?=w1930:bool)
                n579 = case shown="True" w1930 {
                  tunnel: [enum16{"Track", "Reactive Predict", ""}."Reactive Predict" ("Initial Tracking State - Right") enum16{"Track", "Reactive Predict", ""}."Track" ("Initial Tracking State - Right")] -> w1929
                  frame False {
                  }
                  frame True {
                  }
                }
              }
              frame "Reactive Predict" {
                # "Choose New\nTracking State"
                n580 = Or(x=w1979, y=w1982) -> (x .or. y?=w1978:bool)
                n581 = case shown="False" w1978 {
                  tunnel: [w2008 w2061] -> w1995
                  tunnel: w1994 -> [w2007 _]
                  tunnel: w1993 -> [w2006 _]
                  tunnel: w1992 -> [w2005 _]
                  tunnel: w1991 -> [w2004 _]
                  tunnel: w1990 -> [w2003 _]
                  tunnel: w1988 -> [w2002 _]
                  tunnel: [w2001 FALSE] -> w1987
                  tunnel: [w2000 TRUE] -> w1985
                  tunnel: w1984 -> [w1999 _]
                  tunnel: [w1998 0] -> w1983
                  tunnel: [enum16{"Track", "Reactive Predict", ""}."Reactive Predict" ("Initial Tracking State - Right") enum16{"Track", "Reactive Predict", ""}."Track" ("Initial Tracking State - Right")] -> w1981
                  tunnel: w1989 -> [w1996 w2061]
                  frame False {
                    # "Stay in Reactive State"
                    # "Increment Track Timeout"
                    # "Move Respond Flag"
                    n582 = Increment(x=w1999) -> (x+1=w1998:i32)
                    n583 = case shown="True" w2003 {
                      tunnel: w2007 -> [_ w2023]
                      tunnel: w2006 -> [_ w2022]
                      tunnel: w2005 -> [_ w2021]
                      tunnel: w2004 -> [_ w2020]
                      tunnel: w2002 -> [_ w2017]
                      tunnel: [w2009 w2013] -> w2008
                      tunnel: [w2010 w2012] -> w2001
                      tunnel: [w2010 w2012] -> w2000
                      tunnel: w1996 -> [w2009 w2011]
                      frame False {
                        w2010 = FALSE
                        # "Reset Move Respond = F"
                        # "Move Servo = F"
                      }
                      frame True {
                        w2012 = TRUE
                        # "Position Lock"
                        # "Current Servo\nPosition"
                        # "Reset Move\nRespond = T"
                        # "Move Servo = T"
                        # "Apply Direction \nto Offset (delta sum)"
                        # "Check Last Known Position of Robot"
                        n584 = case shown="True" w2023 {
                          tunnel: w2022 -> [_ w2051]
                          tunnel: w2021 -> [_ w2026]
                          tunnel: w2020 -> [_ w2027]
                          tunnel: [sgl 1.0 ("y") w2025] -> w2019
                          frame False {
                            # "No Position Data Available"
                            # "Default is to move\nSame Direction as other\nServo"
                          }
                          frame True {
                            w2032 = sgl 1.0 ("y")
                            # "Use previous position/orientation to Guess Which Direction to Move Servo"
                            # "Choose Search Direction"
                            # "\"Perpendicular \nThreshold\""
                            # "If Orientation is\n ~Perpendicular -> Start Search\n in Opposite Direction of Other"
                            # "****add 90 until orientation angle is fixed"
                            # "Last Orientation"
                            # "Convert to Rad"
                            # "Avoid Divide by 0"
                            # "-1/m"
                            # "Calculate Normal Line to \nLast Robot Position\nfrom Center Beacon"
                            # "last Position \nCoordinates"
                            n585 = Unbundle(w2051) -> ("X"=w2031:sgl, "Y"=w2030:sgl)
                            n586 = Unbundle(w2027) -> ("X"=w2029:sgl, "Y"=w2028:sgl)
                            n587 = Subtract(x=w2030, y=w2028) -> (x-y=w2047:sgl)
                            n588 = Subtract(x=w2031, y=w2029) -> (x-y=w2045:sgl)
                            n589 = Equal To 0?(x=w2045) -> (x = 0?=w2046:bool)
                            n590 = case shown="False" w2046 {
                              tunnel: w2047 -> [w2054 _]
                              tunnel: w2045 -> [w2053 _]
                              tunnel: [w2052 1000000000000000.0] -> w2044
                              frame False {
                                n591 = Divide(x=w2054, y=w2053) -> (x/y=w2052:sgl)
                              }
                              frame True {
                              }
                            }
                            n592 = Equal To 0?(x=w2044) -> (x = 0?=w2049:bool)
                            n593 = case shown="False" w2049 {
                              tunnel: [w2056 1e-08] -> w2048
                              tunnel: w2044 -> [w2056 _]
                              frame False {
                              }
                              frame True {
                                # "Can't have infinit slope"
                              }
                            }
                            n594 = Divide(x=-1.0, y=w2048) -> (x/y=w2043:dbl)
                            n595 = Inverse Tangent(1:w2043) -> (0:w2041:dbl)
                            n596 = expression code="(x/pi)*180.0" "radians to degrees"(w2041) -> (w2042:dbl)
                            n597 = To Single Precision Float(number=w2042) -> (single precision float=w2039:sgl)
                            n598 = Add(x=w2026, y=sgl 90.0) -> (x+y=w2038:sgl)
                            n599 = Subtract(x=w2039, y=w2038) -> (x-y=w2037:sgl)
                            n600 = Absolute Value(x=w2037) -> (abs(x)=w2036:sgl)
                            n601 = Less Or Equal?(x=w2036, y=sgl 10.0) -> (x <= y?=w2034:bool)
                            n602 = Negate(x=w2032) -> (-x=w2033:sgl)
                            n603 = Select(t=w2033, s=w2034, f=w2032) -> (s? t:f=w2025:sgl)
                          }
                        }
                        n604 = To Word Integer(number=w2019) -> (16bit integer=w2018:i16)
                        n605 = Multiply(x=w2018, y=w2017) -> (x*y=w2016:i32)
                        n606 = To Word Integer(number=w2011) -> (16bit integer=w2015:i16)
                        n607 = Add(x=w2016, y=w2015) -> (x+y=w2014:i32)
                        n608 = To Unsigned Word Integer(number=w2014) -> (unsigned 16bit integer=w2013:u16)
                      }
                    }
                  }
                  frame True {
                    # "Either Current Angle Valid or Image Lock Acheived"
                    # "Go Directly to Track State"
                  }
                }
              }
            }
            n609 = local read "Tracking Timeout\nThreshold"() -> (w1913:i32)
            n610 = Less?(x=w1907, y=w1913) -> (x < y?=w1914:bool)
            n611 = case shown="True" w1914 {
              tunnel: [T5."Recovery Mode" ("Next Main State") T5."Tracking" ("Next Main State")] -> w1918
              frame False {
              }
              frame True {
              }
            }
          }
          frame "Recovery Mode" {
            w2071 = u16 0
            # "Recovery Search Move Count"
            # "***Compltetly resets as of R17, used to just reset to \"Max Recovery Count - 1\""
            # "Increment Recoveyr Mode Count"
            # "Frames Processed"
            # "Choose Next Main State"
            # "Reset recovery count"
            # "Recovery move\nCount"
            # "Recovery Search\nAttempt count"
            # "Move Servo = T"
            # "delta move sum"
            # "Robot Position Valid"
            n612 = local read "Image Lock - Right"() -> (w2075:bool)
            n613 = case shown="\"Recovery Search\"" w2068 {
              tunnel: w2097 -> [_ _]
              tunnel: w2096 -> [_ _]
              tunnel: w2095 -> [_ _]
              tunnel: w2094 -> [_ _]
              tunnel: w2093 -> [_ _]
              tunnel: w2092 -> [_ _]
              tunnel: w2091 -> [w2125 w2205]
              tunnel: [w2117 w2203] -> w2090
              tunnel: [w2114 w2197] -> w2089
              tunnel: [FALSE FALSE] -> w2069
              tunnel: [w2119 w2195] -> w2088
              tunnel: w2085 -> [w2123 _]
              tunnel: w2087 -> [w2126 _]
              tunnel: w2086 -> [w2124 w2200]
              tunnel: [w2116 w2194] -> w2083
              tunnel: [w2115 w2194] -> w2084
              tunnel: w2075 -> [w2113 _]
              tunnel: [w2104 w2204] -> w2082
              tunnel: w2081 -> [w2102 w2192]
              tunnel: w2080 -> [w2107 w2201]
              tunnel: w2079 -> [w2103 w2199]
              tunnel: w2065 -> [_ _]
              tunnel: w2067 -> [_ _]
              tunnel: [FALSE w2196] -> w2077
              tunnel: w2074 -> [w2111 _]
              tunnel: w2073 -> [w2110 _]
              tunnel: [w2107 w2193] -> w2072
              tunnel: w2065 -> [_ w2190]
              frame "Recovery Search" {
                # "Wait for 2 Images to be Processed\nBefore Going to Next Step"
                # "Choose Next Reovery State"
                # "Recovery Search \nAttempt Count"
                # "Move Servo"
                # "Goal Position"
                # "Recovery Search\nmove Count"
                # "Attempt Recovery Search if Other Servo has Valid Angle"
                n614 = local read "Last Track Angle - R"() -> (w2106:sgl)
                n615 = Greater Or Equal?(x=w2102, y=w2103) -> (x >= y?=w2105:bool)
                n616 = case shown="True" w2105 {
                  tunnel: w2126 -> [_ w2146]
                  tunnel: [w2131 w2145] -> w2115
                  tunnel: w2125 -> [w2134 w2144]
                  tunnel: w2124 -> [_ w2143]
                  tunnel: [w2132 w2142] -> w2116
                  tunnel: [w2134 w2141] -> w2117
                  tunnel: [FALSE w2140] -> w2114
                  tunnel: w2111 -> [w2132 w2139]
                  tunnel: w2110 -> [w2131 w2138]
                  tunnel: w2113 -> [_ w2137]
                  tunnel: w2106 -> [_ w2136]
                  tunnel: [w2129 0 ("Frames Processed\nCount - in")] -> w2104
                  tunnel: w2102 -> [w2130 _]
                  frame False {
                    # "Increment Frames Processed"
                    # "WAIT"
                    n617 = Increment(x=w2130) -> (x+1=w2129:i32)
                  }
                  frame True {
                    n618 = case shown="True" w2137 {
                      tunnel: w2136 -> [_ w2159]
                      tunnel: w2139 -> [w2147 w2155]
                      tunnel: w2146 -> [_ w2160]
                      tunnel: [w2150 w2158] -> w2141
                      tunnel: [w2148 w2157] -> w2145
                      tunnel: w2138 -> [w2148 w2156]
                      tunnel: w2144 -> [w2150 w2154]
                      tunnel: w2143 -> [_ w2153]
                      tunnel: [FALSE TRUE] -> w2140
                      tunnel: [w2147 w2151] -> w2142
                      frame False {
                        # "Don't Move bc Other Servo Doesn't Have Image Lock"
                      }
                      frame True {
                        # "Move Servo = T"
                        n619 = Greater Than 0?(x=w2155) -> (x > 0?=w2161:bool)
                        n620 = case shown="False" w2161 {
                          tunnel: w2160 -> [w2162 _]
                          tunnel: w2159 -> [w2163 _]
                          tunnel: [w2166 w2174] -> w2158
                          tunnel: [w2170 w2180] -> w2157
                          tunnel: w2156 -> [w2171 w2180]
                          tunnel: w2155 -> [w2169 w2177]
                          tunnel: [w2168 w2179] -> w2151
                          tunnel: w2154 -> [_ w2175]
                          tunnel: w2153 -> [_ w2172]
                          frame False {
                            # "************************"
                            # "Increment move count to transition\nto Pan mode"
                            # "Increment Recovery Search Attempt Count"
                            # "Move Parallel to Other Servo"
                            n621 = Increment(x=w2171) -> (x+1=w2170:i32)
                            n622 = call "Servo_GP_Angle_Conversion_R0.vi"("Angle In"=w2163, "Mode Select"=1, "Mount Offset"=w2162) -> ("GP out"=w2164:u16)  [unwired: 7 in, 1 out]
                            n623 = Increment(x=w2169) -> (x+1=w2168:i32)
                            n624 = Add(x=w2164, y="Recovery Parallel\nSearch Offset") -> (x+y=w2166:u16)
                          }
                          frame True {
                            # "Apply Direction"
                            # "Step SIze"
                            # "Current Position"
                            # "Attempt to Pan in Steps Towards other Servo"
                            # "Could be same or function of \nregular search step size"
                            # "Max # of Pan\nMoves"
                            # "Pan Towards Other Servo"
                            n625 = Greater Or Equal?(x=w2177, y="Max # Pan Moves") -> (x >= y?=w2178:bool)
                            n626 = case shown="False" w2178 {
                              tunnel: w2177 -> [w2188 _]
                              tunnel: [w2187 u16 0] -> w2179
                              frame False {
                                # "Increment Pan Count"
                                n627 = Increment(x=w2188) -> (x+1=w2187:i32)
                              }
                              frame True {
                                # "Reset move count"
                              }
                            }
                            n628 = local read "Recovery Search\nDirection - L"() -> (w2173:bool)
                            n629 = case shown="True" w2173 {
                              tunnel: w2175 -> [w2182 w2186]
                              tunnel: w2172 -> [w2183 w2185]
                              tunnel: [w2181 w2184] -> w2174
                              frame False {
                                # "CCW"
                                n630 = Add(x=w2182, y=w2183) -> (x+y=w2181:u16)
                              }
                              frame True {
                                # "CW"
                                n631 = Subtract(x=w2186, y=w2185) -> (x-y=w2184:u16)
                              }
                            }
                          }
                        }
                      }
                    }
                  }
                }
                n632 = local read "Max Recovery Count\n(Recovery Search)"() -> (w2108:u16)
                n633 = local read "Max Recovery\nSearch Attempts"() -> (w2109:u16)
                n634 = Less Or Equal?(x=w2115, y=w2109) -> (x <= y?=w2121:bool)
                n635 = Less Or Equal?(x=w2123, y=w2108) -> (x <= y?=w2122:bool)
                n636 = And(x=w2121, y=w2122) -> (x .and. y?=w2120:bool)
                n637 = case shown="True" w2120 {
                  tunnel: [enum16{"Generic Sweep", "Recovery Search"}."Generic Sweep" enum16{"Generic Sweep", "Recovery Search"}."Recovery Search"] -> w2119
                  frame False {
                  }
                  frame True {
                  }
                }
              }
              frame "Generic Sweep" {
                w2194 = u16 0
                # "Image Locked?"
                # "Choose Next Recovery State"
                # "Wait for 2 Images to be Processed\nBefore Going to Next Step"
                # "New Goal Position"
                # "Move Servo"
                # "Frames Processed Count"
                n638 = Greater Or Equal?(x=w2192, y=w2199) -> (x >= y?=w2206:bool)
                n639 = case shown="True" w2206 {
                  tunnel: w2205 -> [w2222 w2238]
                  tunnel: w2200 -> [_ w2236]
                  tunnel: w2201 -> [w2221 w2235]
                  tunnel: [w2222 w2226] -> w2203
                  tunnel: [w2220 0] -> w2204
                  tunnel: [FALSE TRUE] -> w2198
                  tunnel: w2192 -> [w2223 _]
                  tunnel: [w2221 w2229] -> w2193
                  frame False {
                    # "Increment Frames Processed"
                    n640 = Increment(x=w2223) -> (x+1=w2220:i32)
                  }
                  frame True {
                    # "Reset Frames\nProcessed Count"
                    # "SWEEP SEARCH - Startup"
                    # "Multiple New Step\nby Step SIze"
                    # "F = CCW\nT = CW"
                    # "Last Direction"
                    # "Min Step"
                    # "add 10 in case\nactual position\nis lower than GP"
                    # "Set New Step #"
                    # "Choose Direction"
                    # "Nearest step"
                    # "Adjust Actual Posiiton\n to pre-determiend steps"
                    # "Move Servo 1 \"Step\" to\nSearch"
                    n641 = Subtract(x=w2238, y=200) -> (x-y=w2228:i32)
                    n642 = Add(x=5, y=w2228) -> (x+y=w2244:i32)
                    n643 = Quotient & Remainder(x=w2244, y=w2236) -> (floor(x/y)=w2242:i32)  [unwired: 1 out]
                    n644 = To Byte Integer(number=w2242) -> (8bit integer=w2233:i8)
                    n645 = Less?(x=w2233, y=1) -> (x < y?=w2239:bool)
                    n646 = case shown="False" w2239 {
                      tunnel: w2233 -> [w2255 w2263]
                      tunnel: [w2257 FALSE] -> w2229
                      tunnel: [w2256 w2263] -> w2241
                      tunnel: w2235 -> [w2254 _]
                      tunnel: w2236 -> [w2252 _]
                      frame False {
                        # "Max Step"
                        # "# of steps\nminus 1"
                        n647 = Divide(x=300, y=w2252) -> (x/y=w2249:dbl)
                        n648 = To Unsigned Byte Integer(number=w2249) -> (unsigned 8bit integer=w2250:u8)
                        n649 = Greater Or Equal?(x=w2255, y=w2250) -> (x >= y?=w2251:bool)
                        n650 = case shown="True" w2251 {
                          tunnel: [w2258 TRUE] -> w2257
                          tunnel: [w2259 w2260] -> w2256
                          tunnel: w2255 -> [w2259 w2260]
                          tunnel: w2254 -> [w2258 _]
                          frame False {
                            # "No Need to\nChange Direction"
                          }
                          frame True {
                            # "T"
                            # "Move CW"
                          }
                        }
                      }
                      frame True {
                        # "F"
                        # "Move CCW"
                      }
                    }
                    n651 = case shown="True" w2229 {
                      tunnel: w2241 -> [w2246 w2247]
                      tunnel: [w2245 w2248] -> w2237
                      frame False {
                        # "CCW\n+1"
                        n652 = Increment(x=w2246) -> (x+1=w2245:i8)
                      }
                      frame True {
                        # "CW\n-1"
                        n653 = Decrement(x=w2247) -> (x-1=w2248:i8)
                      }
                    }
                    n654 = Multiply(x=w2237, y=w2236) -> (x*y=w2234:u16)
                    n655 = To Unsigned Word Integer(number=w2234) -> (unsigned 16bit integer=w2232:u16)
                    n656 = Add(x=200, y=w2232) -> (x+y=w2226:i32)
                  }
                }
                n657 = local read "Image Lock - Right"() -> (w2191:bool)
                n658 = case shown="True" w2190 {
                  tunnel: [w2209 w2219] -> w2197
                  tunnel: w2198 -> [w2210 _]
                  tunnel: [w2211 enum16{"Generic Sweep", "Recovery Search"}."Generic Sweep"] -> w2195
                  tunnel: [w2208 w2219] -> w2196
                  tunnel: w2191 -> [w2207 _]
                  frame False {
                    # "Is other servo tracking?"
                    n659 = case shown="True" w2207 {
                      tunnel: [enum16{"Generic Sweep", "Recovery Search"}."Generic Sweep" enum16{"Generic Sweep", "Recovery Search"}."Recovery Search"] -> w2211
                      tunnel: w2210 -> [w2214 _]
                      tunnel: [w2214 FALSE] -> w2209
                      tunnel: [FALSE TRUE] -> w2208
                      frame False {
                        # "Stay in Sweep"
                      }
                      frame True {
                        # "G o to Recovery Search  State"
                      }
                    }
                  }
                  frame True {
                    w2219 = FALSE
                    # "Override Move Servo\nCommand bc an Angle Was Found\nduring this Step"
                    # "Stay In Sweep\nLet Main State Machine transition\ninto Tracking"
                  }
                }
              }
            }
            n660 = Increment(x=w2085) -> (x+1=w2066:i32)
            n661 = case shown="False" w2077 {
              tunnel: w2066 -> [w2100 _]
              tunnel: [w2100 0] -> w2078
              frame False {
              }
              frame True {
              }
            }
            n662 = case shown="False" w2065 {
              tunnel: [T5."Recovery Mode" ("Next Main State") T5."Tracking" ("Next Main State")] -> w2076
              frame False {
              }
              frame True {
              }
            }
          }
        }
        "Current Move Delta - L" <- w1803
        n663 = Less?(x=w1830, y=w1829) -> (x < y?=w1828:bool)
        n664 = local write "New Data  Flag\nLeft Servo"(FALSE) -> ()
        n665 = Select(t=w1829, s=w1828, f=w1830) -> (s? t:f=w1825:i32)
        n666 = Greater?(x=w1825, y=w1826) -> (0:w1827:bool)
        n667 = Select(t=w1826, s=w1827, f=w1825) -> (s? t:f=w1824:i32)
      }
    }
    "Next Main State - Left" <- w1252
    "Next Tracking State - Left" <- w1235
    "Next Recovery State - Left" <- w1233
    n668 = case shown="True" w1216 {
      tunnel: [w1301 w1339] -> w1186
      tunnel: [w1295 w1338] -> w1185
      tunnel: w1221 -> [w1296 w1337]
      tunnel: w1218 -> [_ w1336]
      tunnel: "Track Angle Valid  - Right" -> [_ w1335]
      tunnel: w1215 -> [_ w1334]
      tunnel: w1214 -> [w1301 w1333]
      tunnel: "Mounting Offset - Right" -> [_ w1332]
      tunnel: w1209 -> [w1292 w1331]
      tunnel: w1207 -> [_ w1330]
      tunnel: w1204 -> [w1293 w1329]
      tunnel: w1202 -> [_ w1328]
      tunnel: w1201 -> [_ w1327]
      tunnel: w1200 -> [_ w1326]
      tunnel: w1199 -> [_ w1325]
      tunnel: w1197 -> [w1291 w1324]
      tunnel: w1206 -> [w1290 w1323]
      tunnel: w1205 -> [w1294 w1322]
      tunnel: w1211 -> [_ w1321]
      tunnel: w1210 -> [_ w1320]
      tunnel: w1208 -> [_ w1319]
      tunnel: [0 w1318] -> w1187
      tunnel: [w1296 w1317] -> w1184
      tunnel: [w1295 w1316] -> w1191
      tunnel: [w1294 w1315] -> w1192
      tunnel: [w1290 w1314] -> w1193
      tunnel: [w1293 w1313] -> w1194
      tunnel: [w1291 w1312] -> w1195
      tunnel: w1198 -> [_ w1311]
      tunnel: [w1292 w1310] -> w1196
      tunnel: w1203 -> [_ w1309]
      tunnel: w1213 -> [w1299 w1308]
      tunnel: w1219 -> [w1298 w1307]
      tunnel: [w1299 w1306] -> w1188
      tunnel: [w1298 w1305] -> w1190
      tunnel: w1220 -> [w1297 w1304]
      tunnel: [w1297 w1303] -> w1189
      frame False {
        w1295 = FALSE
        # "Recovery Mode COunt"
        # "Frames Processed - L"
        # "Recovery Search move Count - L"
        # "Recovery Search Attempt Count- L"
        # "WAITING FOR NEW IMAGE, RETAIN ALL VALUES"
      }
      frame True {
        w1341 = u16 1023
        w1344 = u16 0
        # "New Tracking State"
        # "Tracking Timeout Count"
        # "Next Main State"
        # "Next Recovery State"
        # "Reset Respond"
        # "Search Direction"
        # "Recovery Count"
        # "Recovery Search move Count"
        # "Recovery Search Attempt Count"
        # "Frames Processed"
        # "Apply Floor/Ceiling to Goal Position"
        # "Current move Delta"
        # "Service Track Angle Flag"
        # "Move Servo"
        # "Goal Position"
        # "Go to Current State"
        n669 = case shown="\"Recovery Mode\"" w1337 {
          tunnel: w1333 -> [w1362 w1434 w1602]
          tunnel: w1334 -> [_ w1436 _]
          tunnel: w1319 -> [w1361 _ w1597]
          tunnel: w1331 -> [w1360 w1417 w1591]
          tunnel: [w1359 w1432 w1601] -> w1345
          tunnel: [w1357 w1433 w1600] -> w1338
          tunnel: w1335 -> [_ w1427 w1578]
          tunnel: [w1355 w1429 w1587] -> w1317
          tunnel: w1336 -> [w1346 w1428 w1576]
          tunnel: w1332 -> [_ w1437 w1598]
          tunnel: w1321 -> [_ w1435 _]
          tunnel: [w1349 w1431 w1582] -> w1318
          tunnel: w1320 -> [_ w1430 _]
          tunnel: w1329 -> [w1354 _ w1592]
          tunnel: [enum16{"Generic Sweep", "Recovery Search"}."Recovery Search" enum16{"Generic Sweep", "Recovery Search"}."Recovery Search" w1599] -> w1303
          tunnel: w1324 -> [_ _ w1596]
          tunnel: w1304 -> [_ _ w1579]
          tunnel: w1330 -> [_ w1414 w1608]
          tunnel: w1311 -> [_ w1410 w1603]
          tunnel: w1326 -> [_ w1420 w1605]
          tunnel: w1327 -> [_ w1421 w1606]
          tunnel: w1328 -> [_ w1422 w1607]
          tunnel: w1325 -> [_ w1419 w1604]
          tunnel: [FALSE w1416 w1580] -> w1316
          tunnel: w1309 -> [w1353 _ w1590]
          tunnel: [w1349 w1411 w1589] -> w1312
          tunnel: [w1349 w1411 w1595] -> w1315
          tunnel: [w1349 w1411 w1594] -> w1314
          tunnel: [w1352 w1412 w1593] -> w1313
          tunnel: w1323 -> [_ _ w1585]
          tunnel: w1322 -> [_ _ w1584]
          tunnel: [w1350 w1417 w1583] -> w1310
          tunnel: w1308 -> [_ w1426 _]
          tunnel: [w1349 w1418 w1582] -> w1306
          tunnel: w1307 -> [_ w1423 _]
          tunnel: [enum16{"Track", "Reactive Predict", ""}."Track" ("Initial Tracking State - Right") w1415 enum16{"Track", "Reactive Predict", ""}."Track" ("Initial Tracking State - Right")] -> w1305
          frame "Start Up Search", Default {
            w1349 = u16 0
            # "Image Lock"
            # "Search Direction"
            # "Wait for 'x' Images to be Processed\nBefore Going to Next Step"
            # "Next Main State"
            # "New Goal Position"
            # "Move Servo"
            # "Choose Next State"
            # "Frames Processed Count"
            n670 = Greater Or Equal?(x=w1354, y=w1353) -> (x >= y?=w1358:bool)
            n671 = case shown="True" w1358 {
              tunnel: w1362 -> [w1372 w1384]
              tunnel: w1361 -> [_ w1382]
              tunnel: w1360 -> [w1371 w1381]
              tunnel: [w1372 w1378] -> w1359
              tunnel: [w1370 0] -> w1352
              tunnel: [FALSE TRUE] -> w1356
              tunnel: w1354 -> [w1373 _]
              tunnel: [w1371 w1375] -> w1350
              frame False {
                # "Wait until Min Number of Frames (per search/step) Processed"
                # "Increase Frames\nProcessed Count"
                n672 = Increment(x=w1373) -> (x+1=w1370:i32)
              }
              frame True {
                # "Reset Frames\nProcessed Count"
                # "SWEEP SEARCH - Startup"
                # "Multiple New Step\nby Step SIze"
                # "F = CCW\nT = CW"
                # "Last Direction"
                # "Min Step"
                # "add in case\nactual position\nis lower than GP"
                # "Set New Step #"
                # "Choose Direction"
                # "Nearest step"
                # "Adjust Actual Posiiton\n to pre-determiend steps"
                # "Move Servo 1 \"Step\" to\nSearch"
                n673 = Add(x=3, y=w1384) -> (x+y=w1390:i32)
                n674 = Quotient & Remainder(x=w1390, y=w1382) -> (floor(x/y)=w1388:i32)  [unwired: 1 out]
                n675 = To Byte Integer(number=w1388) -> (8bit integer=w1379:i8)
                n676 = Less?(x=w1379, y=1) -> (x < y?=w1385:bool)
                n677 = case shown="False" w1385 {
                  tunnel: w1379 -> [w1401 w1409]
                  tunnel: [w1403 FALSE] -> w1375
                  tunnel: [w1402 w1409] -> w1387
                  tunnel: w1381 -> [w1400 _]
                  tunnel: w1382 -> [w1398 _]
                  frame False {
                    # "Max Step"
                    # "# of steps\nminus 1"
                    n678 = Divide(x=1024, y=w1398) -> (x/y=w1395:dbl)
                    n679 = To Unsigned Byte Integer(number=w1395) -> (unsigned 8bit integer=w1396:u8)
                    n680 = Greater Or Equal?(x=w1401, y=w1396) -> (x >= y?=w1397:bool)
                    n681 = case shown="True" w1397 {
                      tunnel: [w1404 TRUE] -> w1403
                      tunnel: [w1405 w1406] -> w1402
                      tunnel: w1401 -> [w1405 w1406]
                      tunnel: w1400 -> [w1404 _]
                      frame False {
                        # "No Need to\nChange Direction"
                      }
                      frame True {
                        # "T"
                        # "Move CW"
                      }
                    }
                  }
                  frame True {
                    # "F"
                    # "Move CCW"
                  }
                }
                n682 = case shown="False" w1375 {
                  tunnel: w1387 -> [w1392 w1393]
                  tunnel: [w1391 w1394] -> w1383
                  frame False {
                    # "CCW\n+1"
                    n683 = Increment(x=w1392) -> (x+1=w1391:i8)
                  }
                  frame True {
                    # "CW\n-1"
                    n684 = Decrement(x=w1393) -> (x-1=w1394:i8)
                  }
                }
                n685 = Multiply(x=w1383, y=w1382) -> (x*y=w1380:u16)
                n686 = To Unsigned Word Integer(number=w1380) -> (unsigned 16bit integer=w1378:u16)
              }
            }
            n687 = case shown="False" w1346 {
              tunnel: [w1364 FALSE] -> w1357
              tunnel: w1356 -> [w1364 _]
              tunnel: [w1365 T5."Tracking" ("Next Main State")] -> w1355
              frame False {
                # "Check other Servo\nStay in Startup  State"
                n688 = local read "Image Lock - Left"() -> (w1363:bool)
                n689 = case shown="False" w1363 {
                  tunnel: [T5."Start Up Search" ("Next Main State") T5."Recovery Mode" ("Next Main State")] -> w1365
                  frame False {
                  }
                  frame True {
                  }
                }
              }
              frame True {
                # "Override Move Servo\nCommand bc an Angle Was Found\nduring this Step"
                # "Transition to Tracking State When\nImage Processing has Locked"
              }
            }
          }
          frame "Tracking" {
            w1411 = 0
            # "Frames Processed Count"
            # "Image Lock - L"
            # "Track Angle Valid"
            # "Tracking Angle"
            # "Tracking Timeout Count"
            # "Max ove delta"
            # "Move delta threshold"
            # "mount offset"
            # "Current Position"
            # "Move Respond"
            # "Trackin Timeout count"
            # "Move Servo"
            # "delta"
            # "GP"
            # "Reset Move Respond"
            # "New Tracking State"
            # "Delta Move Sum"
            # "Choose Next State"
            n690 = case shown="\"Track\", Default" w1423 {
              tunnel: w1437 -> [w1455 _]
              tunnel: w1436 -> [w1454 _]
              tunnel: w1435 -> [w1453 _]
              tunnel: w1434 -> [w1452 w1500]
              tunnel: [w1451 w1498] -> w1433
              tunnel: [w1450 w1506] -> w1432
              tunnel: [w1449 0] -> w1431
              tunnel: w1430 -> [w1448 _]
              tunnel: w1428 -> [w1447 w1490]
              tunnel: w1427 -> [w1446 w1493]
              tunnel: w1426 -> [w1445 w1495]
              tunnel: w1422 -> [_ w1505]
              tunnel: w1421 -> [_ w1504]
              tunnel: w1420 -> [_ w1503]
              tunnel: w1419 -> [_ w1502]
              tunnel: w1414 -> [_ w1501]
              tunnel: w1410 -> [_ w1499]
              tunnel: [TRUE w1496] -> w1416
              tunnel: [w1442 w1494] -> w1418
              tunnel: [w1440 w1492] -> w1415
              tunnel: [0 0] -> w1412
              frame "Track", Default {
                # "Reset"
                # "Tracking Timeout"
                # "Move Delta"
                # "Goal Position"
                # "Tracking Move"
                # "Move Servo"
                # "Only Consider Tracking Angle\n\nIF\n\nImage Locked        == T\nTrack Angle Flag   == T"
                n691 = And(x=w1447, y=w1446) -> (x .and. y?=w1439:bool)
                n692 = case shown="True" w1439 {
                  tunnel: w1455 -> [_ w1463]
                  tunnel: w1454 -> [_ w1461]
                  tunnel: w1453 -> [_ w1478]
                  tunnel: w1452 -> [w1458 w1468]
                  tunnel: [w1458 w1477] -> w1450
                  tunnel: [w1460 w1476] -> w1451
                  tunnel: [w1460 w1475] -> _
                  tunnel: [u16 0 w1474] -> w1449
                  tunnel: w1448 -> [_ w1470]
                  tunnel: w1445 -> [w1457 _]
                  tunnel: [w1456 0] -> w1442
                  frame False {
                    w1460 = FALSE
                    # "Increment timeout"
                    n693 = Increment(x=w1457) -> (x+1=w1456:i32)
                  }
                  frame True {
                    # "******"
                    # "Move to Tracking Angle \n\nif delta is greater than move servo threshold\nAND less than max move threshold"
                    n694 = call "Servo_GP_Angle_Conversion_R0.vi"("Angle In"=w1461, "Mode Select"=1, "Mount Offset"=w1463) -> ("GP out"=w1462:u16)  [unwired: 7 in, 1 out]
                    n695 = To Word Integer(number=w1468) -> (16bit integer=w1466:i16)
                    n696 = To Word Integer(number=w1462) -> (16bit integer=w1479:i16)
                    n697 = Subtract(x=w1479, y=w1466) -> (x-y=w1469:i16)
                    n698 = Absolute Value(x=w1469) -> (abs(x)=w1465:i16)
                    n699 = Greater Or Equal?(x=w1465, y=w1478) -> (x >= y?=w1472:bool)
                    n700 = Less Or Equal?(x=w1465, y=w1470) -> (x <= y?=w1471:bool)
                    n701 = And(x=w1472, y=w1471) -> (x .and. y?=w1473:bool)
                    n702 = case shown="True" w1473 {
                      tunnel: w1462 -> [_ w1484]
                      tunnel: [w1481 w1484] -> w1477
                      tunnel: [w1482 w1486] -> w1476
                      tunnel: [w1482 w1486] -> w1475
                      tunnel: w1468 -> [w1481 _]
                      tunnel: w1465 -> [_ w1485]
                      tunnel: [u16 0 w1485] -> w1474
                      tunnel: w1461 -> [_ w1483]
                      frame False {
                        w1482 = FALSE
                        # "Don't Move"
                      }
                      frame True {
                        w1486 = TRUE
                        # "Current Delta"
                        # "Use new Track Angle"
                        n703 = local write "Last Track Angle - R"(w1483) -> ()
                      }
                    }
                  }
                }
                n704 = local read "Timeout to \nEnable Reactive Predict"() -> (w1443:u16)
                n705 = Less?(x=w1442, y=w1443) -> (x < y?=w1441:bool)
                n706 = case shown="True" w1441 {
                  tunnel: [enum16{"Track", "Reactive Predict", ""}."Reactive Predict" ("Initial Tracking State - Right") enum16{"Track", "Reactive Predict", ""}."Track" ("Initial Tracking State - Right")] -> w1440
                  frame False {
                  }
                  frame True {
                  }
                }
              }
              frame "Reactive Predict" {
                # "Choose New\nTracking State"
                n707 = Or(x=w1490, y=w1493) -> (x .or. y?=w1489:bool)
                n708 = case shown="False" w1489 {
                  tunnel: [w1519 w1572] -> w1506
                  tunnel: w1505 -> [w1518 _]
                  tunnel: w1504 -> [w1517 _]
                  tunnel: w1503 -> [w1516 _]
                  tunnel: w1502 -> [w1515 _]
                  tunnel: w1501 -> [w1514 _]
                  tunnel: w1499 -> [w1513 _]
                  tunnel: [w1512 FALSE] -> w1498
                  tunnel: [w1511 TRUE] -> w1496
                  tunnel: w1495 -> [w1510 _]
                  tunnel: [w1509 0] -> w1494
                  tunnel: [enum16{"Track", "Reactive Predict", ""}."Reactive Predict" ("Initial Tracking State - Right") enum16{"Track", "Reactive Predict", ""}."Track" ("Initial Tracking State - Right")] -> w1492
                  tunnel: w1500 -> [w1507 w1572]
                  frame False {
                    # "Stay in Reactive State"
                    # "Increment Track Timeout"
                    # "Move Respond Flag"
                    n709 = Increment(x=w1510) -> (x+1=w1509:i32)
                    n710 = case shown="True" w1514 {
                      tunnel: w1518 -> [_ w1534]
                      tunnel: w1517 -> [_ w1533]
                      tunnel: w1516 -> [_ w1532]
                      tunnel: w1515 -> [_ w1531]
                      tunnel: w1513 -> [_ w1528]
                      tunnel: [w1520 w1524] -> w1519
                      tunnel: [w1521 w1523] -> w1512
                      tunnel: [w1521 w1523] -> w1511
                      tunnel: w1507 -> [w1520 w1522]
                      frame False {
                        w1521 = FALSE
                        # "Reset Move Respond = F"
                        # "Move Servo = F"
                      }
                      frame True {
                        w1523 = TRUE
                        # "Position Lock"
                        # "Current Servo\nPosition"
                        # "Reset Move\nRespond = T"
                        # "Move Servo = T"
                        # "Apply Direction \nto Offset (delta sum)"
                        # "Check Last Known Position of Robot"
                        n711 = case shown="True" w1534 {
                          tunnel: w1533 -> [_ w1562]
                          tunnel: w1532 -> [_ w1537]
                          tunnel: w1531 -> [_ w1538]
                          tunnel: [sgl 1.0 ("y") w1536] -> w1530
                          frame False {
                            # "No Position Data Available"
                            # "Default is to move\nSame Direction as other\nServo"
                          }
                          frame True {
                            w1543 = sgl 1.0 ("y")
                            # "Use previous position/orientation to Guess Which Direction to Move Servo"
                            # "Choose Search Direction"
                            # "\"Perpendicular \nThreshold\""
                            # "If Orientation is\n ~Perpendicular -> Start Search\n in Opposite Direction of Other"
                            # "****add 90 until orientation angle is fixed"
                            # "Last Orientation"
                            # "Convert to Rad"
                            # "Avoid Divide by 0"
                            # "-1/m"
                            # "Calculate Normal Line to \nLast Robot Position\nfrom Center Beacon"
                            # "last Position \nCoordinates"
                            n712 = Unbundle(w1562) -> ("X"=w1542:sgl, "Y"=w1541:sgl)
                            n713 = Unbundle(w1538) -> ("X"=w1540:sgl, "Y"=w1539:sgl)
                            n714 = Subtract(x=w1541, y=w1539) -> (x-y=w1558:sgl)
                            n715 = Subtract(x=w1542, y=w1540) -> (x-y=w1556:sgl)
                            n716 = Equal To 0?(x=w1556) -> (x = 0?=w1557:bool)
                            n717 = case shown="False" w1557 {
                              tunnel: w1558 -> [w1565 _]
                              tunnel: w1556 -> [w1564 _]
                              tunnel: [w1563 1000000000000000.0] -> w1555
                              frame False {
                                n718 = Divide(x=w1565, y=w1564) -> (x/y=w1563:sgl)
                              }
                              frame True {
                              }
                            }
                            n719 = Equal To 0?(x=w1555) -> (x = 0?=w1560:bool)
                            n720 = case shown="False" w1560 {
                              tunnel: [w1567 1e-08] -> w1559
                              tunnel: w1555 -> [w1567 _]
                              frame False {
                              }
                              frame True {
                                # "Can't have infinit slope"
                              }
                            }
                            n721 = Divide(x=-1.0, y=w1559) -> (x/y=w1554:dbl)
                            n722 = Inverse Tangent(1:w1554) -> (0:w1552:dbl)
                            n723 = expression code="(x/pi)*180.0" "radians to degrees"(w1552) -> (w1553:dbl)
                            n724 = To Single Precision Float(number=w1553) -> (single precision float=w1550:sgl)
                            n725 = Add(x=w1537, y=sgl 90.0) -> (x+y=w1549:sgl)
                            n726 = Subtract(x=w1550, y=w1549) -> (x-y=w1548:sgl)
                            n727 = Absolute Value(x=w1548) -> (abs(x)=w1547:sgl)
                            n728 = Less Or Equal?(x=w1547, y=sgl 10.0) -> (x <= y?=w1545:bool)
                            n729 = Negate(x=w1543) -> (-x=w1544:sgl)
                            n730 = Select(t=w1544, s=w1545, f=w1543) -> (s? t:f=w1536:sgl)
                          }
                        }
                        n731 = To Word Integer(number=w1530) -> (16bit integer=w1529:i16)
                        n732 = Multiply(x=w1529, y=w1528) -> (x*y=w1527:i32)
                        n733 = To Word Integer(number=w1522) -> (16bit integer=w1526:i16)
                        n734 = Add(x=w1527, y=w1526) -> (x+y=w1525:i32)
                        n735 = To Unsigned Word Integer(number=w1525) -> (unsigned 16bit integer=w1524:u16)
                      }
                    }
                  }
                  frame True {
                    # "Either Current Angle Valid or Image Lock Acheived"
                    # "Go Directly to Track State"
                  }
                }
              }
            }
            n736 = local read "Tracking Timeout\nThreshold"() -> (w1424:i32)
            n737 = Less?(x=w1418, y=w1424) -> (x < y?=w1425:bool)
            n738 = case shown="True" w1425 {
              tunnel: [T5."Recovery Mode" ("Next Main State") T5."Tracking" ("Next Main State")] -> w1429
              frame False {
              }
              frame True {
              }
            }
          }
          frame "Recovery Mode" {
            w1582 = u16 0
            # "Recovery Search Move Count"
            # "***Compltetly resets as of R17, used to just reset to \"Max Recovery Count - 1\""
            # "Increment Recoveyr Mode Count"
            # "Frames Processed"
            # "Choose Next Main State"
            # "Reset recovery count"
            # "Recovery move\nCount"
            # "Recovery Search\nAttempt count"
            # "Move Servo = T"
            # "delta move sum"
            # "Robot Position Valid"
            n739 = local read "Image Lock - Left"() -> (w1586:bool)
            n740 = case shown="\"Recovery Search\"" w1579 {
              tunnel: w1608 -> [_ _]
              tunnel: w1607 -> [_ _]
              tunnel: w1606 -> [_ _]
              tunnel: w1605 -> [_ _]
              tunnel: w1604 -> [_ _]
              tunnel: w1603 -> [_ _]
              tunnel: w1602 -> [w1636 w1716]
              tunnel: [w1628 w1714] -> w1601
              tunnel: [w1625 w1708] -> w1600
              tunnel: [FALSE FALSE] -> w1580
              tunnel: [w1630 w1706] -> w1599
              tunnel: w1596 -> [w1634 _]
              tunnel: w1598 -> [w1637 _]
              tunnel: w1597 -> [w1635 w1711]
              tunnel: [w1627 w1705] -> w1594
              tunnel: [w1626 w1705] -> w1595
              tunnel: w1586 -> [w1624 _]
              tunnel: [w1615 w1715] -> w1593
              tunnel: w1592 -> [w1613 w1703]
              tunnel: w1591 -> [w1618 w1712]
              tunnel: w1590 -> [w1614 w1710]
              tunnel: w1576 -> [_ _]
              tunnel: w1578 -> [_ _]
              tunnel: [FALSE w1707] -> w1588
              tunnel: w1585 -> [w1622 _]
              tunnel: w1584 -> [w1621 _]
              tunnel: [w1618 w1704] -> w1583
              tunnel: w1576 -> [_ w1701]
              frame "Recovery Search" {
                # "Wait for 2 Images to be Processed\nBefore Going to Next Step"
                # "Choose Next Reovery State"
                # "Recovery Search \nAttempt Count"
                # "Move Servo"
                # "Goal Position"
                # "Recovery Search\nmove Count"
                # "Attempt Recovery Search if Other Servo has Valid Angle"
                n741 = local read "Last Track Angle - L"() -> (w1617:sgl)
                n742 = Greater Or Equal?(x=w1613, y=w1614) -> (x >= y?=w1616:bool)
                n743 = case shown="True" w1616 {
                  tunnel: w1637 -> [_ w1657]
                  tunnel: [w1642 w1656] -> w1626
                  tunnel: w1636 -> [w1645 w1655]
                  tunnel: w1635 -> [_ w1654]
                  tunnel: [w1643 w1653] -> w1627
                  tunnel: [w1645 w1652] -> w1628
                  tunnel: [FALSE w1651] -> w1625
                  tunnel: w1622 -> [w1643 w1650]
                  tunnel: w1621 -> [w1642 w1649]
                  tunnel: w1624 -> [_ w1648]
                  tunnel: w1617 -> [_ w1647]
                  tunnel: [w1640 0 ("Frames Processed\nCount - in")] -> w1615
                  tunnel: w1613 -> [w1641 _]
                  frame False {
                    # "Increment Frames Processed"
                    # "WAIT"
                    n744 = Increment(x=w1641) -> (x+1=w1640:i32)
                  }
                  frame True {
                    n745 = case shown="True" w1648 {
                      tunnel: w1647 -> [_ w1670]
                      tunnel: w1650 -> [w1658 w1666]
                      tunnel: w1657 -> [_ w1671]
                      tunnel: [w1661 w1669] -> w1652
                      tunnel: [w1659 w1668] -> w1656
                      tunnel: w1649 -> [w1659 w1667]
                      tunnel: w1655 -> [w1661 w1665]
                      tunnel: w1654 -> [_ w1664]
                      tunnel: [FALSE TRUE] -> w1651
                      tunnel: [w1658 w1662] -> w1653
                      frame False {
                        # "Don't Move bc Other Servo Doesn't Have Image Lock"
                      }
                      frame True {
                        # "Move Servo = T"
                        n746 = Greater Than 0?(x=w1666) -> (x > 0?=w1672:bool)
                        n747 = case shown="False" w1672 {
                          tunnel: w1671 -> [w1674 _]
                          tunnel: w1670 -> [w1675 _]
                          tunnel: [w1678 w1686] -> w1669
                          tunnel: [w1681 w1691] -> w1668
                          tunnel: w1667 -> [w1682 w1691]
                          tunnel: w1666 -> [w1680 w1688]
                          tunnel: [w1679 w1690] -> w1662
                          tunnel: w1665 -> [_ w1687]
                          tunnel: w1664 -> [_ w1684]
                          frame False {
                            # "************************"
                            # "Increment move count to transition\nto Pan mode"
                            # "Increment Recovery Search Attempt Count"
                            # "Move Parallel to Other Servo"
                            n748 = Increment(x=w1682) -> (x+1=w1681:i32)
                            n749 = call "Servo_GP_Angle_Conversion_R0.vi"("Angle In"=w1675, "Mode Select"=1, "Mount Offset"=w1674) -> ("GP out"=w1673:u16)  [unwired: 7 in, 1 out]
                            n750 = Increment(x=w1680) -> (x+1=w1679:i32)
                            n751 = local read "Recovery Parallel\nSearch Offset"() -> (w1677:u16)
                            n752 = Subtract(x=w1673, y=w1677) -> (x-y=w1678:u16)
                          }
                          frame True {
                            # "Apply Direction"
                            # "Step SIze"
                            # "Current Position"
                            # "Attempt to Pan in Steps Towards other Servo"
                            # "Could be same or function of \nregular search step size"
                            # "Max # of Pan\nMoves"
                            # "Pan Towards Other Servo"
                            n753 = local read "Max # Pan Moves"() -> (w1683:u16)
                            n754 = Greater Or Equal?(x=w1688, y=w1683) -> (x >= y?=w1689:bool)
                            n755 = case shown="False" w1689 {
                              tunnel: w1688 -> [w1699 _]
                              tunnel: [w1698 u16 0] -> w1690
                              frame False {
                                # "Increment Pan Count"
                                n756 = Increment(x=w1699) -> (x+1=w1698:i32)
                              }
                              frame True {
                                # "Reset move count"
                              }
                            }
                            n757 = local read "Recovery Search\nDirection - R"() -> (w1685:bool)
                            n758 = case shown="True" w1685 {
                              tunnel: w1687 -> [w1693 w1697]
                              tunnel: w1684 -> [w1694 w1696]
                              tunnel: [w1692 w1695] -> w1686
                              frame False {
                                # "CCW"
                                n759 = Add(x=w1693, y=w1694) -> (x+y=w1692:u16)
                              }
                              frame True {
                                # "CW"
                                n760 = Subtract(x=w1697, y=w1696) -> (x-y=w1695:u16)
                              }
                            }
                          }
                        }
                      }
                    }
                  }
                }
                n761 = local read "Max Recovery Count\n(Recovery Search)"() -> (w1619:u16)
                n762 = local read "Max Recovery\nSearch Attempts"() -> (w1620:u16)
                n763 = Less Or Equal?(x=w1626, y=w1620) -> (x <= y?=w1632:bool)
                n764 = Less Or Equal?(x=w1634, y=w1619) -> (x <= y?=w1633:bool)
                n765 = And(x=w1632, y=w1633) -> (x .and. y?=w1631:bool)
                n766 = case shown="True" w1631 {
                  tunnel: [enum16{"Generic Sweep", "Recovery Search"}."Generic Sweep" enum16{"Generic Sweep", "Recovery Search"}."Recovery Search"] -> w1630
                  frame False {
                  }
                  frame True {
                  }
                }
              }
              frame "Generic Sweep" {
                w1705 = u16 0
                # "Image Locked?"
                # "Choose Next Recovery State"
                # "Wait for 2 Images to be Processed\nBefore Going to Next Step"
                # "New Goal Position"
                # "Move Servo"
                # "Frames Processed Count"
                n767 = Greater Or Equal?(x=w1703, y=w1710) -> (x >= y?=w1717:bool)
                n768 = case shown="True" w1717 {
                  tunnel: w1716 -> [w1733 w1749]
                  tunnel: w1711 -> [_ w1747]
                  tunnel: w1712 -> [w1732 w1746]
                  tunnel: [w1733 w1739] -> w1714
                  tunnel: [w1731 0] -> w1715
                  tunnel: [FALSE TRUE] -> w1709
                  tunnel: w1703 -> [w1734 _]
                  tunnel: [w1732 w1740] -> w1704
                  frame False {
                    # "Increment Frames Processed"
                    n769 = Increment(x=w1734) -> (x+1=w1731:i32)
                  }
                  frame True {
                    # "Reset Frames\nProcessed Count"
                    # "SWEEP SEARCH - Startup"
                    # "Multiple New Step\nby Step SIze"
                    # "F = CCW\nT = CW"
                    # "Last Direction"
                    # "Min Step"
                    # "add 10 in case\nactual position\nis lower than GP"
                    # "Set New Step #"
                    # "Choose Direction"
                    # "Nearest step"
                    # "Adjust Actual Posiiton\n to pre-determiend steps"
                    # "Move Servo 1 \"Step\" to\nSearch"
                    n770 = Subtract(x=w1749, y=u16 524) -> (x-y=w1737:u16)
                    n771 = Add(x=5, y=w1737) -> (x+y=w1755:i32)
                    n772 = Quotient & Remainder(x=w1755, y=w1747) -> (floor(x/y)=w1753:i32)  [unwired: 1 out]
                    n773 = To Byte Integer(number=w1753) -> (8bit integer=w1744:i8)
                    n774 = Less?(x=w1744, y=1) -> (x < y?=w1750:bool)
                    n775 = case shown="False" w1750 {
                      tunnel: w1744 -> [w1766 w1774]
                      tunnel: [w1768 FALSE] -> w1740
                      tunnel: [w1767 w1774] -> w1752
                      tunnel: w1746 -> [w1765 _]
                      tunnel: w1747 -> [w1763 _]
                      frame False {
                        # "Max Step"
                        # "# of steps\nminus 1"
                        n776 = Divide(x=300, y=w1763) -> (x/y=w1760:dbl)
                        n777 = To Unsigned Byte Integer(number=w1760) -> (unsigned 8bit integer=w1761:u8)
                        n778 = Greater Or Equal?(x=w1766, y=w1761) -> (x >= y?=w1762:bool)
                        n779 = case shown="True" w1762 {
                          tunnel: [w1769 TRUE] -> w1768
                          tunnel: [w1770 w1771] -> w1767
                          tunnel: w1766 -> [w1770 w1771]
                          tunnel: w1765 -> [w1769 _]
                          frame False {
                            # "No Need to\nChange Direction"
                          }
                          frame True {
                            # "T"
                            # "Move CW"
                          }
                        }
                      }
                      frame True {
                        # "F"
                        # "Move CCW"
                      }
                    }
                    n780 = case shown="True" w1740 {
                      tunnel: w1752 -> [w1757 w1758]
                      tunnel: [w1756 w1759] -> w1748
                      frame False {
                        # "CCW\n+1"
                        n781 = Increment(x=w1757) -> (x+1=w1756:i8)
                      }
                      frame True {
                        # "CW\n-1"
                        n782 = Decrement(x=w1758) -> (x-1=w1759:i8)
                      }
                    }
                    n783 = Multiply(x=w1748, y=w1747) -> (x*y=w1745:u16)
                    n784 = To Unsigned Word Integer(number=w1745) -> (unsigned 16bit integer=w1743:u16)
                    n785 = Add(x=w1743, y=u16 524) -> (x+y=w1739:u16)
                  }
                }
                n786 = local read "Image Lock - Left"() -> (w1702:bool)
                n787 = case shown="False" w1701 {
                  tunnel: [w1720 w1730] -> w1708
                  tunnel: w1709 -> [w1721 _]
                  tunnel: [w1722 enum16{"Generic Sweep", "Recovery Search"}."Generic Sweep"] -> w1706
                  tunnel: [w1719 w1730] -> w1707
                  tunnel: w1702 -> [w1718 _]
                  frame False {
                    # "Is other servo tracking?"
                    n788 = case shown="True" w1718 {
                      tunnel: [enum16{"Generic Sweep", "Recovery Search"}."Generic Sweep" enum16{"Generic Sweep", "Recovery Search"}."Recovery Search"] -> w1722
                      tunnel: w1721 -> [w1725 _]
                      tunnel: [w1725 FALSE] -> w1720
                      tunnel: [FALSE TRUE] -> w1719
                      frame False {
                        # "Stay in Sweep"
                      }
                      frame True {
                        # "G o to Recovery Search  State"
                      }
                    }
                  }
                  frame True {
                    w1730 = FALSE
                    # "Override Move Servo\nCommand bc an Angle Was Found\nduring this Step"
                    # "Stay In Sweep\nLet Main State Machine transition\ninto Tracking"
                  }
                }
              }
            }
            n789 = Increment(x=w1596) -> (x+1=w1577:i32)
            n790 = case shown="False" w1588 {
              tunnel: w1577 -> [w1611 _]
              tunnel: [w1611 0] -> w1589
              frame False {
              }
              frame True {
              }
            }
            n791 = case shown="False" w1576 {
              tunnel: [T5."Recovery Mode" ("Next Main State") T5."Tracking" ("Next Main State")] -> w1587
              frame False {
              }
              frame True {
              }
            }
          }
        }
        "Current Move Delta - R" <- w1318
        n792 = local write "New Data  Flag\nRight Servo"(FALSE) -> ()
        n793 = Less?(x=w1345, y=w1344) -> (x < y?=w1343:bool)
        n794 = Select(t=w1344, s=w1343, f=w1345) -> (s? t:f=w1340:u16)
        n795 = Greater?(x=w1340, y=w1341) -> (0:w1342:bool)
        n796 = Select(t=w1341, s=w1342, f=w1340) -> (s? t:f=w1339:u16)
      }
    }
    "Next Main State - Right" <- w1184
    "Next Tracking State - Right" <- w1190
    "Next Recovery State - Right" <- w1189
    n797 = flat-sequence {
      tunnel: w1275 -> [w2270]
      tunnel: w1185 -> [w2269]
      tunnel: w1276 -> [w2272]
      tunnel: w1186 -> [w2271]
      tunnel: [w2270] -> w1289
      tunnel: [w2269] -> w1288
      tunnel: w1289 -> [w2278]
      tunnel: [w2277] -> w1284
      tunnel: [w2276] -> w1285
      tunnel: w1288 -> [w2275]
      frame #0 {
        # "Only Update GP if Moving Servo"
        n798 = case shown="True" w2270 {
          tunnel: w2272 -> [_ w2274]
          frame False {
          }
          frame True {
            # "Update Goal Position"
            n799 = local write "Servo Goal Position\n - Left"(w2274) -> ()
          }
        }
        n800 = case shown="True" w2269 {
          tunnel: w2271 -> [_ w2273]
          frame False {
          }
          frame True {
            # "New Direction"
            # "Update Goal Position"
            # "Update Direction"
            n801 = local write "Servo Goal Position\n - Right"(w2273) -> ()
          }
        }
      }
      frame #1 {
        # "Allow Comm Process to Take Down the Flag\nOnly Raise if not already in motion"
        n802 = local read "Servo Moving - R"() -> (w2283:bool)
        n803 = local read "Servo Moving - L"() -> (w2280:bool)
        n804 = local read "Move Servo - L"() -> (w2279:bool)
        n805 = local read "Move Servo - R"() -> (w2286:bool)
        n806 = Not(x=w2283) -> (.not. x?=w2285:bool)
        n807 = Not(x=w2280) -> (.not. x?=w2282:bool)
        n808 = And(x=w2275, y=w2285) -> (x .and. y?=w2284:bool)
        n809 = And(x=w2278, y=w2282) -> (x .and. y?=w2281:bool)
        n810 = case shown="True" w2284 {
          selector: w2284 -> [_ w2288]
          tunnel: [w2287 w2288] -> w2276
          tunnel: w2286 -> [w2287 _]
          frame False {
          }
          frame True {
          }
        }
        n811 = case shown="False" w2281 {
          selector: w2281 -> [_ w2290]
          tunnel: [w2289 w2290] -> w2277
          tunnel: w2279 -> [w2289 _]
          frame False {
          }
          frame True {
          }
        }
        n812 = local write "Move Servo - R"(w2276) -> ()
        n813 = local write "Move Servo - L"(w2277) -> ()
      }
    }
    n814 = local read "Current Tracking State - Right 2"() -> (w1229:enum16{"Track", "Reactive Predict", ""})
    n815 = local read "Current Tracking State - Left"() -> (w1231:enum16{"Track", "Reactive Predict", ""})
    n816 = local read "Current Main State - Left"() -> (w1255:T5)
    n817 = local read "Current Main State - Right"() -> (w1230:T5)
    n818 = Equal?(x=w1230, y=w1254) -> (x = y?=w1224:bool)
    n819 = Equal?(x=w1229, y=w1228) -> (x = y?=w1223:bool)
    n820 = Equal?(x=w1255, y=w1254) -> (x = y?=w1226:bool)
    n821 = Equal?(x=w1231, y=w1228) -> (x = y?=w1227:bool)
    n822 = And(x=w1224, y=w1223) -> (x .and. y?=w1222:bool)
    n823 = And(x=w1226, y=w1227) -> (x .and. y?=w1225:bool)
    n824 = And(x=w1225, y=w1284) -> (x .and. y?=w1280:bool)
    n825 = And(x=w1285, y=w1222) -> (x .and. y?=w1281:bool)
    n826 = And(x=w1225, y=w1222) -> (x .and. y?=w1279:bool)
    n827 = Exclusive Or(1:w1281, 2:w1280) -> (0:w1278:bool)
    n828 = case shown="True" w1278 {
      tunnel: [w2301 w2322] -> w1286
      tunnel: [w2302 w2321] -> w1282
      tunnel: w1187 -> [_ w2325]
      tunnel: w1245 -> [w2299 w2326]
      tunnel: w1198 -> [w2297 w2324]
      tunnel: [w2300 w2312] -> w1283
      tunnel: [w2298 w2311] -> w1287
      tunnel: w1253 -> [_ w2323]
      tunnel: w1279 -> [w2296 _]
      tunnel: w1280 -> [_ w2322]
      tunnel: w1281 -> [_ w2321]
      frame False {
        n829 = case shown="False" w2296 {
          tunnel: [w2306 w2308] -> w2302
          tunnel: [w2305 w2308] -> w2301
          tunnel: [w2304 w2307] -> w2300
          tunnel: w2299 -> [w2304 _]
          tunnel: [w2303 w2307] -> w2298
          tunnel: w2297 -> [w2303 _]
          frame False {
            # "No Movement\nRetain All Values"
            n830 = local read "Move Respond - L"() -> (w2306:bool)
            n831 = local read "Move Respond - R"() -> (w2305:bool)
          }
          frame True {
            w2307 = i16 0
            w2308 = FALSE
            # "Reset Delta Move sum\nfor both"
            # "F"
            # "Both Moved,\nMake Flags False"
          }
        }
      }
      frame True {
        w2318 = 200 ("y")
        w2309 = -200 ("y")
        # "Add/Clear Sum for \nServo That didn't move"
        # "Update Moving Servo's  Delta Position"
        # "if one Servo Moves, other should \nmove too eventually,\nUsed in Search Process"
        # "Only 1 Servo is Moving Due to Tracking --> Update delta move sum"
        n832 = case shown="True" w2321 {
          tunnel: w2326 -> [_ w2334]
          tunnel: w2325 -> [_ w2333]
          tunnel: [i16 0 w2332] -> w2319
          frame False {
          }
          frame True {
            n833 = Add(x=w2334, y=w2333) -> (x+y=w2332:i32)
          }
        }
        n834 = case shown="True" w2322 {
          tunnel: w2324 -> [_ w2330]
          tunnel: w2323 -> [_ w2329]
          tunnel: [i16 0 w2328] -> w2316
          frame False {
          }
          frame True {
            n835 = Add(x=w2330, y=w2329) -> (x+y=w2328:i32)
          }
        }
        n836 = Greater?(x=w2319, y=w2318) -> (0:w2320:bool)
        n837 = Greater?(x=w2316, y=w2318) -> (0:w2317:bool)
        n838 = Select(t=w2318, s=w2317, f=w2316) -> (s? t:f=w2313:i32)
        n839 = Select(t=w2318, s=w2320, f=w2319) -> (s? t:f=w2314:i32)
        n840 = Greater?(x=w2314, y=w2309) -> (0:w2310:bool)
        n841 = Greater?(x=w2313, y=w2309) -> (0:w2315:bool)
        n842 = Select(t=w2313, s=w2315, f=w2309) -> (s? t:f=w2311:i32)
        n843 = Select(t=w2314, s=w2310, f=w2309) -> (s? t:f=w2312:i32)
      }
    }
    n844 = case shown="True" w1191 {
      selector: w1191 -> [_ w2268]
      tunnel: [w2265 w2267] -> w1240
      tunnel: [w2264 i16 0] -> w1241
      tunnel: w1286 -> [w2265 _]
      tunnel: w1287 -> [w2264 _]
      frame False {
      }
      frame True {
        n845 = Not(x=w2268) -> (.not. x?=w2267:bool)
      }
    }
    "Move Respond - R" <- w1240
    "deltaMoveServo\n- R" <- w1241
    n846 = case shown="False" w1251 {
      selector: w1251 -> [_ w2295]
      tunnel: [w2292 w2294] -> w1243
      tunnel: [w2291 i16 0] -> w1246
      tunnel: w1282 -> [w2292 _]
      tunnel: w1283 -> [w2291 _]
      frame False {
      }
      frame True {
        n847 = Not(x=w2295) -> (.not. x?=w2294:bool)
      }
    }
    "Move Respond - L" <- w1243
    "deltaMoveServo\n- L" <- w1246
    "Current Main State - Left" <- w1274
    "Frames Processed\nCount - in -L" <- w1266
    "Recovery Mode Count - in Left" <- w1261
    "Recovery Search\nmove Count - in - L" <- w1260
    "Recovery Search\nAttempt Count - in - L" <- w1259
    "Current Main State - Right" <- w1221
    "Frames Processed\nCount - in Right" <- w1204
    "Recovery Search\nmove Count - Right" <- w1206
    "Recovery Search\nAttempt Count - Right" <- w1205
    "Recovery Mode Count in Right" <- w1197
    "Tracking Timeout\nCount - L" <- w1238
    "Tracking Timeout\nCount - R" <- w1213
    "Current Tracking State - Left" <- w1237
    "Current Tracking State - Right 2" <- w1219
    "Current Recovery State - Right" <- w1220
    "Current Recovery State -L" <- w1234
  }
